vi "Oxford-1820-Main.vi"() -> ()   [LabVIEW 2016]
uses:
  <instrlib>/Mercury iXX/Mercury iXX.lvlib
  <instrlib>/Mercury iXX/Public/Controls/Comms Transport Layer.ctl
  <instrlib>/Mercury iXX/Public/Libraries/Pressure/Open/Open Pressure Device.vi
  <instrlib>/Mercury iXX/Public/Libraries/Pressure.lvlib
  <instrlib>/Mercury iXX/Public/Libraries/Pressure/Configuration/Read/Pressure Device (Read).vi
  <instrlib>/Mercury iXX/Public/Libraries/System/Read/Display Automatic Dimming (Read).vi
  <instrlib>/Mercury iXX/Public/Libraries/System.lvlib
  <instrlib>/Mercury iXX/Public/Libraries/System/Read/Display Automatic Dimming Time (Read).vi
  <instrlib>/Mercury iXX/Public/Libraries/System/Read/Display Brightness (Read).vi
  <instrlib>/Mercury iXX/Public/Libraries/System/Read/Mode (Read).vi
  <instrlib>/Mercury iXX/Public/Libraries/System/Read/Serial Number (Read).vi
  <instrlib>/Mercury iXX/Public/Libraries/System/Read/FVer (Read).vi
  <instrlib>/Mercury iXX/Public/Libraries/System/Read/HVer (Read).vi
  <instrlib>/Mercury iXX/Public/Libraries/System/Set/DateTime (Set).vi
  <instrlib>/Mercury iXX/Public/Libraries/Temperature/Signals/Read/Temperature (Read).vi
  <instrlib>/Mercury iXX/Public/Libraries/Temperature.lvlib
  <instrlib>/Mercury iXX/Public/Libraries/Temperature/Configuration/Read/Calibration Cold Limit (Read).vi
  <instrlib>/Mercury iXX/Public/Libraries/Temperature/Configuration/Read/Calibration Hot Limit (Read).vi
  <instrlib>/Mercury iXX/Public/Libraries/Temperature/Configuration/Read/Excitation Type (Read).vi
  <instrlib>/Mercury iXX/Public/Libraries/Temperature/Configuration/Read/Temperature Sensor (Read).vi
  <instrlib>/Mercury iXX/Public/Libraries/Temperature/Configuration/Read/Temperature Device (Read).vi
  <instrlib>/Mercury iXX/Public/Libraries/Temperature/Configuration/Read/Nickname (Read).vi
  <instrlib>/Mercury iXX/Public/Libraries/Temperature/Configuration/Read/Excitation Magnitude (Read).vi
  <instrlib>/Mercury iXX/Public/Libraries/Temperature/Configuration/Read/Serial Number (Read).vi
  <instrlib>/Mercury iXX/Public/Libraries/System/Read/Catalogue (Read).vi
  <instrlib>/Mercury iXX/Public/Libraries/System/Read/Flash Space (Read).vi
  <instrlib>/Mercury iXX/Public/Libraries/System/Read/DateTime (Read).vi
  <instrlib>/Mercury iXX/Public/Libraries/System/Read/Time (Read).vi
  <instrlib>/Mercury iXX/Public/Libraries/System/Read/Date (Read).vi
  <instrlib>/Mercury iXX/Public/Libraries/System/Open/Open System.vi
  <instrlib>/Mercury iXX/Public/Libraries/Temperature/Open/Open Temperature Device.vi
  <instrlib>/Mercury iXX/Public/Libraries/Auxiliary/Open/Open Auxiliary Device.vi
  <instrlib>/Mercury iXX/Public/Libraries/Auxiliary.lvlib
  <instrlib>/Mercury iXX/Public/Libraries/Auxiliary/Signals/Read/Percent Open (Read).vi
  <instrlib>/Mercury iXX/Public/Libraries/Magnet/Open/Open Magnet Device.vi
  <instrlib>/Mercury iXX/Public/Libraries/Magnet.lvlib
  <instrlib>/Mercury iXX/Public/Libraries/Magnet/Configuration/Read/PSU Action Status (Read).vi
  <instrlib>/Mercury iXX/Public/Libraries/Magnet/Configuration/Read/Magnet Device (Read).vi
  <instrlib>/Mercury iXX/Public/Libraries/Temperature/Signals/Read/Voltage (Read).vi
  <instrlib>/Mercury iXX/Private/Controls/Query Dynamic Reference.ctl
  <instrlib>/Mercury iXX/Public/Controls/Mercury Reference.ctl
  <instrlib>/Mercury iXX/Public/Libraries/Level Meter/Open/Open Level Meter Device.vi
  <instrlib>/Mercury iXX/Public/Libraries/Level Meter.lvlib
  <instrlib>/Mercury iXX/Public/Libraries/Level Meter/Signals/Read/Probe Level Nitrogen (Read).vi
  <instrlib>/Mercury iXX/Public/Libraries/Level Meter/Signals/Read/Probe Level Helium (Read).vi
  <instrlib>/Mercury iXX/Public/Libraries/Magnet/Signals/Read/Switch Heater Status (Read).vi
  <instrlib>/Mercury iXX/Public/Libraries/Magnet/Signals/Read/Current (Read).vi
  <instrlib>/Mercury iXX/Public/Libraries/Magnet/Configuration/Set/PSU Action Status (Set).vi
  <instrlib>/Mercury iXX/Public/Libraries/Magnet/Controls/PSU Actions.ctl
  <instrlib>/Mercury iXX/Public/Libraries/Magnet/Controls/Switch Heater.ctl
  SMOs/Instrument.Oxford1820/Instrument.Oxford1820.lvclass
  <instrlib>/Mercury iXX/Public/Libraries/Lambda/Configuration/Set/Lambda Percentage Flow (Set).vi
  <instrlib>/Mercury iXX/Public/Libraries/Lambda.lvlib
  <instrlib>/Mercury iXX/Public/Libraries/Lambda/Open/Open Lambda Device.vi
  <instrlib>/Mercury iXX/Public/Controls/Response String.ctl
  <instrlib>/Mercury iXX/Public/Libraries/Temperature/Signals/Read/Resistance (Read).vi
  <instrlib>/Mercury iXX/Public/Libraries/Temperature/Configuration/Set/Excitation Magnitude (Set).vi
  <instrlib>/Mercury iXX/Public/Libraries/Magnet/Signals/Read/Voltage (Read).vi
  SMOs/Instrument.Oxford1820/Typedefs/Status.ctl
  SMOs/Instrument.Oxford1820/Typedefs/Actions.ctl
  <instrlib>/Mercury iXX/Public/Libraries/System/Controls/User Mode.ctl
  <instrlib>/Mercury iXX/Public/Libraries/System/Set/Mode (Set).vi
  <instrlib>/Mercury iXX/Public/Libraries/Heater/Signals/Read/Power (Read).vi
  <instrlib>/Mercury iXX/Public/Libraries/Heater.lvlib
  <instrlib>/Mercury iXX/Public/Libraries/Heater/Signals/Read/Current (Read).vi
  <instrlib>/Mercury iXX/Public/Libraries/Auxiliary/Signals/Read/Position (Read).vi
  <instrlib>/Mercury iXX/Public/Libraries/Level Meter/Signals/Read/Probe Count Nitrogen (Read).vi
  <instrlib>/Mercury iXX/Public/Libraries/Magnet/Signals/Read/Current Rate (Read).vi
  <userlib>/_OpenG.lib/error/error.llb/Filter Error Codes (Array)__ogtk.vi
  <instrlib>/Mercury iXX/Public/Libraries/Heater/Configuration/Read/Nickname (Read).vi
  <instrlib>/Mercury iXX/Public/Libraries/Heater/Configuration/Read/Voltage Limit (Read).vi
  <instrlib>/Mercury iXX/Public/Libraries/Heater/Configuration/Read/Serial Number (Read).vi
  <instrlib>/Mercury iXX/Public/Libraries/Heater/Configuration/Read/Heater Device (Read).vi
  <instrlib>/Mercury iXX/Public/Libraries/Heater/Open/Open Heater Device.vi
  <instrlib>/Mercury iXX/Public/Libraries/Heater/Signals/Read/Voltage (Read).vi
  <instrlib>/Mercury iXX/Public/Libraries/Heater/Configuration/Read/Maximum Power (Read).vi
  <instrlib>/Mercury iXX/Public/Libraries/Heater/Configuration/Read/Nominal Resistance (Read).vi
  <instrlib>/Mercury iXX/Public/Libraries/Auxiliary/Configuration/Read/Stepper Speed (Read).vi
  <instrlib>/Mercury iXX/Public/Libraries/Auxiliary/Configuration/Read/Valve Gearing (Read).vi
  <instrlib>/Mercury iXX/Public/Libraries/Auxiliary/Configuration/Read/Temperature Error Voltage Sensitivity (Read).vi
  <instrlib>/Mercury iXX/Public/Libraries/Auxiliary/Configuration/Read/Temperature Error Sensitivity (Read).vi
  <instrlib>/Mercury iXX/Public/Libraries/Auxiliary/Configuration/Read/Gas Flow Scaling (Read).vi
  <instrlib>/Mercury iXX/Public/Libraries/Auxiliary/Configuration/Read/Minimum Gas Flow (Read).vi
  <instrlib>/Mercury iXX/Public/Libraries/Auxiliary/Configuration/Read/Serial Number (Read).vi
  <instrlib>/Mercury iXX/Public/Libraries/Auxiliary/Configuration/Read/Aux Device (Read).vi
  <instrlib>/Mercury iXX/Public/Libraries/Pressure/Signals/Read/Voltage (Read).vi
  <instrlib>/Mercury iXX/Public/Libraries/Pressure/Signals/Read/Current (Read).vi
  <instrlib>/Mercury iXX/Public/Libraries/Pressure/Configuration/Read/Nickname (Read).vi
  <instrlib>/Mercury iXX/Public/Libraries/Level Meter/Signals/Read/Probe Resistance Helium (Read).vi
  <instrlib>/Mercury iXX/Public/Libraries/Level Meter/Configuration/Read/Nitrogen Pulse Count Period (Read).vi
  <instrlib>/Mercury iXX/Public/Libraries/Level Meter/Configuration/Read/Nitrogen Freq at 100 (Read).vi
  <instrlib>/Mercury iXX/Public/Libraries/Level Meter/Configuration/Read/Helium Pulse Duration (Read).vi
  <instrlib>/Mercury iXX/Public/Libraries/Level Meter/Configuration/Read/Helium Pulse Mag (Read).vi
  <instrlib>/Mercury iXX/Public/Libraries/Level Meter/Configuration/Read/Helium Probe Resistance (Read).vi
  <instrlib>/Mercury iXX/Public/Libraries/Level Meter/Configuration/Read/Serial Number (Read).vi
  <instrlib>/Mercury iXX/Public/Libraries/Level Meter/Configuration/Read/Level Meter Device (Read).vi
  <instrlib>/Mercury iXX/Public/Libraries/Magnet/Configuration/Read/Software Voltage Limit (Read).vi
  <instrlib>/Mercury iXX/Public/Libraries/Magnet/Configuration/Read/Switch Present (Read).vi
  <instrlib>/Mercury iXX/Public/Libraries/Magnet/Configuration/Read/Current to Field Factor (Read).vi
  <instrlib>/Mercury iXX/Public/Libraries/Magnet/Configuration/Read/Current Limit (Read).vi
  <instrlib>/Mercury iXX/Public/Libraries/Magnet/Configuration/Read/Output Configuration (Read).vi
  <instrlib>/Mercury iXX/Public/Libraries/Magnet/Configuration/Read/Bipolar Output (Read).vi
  <instrlib>/Mercury iXX/Public/Libraries/Magnet/Configuration/Read/Serial Number (Read).vi
  <instrlib>/Mercury iXX/Public/Libraries/Magnet/Signals/Read/Target Field (Read).vi
  <instrlib>/Mercury iXX/Public/Libraries/Magnet/Signals/Read/Target Field Rate (Read).vi
  <instrlib>/Mercury iXX/Public/Libraries/Magnet/Signals/Read/Field (Read).vi
  <instrlib>/Mercury iXX/Public/Libraries/Magnet/Signals/Read/Persistant Field (Read).vi
  <instrlib>/Mercury iXX/Public/Libraries/Magnet/Configuration/Set/Switch Heater Current (Set).vi
  <instrlib>/Mercury iXX/Public/Libraries/Magnet/Signals/Read/Persistant Current (Read).vi
  <instrlib>/Mercury iXX/Public/Libraries/Magnet/Signals/Set/Switch Heater No Check (Set).vi
  <instrlib>/Mercury iXX/Public/Libraries/Magnet/Signals/Set/Target Field (Set).vi
  <instrlib>/Mercury iXX/Public/Libraries/Magnet/Signals/Set/Target Field Rate (Set).vi
  <instrlib>/Mercury iXX/Public/Libraries/Lambda/Configuration/Set/Lambda Flow Auto (Set).vi
  <instrlib>/Mercury iXX/Public/Libraries/Level Meter/Configuration/Set/Pulse Slow-Fast (Set).vi
  <instrlib>/Mercury iXX/Public/Libraries/Temperature/Controls/Excitation Type.ctl
  <instrlib>/Mercury iXX/Public/Controls/Manufacturing Data.ctl
  <instrlib>/Mercury iXX/Public/Libraries/Temperature/Controls/Excitation Cluster.ctl
  <instrlib>/Mercury iXX/Public/Libraries/Temperature/Controls/Calibration Interpolation.ctl
  <instrlib>/Mercury iXX/Public/Libraries/Temperature/Controls/Calibration Cluster.ctl
  <instrlib>/Mercury iXX/Public/Controls/Unit String.ctl
  <instrlib>/Mercury iXX/Public/Libraries/Heater/Controls/Heater Signals Cluster.ctl
  <instrlib>/Mercury iXX/Public/Libraries/Heater/Controls/Heater Device (Read).ctl
  <instrlib>/Mercury iXX/Public/Libraries/Level Meter/Controls/Resistance Configuration.ctl
  <instrlib>/Mercury iXX/Public/Libraries/Level Meter/Controls/Pre-Pulse.ctl
  <instrlib>/Mercury iXX/Public/Libraries/Level Meter/Controls/Pulse.ctl
  <instrlib>/Mercury iXX/Public/Libraries/Level Meter/Controls/Helium Configuration.ctl
  <instrlib>/Mercury iXX/Public/Libraries/Level Meter/Controls/Frequency Configuration.ctl
  <instrlib>/Mercury iXX/Public/Libraries/Level Meter/Controls/Nitrogen Configuration.ctl
  <instrlib>/Mercury iXX/Public/Libraries/Level Meter/Controls/Signals.ctl
  <instrlib>/Mercury iXX/Public/Libraries/Level Meter/Controls/Level Meter (Read).ctl
  <instrlib>/Mercury iXX/Public/Libraries/Auxiliary/Controls/AUX Signals (Read).ctl
  <instrlib>/Mercury iXX/Public/Libraries/Auxiliary/Controls/AUX Device (Read).ctl
  <instrlib>/Mercury iXX/Public/Libraries/Magnet/Controls/Signals (Read).ctl
  <instrlib>/Mercury iXX/Public/Libraries/Magnet/Controls/Device (Read).ctl
  <instrlib>/Mercury iXX/Public/Libraries/Magnet/Controls/Identifier.ctl
  <instrlib>/Mercury iXX/Public/Libraries/Pressure/Controls/Pressure Signals Cluster.ctl
panel:
  out "LPF ON":timestamp
  in  "Tab Control":T1(tab)
  in  "Enable RS232 Panel":bool
  out "LEDs":bool[](array[boolean])
  out "Iteration Time":dbl
  in  "Percentage Open":dbl=100.0 format="%#_13g"
  out "PS Heat on or off (sec)":dbl format="%<%H:%M:%S>t"
  out "LPF on (min)":dbl=5373.0 format="%<%H:%M:%S>t"
  out "Magnet Status 2":string
  in  "OK":bool
  out "LPF Resistance":dbl=4.2075 format="%_3f ohms"
  out "Magnet Resistance":dbl=3.8705 format="%_3f ohms"
  out "ETA":timestamp format="%<%I:%M:%S %p\n%m/%d/%y>T"
  in  "Open Needle Valve":bool
  in  "Close Needle Valve":bool
  in  "Lambda":bool
  out "LPF Pressure":dbl format="%_5f mB"
  out "LPF Needle Valve (%)":dbl format="%_6g"
  out "LPF Temperature":dbl=4.2075 format="%_2f K"
  out "Magnet Temperature":dbl=3.8705 format="%_2f K"
  out "He LVL Chart":dbl(slide)=52.0833 scale=0.0..100.0
  out "N2 LVL Chart":dbl(slide)=61.3025 scale=0.0..100.0
  in  "Remote Mode":bool
  out "Power Supply Field (T)":dbl=0.0001 format="%#.5f"
  out "Magnet Field (T)":dbl format="%.5f"
  out "Voltage (V)":dbl=-0.0003 format="%.5f"
  out "Current (A)":dbl=0.0006 format="%.5f"
  out "N2 LEVEL":dbl=61.3025 format="%.0f %"
  out "He LEVEL":dbl=52.0833 format="%.0f %"
  in  "Fast/Slow Fill":bool
  out "Magnet Field (T)":dbl(knob) caption="Voltage (V)" scale=-20.0..20.0
  out "SWITCH HEATER":bool
  in  "PS Heat":bool
  in  "Clamp":bool
  in  "To Set":bool
  in  "To Zero":bool
  in  "Hold":bool
  out "Magnet Status":string="Clamped"
  out "Target Field Rate (T/min)":dbl=1.0 format="%.5f"
  out "Target Field (T)":dbl format="%#.5f"
  in  "Target Rate (T/min)":dbl=0.1 format="%.5f"
  in  "Target Field (T)":dbl format="%#.5f"
  in  "Send to IPS":bool
  out "Voltage (V)":dbl(knob)=-0.0003 scale=-10.0..10.0
  out "Current (A)":dbl(knob)=0.0006 scale=-180.0..180.0
  in  "Mercury Functions":T2(tab)=enum."ITC: Temperature"
  out "time stamp":timestamp=timestamp(3543841780 s since 1904-01-01)
  out "Free Space":i32=166384 caption="Free Space (KB)"
  out "Set Date Response":string="VALID"
  out "String":string="NORM" caption="User Mode"
  out "Date":string="2016:04:18"
  out "Time":string="11:29:40"
  out "Hardware Version":string="65"
  out "Firmware Version":string="2.2.6.20"
  out "Serial Number":string="154650110"
  out "ITC Devices":string[](array[string])=["DB4.G1:AUX", "DB8.P1:PRES", "MB0.H1:HTR", "MB1.T1:TEMP"]
  out "S/W Version(s)":string[](array[string])=["2.2.6.20\n"]
  out "Serial Number(s)":string[](array[string])=["154650110"]
  out "# of Instruments":i32=1
  out "Automatic Dimming":string="OFF"
  out "Dimming Time":string="5"
  out "Display Brightness":string="100"
  in  "ITC IP Address":string="130.49.180.101"
  out "Excitation Magnitude":dbl=5.0
  out "Sensor Type":string="NTC"
  out "Excitation Type":string="UNIP"
  out "Hot Limit":dbl=1000.0
  out "H Unit":T3="K"
  out "Cold Limit":dbl=1000.0
  out "C Unit":T3="K"
  out "Unit":T3
  out "Voltage":dbl=0.005
  out "V Unit":T3="V"
  out "Temperature":dbl=4.2075
  out "T Unit":T3="K"
  out "Temp S/N":string="154650110"
  out "T Nickname":string="Mag_AB_MB1"
  out "ITC Calibration":T4
  out "ITC Excitation":T6
  out "ITC Manufacturing":T8
  out "Heater Device Settings":T9={"Manufacturing"={"Hardware Version"="65", "Firmware Version"="2.3", "Serial Number"="154650110"}, "Nickname"="MB0.H1", "Voltage Limit"="1", "Nominal Resistance"="10", "Maximum Power"="0.1000", "Heater Signals"={"Voltage"="0.0507V", "Current"="-0.0000A", "Power"="0.0000W"}, "Status"="2"}
  out "Htr C Unit":T3="A"
  out "Htr P Unit":T3="W"
  out "Htr V Unit":T3="V"
  out "Htr Current":dbl=-0.0
  out "Htr Power":dbl
  out "Htr Voltage":dbl=0.0507
  out "Power Unit":T3
  out "Volt Unit":T3
  out "Res Unit":T3
  out "Maximum Power":dbl=0.1
  out "Htr Resistance":dbl=10.0
  out "Htr Voltage Limit":dbl=1.0
  out "Htr S/N":string="154650110"
  out "Htr Nickname":string="MB0.H1"
  out "Nickname":string="Lam_P_DB8"
  out "Current":dbl=-0.0
  out "Voltage":dbl=-8.219999999999999e-05
  out "Manufacturing":T8
  out "Pressure Signals":T11
  out "Auxiliary Device Details":T12={"Manufacturing"={"Hardware Version"="65", "Firmware Version"="3.1", "Serial Number"="154650084"}, "Min Flow"=0.0, "Scaling Factor"=50.0, "Temp Err"=9.0, "Temp V Err"=11.0, "Gear"=2, "Speed"=2, "Signals"={"Position"=0.0, "% Open"=0.0, "I0"="ON", "I1"="OFF", "I2"="OFF", "I3"="OFF", "O0"="OFF", "O1"="OFF", "O2"="OFF", "O3"="OFF"}, "Nickname"="DB4.G1", "Status"="0"} {"Signals"."% Open" min=0.0 max=100.0 step=0.1 format="%.4f"; "Signals"."Position" max=20.0 step=1.0 format="%.4f"; "Speed" max=7 step=1; "Gear" max=7 step=1; "Temp V Err" min=0.0 max=20.0 step=0.1; "Temp Err" min=0.0 max=20.0 step=0.1; "Scaling Factor" min=0.0 max=99.0 step=0.1; "Min Flow" min=0.0 max=20.0 step=0.1}
  out "Aux S/N":string="154650084"
  out "Min Flow":dbl caption="Minimum Gas Flow" format="%#.1f"
  out "Scaling Factor":dbl=50.0 caption="Gas Flow Scaling Factor" format="%#.1f"
  out "Temp Err":dbl=9.0 caption="Temperature Error Sensitivity" format="%#.1f"
  out "Temp V Err":dbl=11.0 caption="Temperature Voltage Error Sensitivity" format="%#.1f"
  out "Gear":u32=2 caption="Valve Gearing"
  out "Speed":u32=2 caption="Stepper Speed"
  out "Unit 2":T3
  out "Unit 3":T3
  out "Unit 4":T3
  out "Unit 5":T3
  out "Unit 6":T3
  out "Unit 7":T3
  out "Position":u32
  out "% Open":dbl caption="Percentage Open (%)"
  out "Unit":T3
  out "Unit":T3="%"
  out "time stamp 2":timestamp=timestamp(3543841781 s since 1904-01-01)
  out "Free Space 2":i32=166316 caption="Free Space (KB)"
  out "Set Date Response 2":string="VALID"
  out "String 2":string="NORM" caption="User Mode"
  out "Date 2":string="2016:04:18"
  out "Time 2":string="11:29:45"
  out "Hardware Version 2":string="65"
  out "Firmware Version 2":string="2.2.6.20"
  out "Serial Number 2":string="153350063"
  out "IPS Devices":string[](array[string])=["DB3.L1:LVL", "GRPX:PSU", "GRPY:PSU", "GRPZ:PSU", "MB1.T1:TEMP", "PSU.M1:PSU", "PSU.M2:PSU", "PSU.M3:PSU"]
  out "S/W Version(s) 2":string[](array[string])=["2.2.6.20\n"]
  out "Serial Number(s) 2":string[](array[string])=["153350063"]
  out "# of Instruments 2":i32=1
  out "Automatic Dimming 2":string="OFF"
  out "Dimming Time 2":string="5"
  out "Display Brightness 2":string="100"
  in  "IPS IP Address":string="130.49.180.102"
  out "LVL Device DetailSettings":T14={"Manufacturing"={"Hardware Version"="65", "Firmware Version"="2.2", "Serial Number"="152450013"}, "Nitrogen Configuration"={"Frequency Configuration"={"Freq 0%"=0.0, "Freq 100%"=0.0}, "Pulse Period"=0.0}, "Signals"={"Helium Signals"={"Resistance"=75.5626, "Level"=52.0833}, "Nitrogen Signals"={"Count"=8800.0, "Freq"=487361.0, "Level"=61.3445}}, "Nickname"="DB3.L1", "Status"="0", "Helium Configuration"={"Resistance Configuration"={"Res 0%"=0.0, "Res 100%"=0.0}, "Pre-Pulse"={"Magnitude"=0.0, "Duration"=0.0}, "Pulse"={"Magnitude"=0.0, "Duration"=0.0, "Delay"=0.0}}}
  out "LVL S/N":string="152450013"
  out "LVL P Magnitude":dbl=125.0 caption="Pulse Magnitude (mA)"
  out "LVL P Duration":dbl=5.0 caption="Pulse Duration (s)"
  out "N Freq 100%":dbl=7880.0 caption="Frequency at 100% (Hz)"
  out "N Pulse Period":dbl=1000.0 caption="Pulse Period (ms)"
  out "He Res Config":T19={"Res 0%"=149.0, "Res 100%"=8.0}
  out "He Resistance":dbl=75.5626 caption="Resistance (Ohms)"
  out "He Level":dbl=52.0833 caption="Helium Level (%)"
  out "N Counter":u32 caption="Counter"
  out "N Level":dbl=61.3445 caption="Nitrogen Level (%)"
  out "Excitation Magnitude 2":dbl=5.0
  out "Sensor Type 2":string="NTC"
  out "Excitation Type 2":string="UNIP"
  out "Hot Limit 2":dbl=1000.0
  out "H Unit 2":T3="K"
  out "Cold Limit 2":dbl=1000.0
  out "C Unit 2":T3="K"
  out "Unit 12":T3
  out "Voltage 2":dbl=0.005
  out "V Unit 2":T3="V"
  out "Temperature 2":dbl=3.8706
  out "T Unit 2":T3="K"
  out "Temp S/N 2":string="153350063"
  out "T Nickname 2":string="MB1.T1"
  out "IPS Calibration":T4
  out "IPS Excitation":T6
  out "IPS Manufacturing":T8
  out "Magnet Device Details":T22={"Manufacturing"={"Hardware Version"="NOT_FOUND", "Firmware Version"="NOT_FOUND", "Serial Number"="NOT_FOUND"}, "Nickname"="GRPZ", "Bipolar Output"="ON", "String"="PARA", "Current Limit"=174.0, "AtoB"=8.688, "Inductance"=39.406, "Switch Present"="PSU.M1", "Swh Htr Current"=86.0, "SW VLIM"=9.0, "V Trans Time"=1000.0, "Magnet PSU Signals"={"Voltage"=-0.0002, "Current"=0.0002, "Current Rate"=100.0, "Field"=0.0001, "Field Rate"=11.5101, "Persistant Current"=0.0003, "Persistant Field"=0.0, "Target Current"=0.0, "Target Field"=0.0, "Target Current Rate"=8.688, "Target Field Rate"=1.0, "Switch Heater Status (SWHT)"="OFF", "Switch Heater Status (SWHN)"="OFF"}, "PSU Action"="CLMP", "Status"="40000000", "Level Limit"=0.0, "Temperature Limit"=999.0} {"Temperature Limit" format="%#.1f"; "Level Limit" format="%#.1f"; "V Trans Time" format="%#.1f"; "SW VLIM" format="%#.1f"; "Swh Htr Current" format="%#.1f"; "Inductance" format="%#.1f"; "AtoB" format="%#.1f"; "Current Limit" format="%#.1f"}
  out "Mag S/N":string="NOT_FOUND"
  out "Bipolar Output":string="ON"
  out "Out Config":string="PARA" caption="Output Configuration"
  out "Current Limit":dbl=174.0 caption="Current Limit (A)" format="%#.1f"
  out "AtoB":dbl=8.688 caption="Current Field Factor (A/T)" format="%#.1f"
  out "Switch Present":string="PSU.M1"
  out "SW VLIM":dbl=9.0 caption="Software Voltage Limit (V)" format="%#.1f"
  out "Unit 8":T3
  out "Unit 9":T3
  out "Unit 10":T3
  out "Current Rate":dbl=100.0
  out "PSU Act Stat":string="CLMP" caption="PSU Action Status"
  out "Unit 11":T3="A/min"
  in  "Device Identifier":T24="GRPZ"
  out "M3 Voltage":dbl
  out "M3 Current":dbl
  out "M2 Voltage":dbl
  out "M2 Current":dbl
  out "M1 Voltage":dbl
  out "M1 Current":dbl
  out "Error List":T25(array[cluster])
  out "PS ON/OFF":timestamp format="%<%I:%M:%S %p>T"
  in  "Heater Current":bool
  in  "Swh Htr Current (mA)":dbl=90.0 format="%#_13g"
  # "v2017/10/10"
  # "Voltage (V)"
  # "Magnet (T)"
  # "Current (A)"
  # "Slow Rates\nCurrent Range (A)     Field Range (T)    Rate (T/min)\n0       -- 100        0    -- 11.5       0.91\n100     -- 150        11.5 -- 17.2       0.23\n150     -- 155.467    17.2 -- 18         0.11\n155.567 -- 172.471    18   -- 20         0.11"
  # "Fast Rates\nCurrent Range (A)     Field Range (T)    Rate (T/min)\n0       -- 155.467    0    -- 18         1.0\n155.567 -- 172.471    18   -- 20         0.25"
  # "ITC: 101\nIPS: 102\nIPS VR: 67"
  # "ITC: 101\nIPS: 102\nIPS VR: 67"
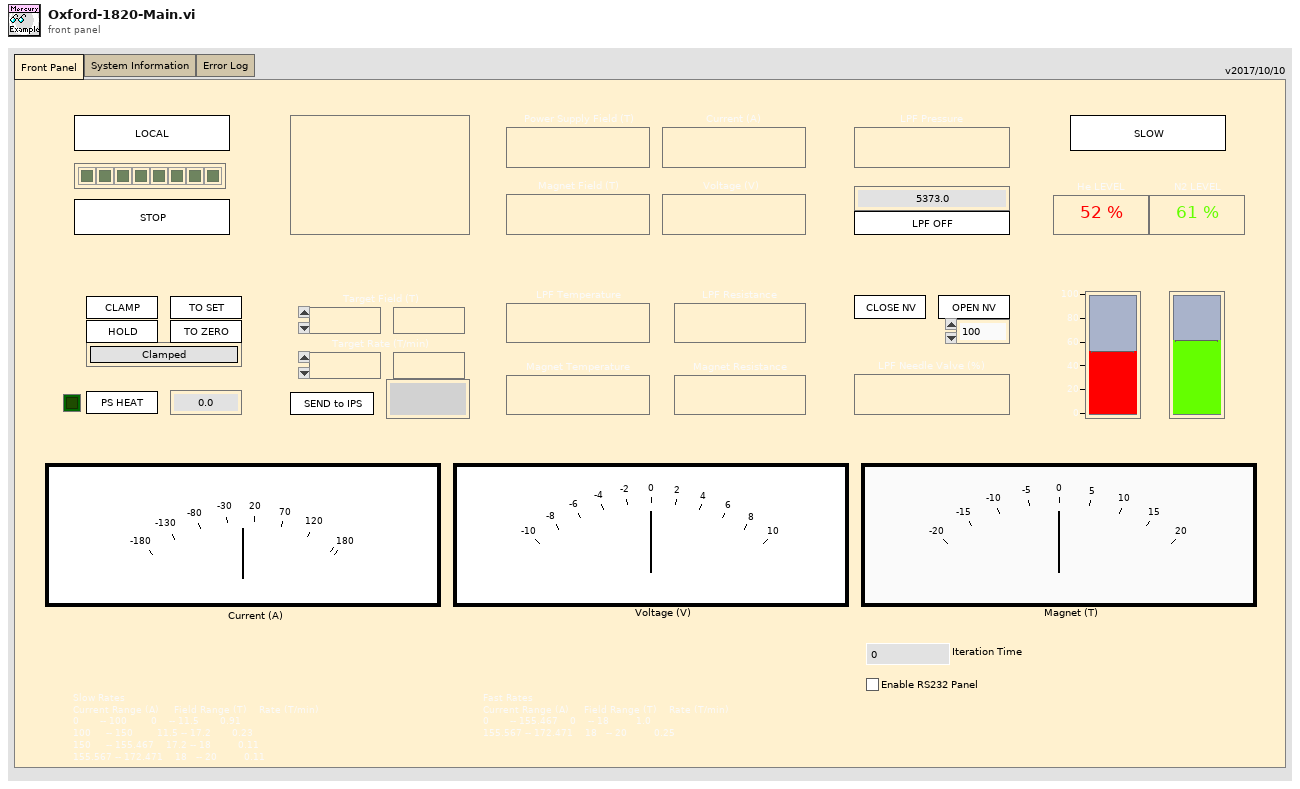
[diagram p1: front panel]
types:
  T1 = enum32{"Front Panel", "System Information", "Error Log"}
  T2 = enum32{"ITC: System", "ITC: Temperature", "ITC: Heater", "ITC: Pressure", "ITC: Auxiliary", "IPS: System", "IPS: Level Meter", "IPS: Temperature", "IPS: Magnet"}
  T3 = typedef "Mercury iXX.lvlib/Unit String.ctl" = string
  T4 = typedef "Mercury iXX.lvlib/Temperature.lvlib/Calibration Cluster.ctl" = cluster{"Filename":string, "Interpolation":T5, "Scaling Factor":string, "Offset Factor":string, "Hot Limit":string, "Cold Limit":string, "Last Calibration":string, "Reference":string}
  T5 = typedef "Mercury iXX.lvlib/Temperature.lvlib/Calibration Interpolation.ctl" = string
  T6 = typedef "Mercury iXX.lvlib/Temperature.lvlib/Excitation Cluster.ctl" = cluster{"Excitation Type":T7, "Magnitude":string}
  T7 = typedef "Mercury iXX.lvlib/Temperature.lvlib/Excitation Type.ctl" = string
  T8 = typedef "Mercury iXX.lvlib/Manufacturing Data.ctl" = cluster{"Hardware Version":string, "Firmware Version":string, "Serial Number":string}
  T9 = typedef "Mercury iXX.lvlib/Heater.lvlib/Heater Device (Read).ctl" = cluster{"Manufacturing":T8, "Nickname":string, "Voltage Limit":string, "Nominal Resistance":string, "Maximum Power":string, "Heater Signals":T10, "Status":string}
  T10 = typedef "Mercury iXX.lvlib/Heater.lvlib/Heater Signals Cluster.ctl" = cluster{"Voltage":string, "Current":string, "Power":string}
  T11 = typedef "Mercury iXX.lvlib/Pressure.lvlib/Pressure Signals Cluster.ctl" = cluster{"Voltage":string, "Current":string, "Power":string, "Pressure":string}
  T12 = typedef "Mercury iXX.lvlib/Auxiliary.lvlib/AUX Device (Read).ctl" = cluster{"Manufacturing":T8, "Min Flow":dbl, "Scaling Factor":dbl, "Temp Err":dbl, "Temp V Err":dbl, "Gear":u32, "Speed":u32, "Signals":T13, "Nickname":string, "Status":string}
  T13 = typedef "Mercury iXX.lvlib/Auxiliary.lvlib/AUX Signals (Read).ctl" = cluster{"Position":dbl, "% Open":dbl, "I0":string, "I1":string, "I2":string, "I3":string, "O0":string, "O1":string, "O2":string, "O3":string}
  T14 = typedef "Mercury iXX.lvlib/Level Meter.lvlib/Level Meter (Read).ctl" = cluster{"Manufacturing":T8, "Nitrogen Configuration":T15, "Signals":T17, "Nickname":string, "Status":string, "Helium Configuration":T18}
  T15 = typedef "Mercury iXX.lvlib/Level Meter.lvlib/Nitrogen Configuration.ctl" = cluster{"Frequency Configuration":T16, "Pulse Period":dbl}
  T16 = typedef "Mercury iXX.lvlib/Level Meter.lvlib/Frequency Configuration.ctl" = cluster{"Freq 0%":dbl, "Freq 100%":dbl}
  T17 = typedef "Mercury iXX.lvlib/Level Meter.lvlib/Signals.ctl" = cluster{"Helium Signals":cluster{"Resistance":dbl, "Level":dbl}, "Nitrogen Signals":cluster{"Count":dbl, "Freq":dbl, "Level":dbl}}
  T18 = typedef "Mercury iXX.lvlib/Level Meter.lvlib/Helium Configuration.ctl" = cluster{"Resistance Configuration":T19, "Pre-Pulse":T20, "Pulse":T21}
  T19 = typedef "Mercury iXX.lvlib/Level Meter.lvlib/Resistance Configuration.ctl" = cluster{"Res 0%":dbl, "Res 100%":dbl}
  T20 = typedef "Mercury iXX.lvlib/Level Meter.lvlib/Pre-Pulse.ctl" = cluster{"Magnitude":dbl, "Duration":dbl}
  T21 = typedef "Mercury iXX.lvlib/Level Meter.lvlib/Pulse.ctl" = cluster{"Magnitude":dbl, "Duration":dbl, "Delay":dbl}
  T22 = typedef "Mercury iXX.lvlib/Magnet.lvlib/Device (Read).ctl" = cluster{"Manufacturing":T8, "Nickname":string, "Bipolar Output":string, "String":string, "Current Limit":dbl, "AtoB":dbl, "Inductance":dbl, "Switch Present":string, "Swh Htr Current":dbl, "SW VLIM":dbl, "V Trans Time":dbl, "Magnet PSU Signals":T23, "PSU Action":string, "Status":string, "Level Limit":dbl, "Temperature Limit":dbl}
  T23 = typedef "Mercury iXX.lvlib/Magnet.lvlib/Signals (Read).ctl" = cluster{"Voltage":dbl, "Current":dbl, "Current Rate":dbl, "Field":dbl, "Field Rate":dbl, "Persistant Current":dbl, "Persistant Field":dbl, "Target Current":dbl, "Target Field":dbl, "Target Current Rate":dbl, "Target Field Rate":dbl, "Switch Heater Status (SWHT)":string, "Switch Heater Status (SWHN)":string}
  T24 = typedef "Mercury iXX.lvlib/Magnet.lvlib/Identifier.ctl" = string
  T25 = cluster{"time":timestamp, "code":i32, "source":string}[]
  T26 = enum32{"invalid app kind", "Development System", "Run Time System", "Student Edition", "Embedded LabVIEW", "Evaluation", "Custom"}
  T27 = cluster{"time":timestamp, "code":i32, "source":string}
  T28 = enum32{"Invalid", "Standard", "Closed", "Hidden", "Minimized", "Maximized"}
  T29 = typedef "Instrument.Oxford1820.lvclass/Status.ctl" = cluster{"Magnet Field":dbl, "PS Field":dbl, "Target Field":dbl, "Target Field Rate":dbl, "Voltage":dbl, "Current":dbl, "Switch":bool, "Mercury State":string}
  T30 = cluster{"Magnet Field":dbl, "PS Field":dbl, "Target Field":dbl, "Target Field Rate":dbl, "Voltage":dbl, "Current":dbl}
  T31 = typedef "Instrument.Oxford1820.lvclass/Actions.ctl" = cluster{"Hold":bool, "Clamp":bool, "To Set":bool, "To Zero":bool, "Send to IPS":bool, "PS Heat":bool, "Lambda":bool}
  T32 = typedef "Mercury iXX.lvlib/System.lvlib/User Mode.ctl" = string
  T33 = typedef "Mercury iXX.lvlib/Magnet.lvlib/Switch Heater.ctl" = string
  T34 = typedef "Mercury iXX.lvlib/Response String.ctl" = string
  T35 = typedef "Mercury iXX.lvlib/Mercury Reference.ctl" = cluster{"Comms":refnum<visa-resource-name>, "Device ID":string[], "Comms Layer":T36, "Command":string, "Query reference":T37}
  T36 = typedef "Mercury iXX.lvlib/Comms Transport Layer.ctl" = enum16{"Ethernet TCP/IP", "USB", "ISOBus - RS-232", "GPIB"}
  T37 = typedef "Mercury iXX.lvlib/Query Dynamic Reference.ctl" = refnum<vi>
  T38 = cluster{"Core":cluster{"Current VI Reference":refnum<vi>, "Close Panel on Exit?":bool}, "Mercury ITC Ref":T35, "Mercury IPS Ref":T35, "sentinel":bool, "Error Log":cluster{"time":timestamp, "code":i32, "source":string}[], "read ITC T?":bool, "counter":i32, "LEDs":bool[]}
  T39 = typedef "Filtered Error Details - Cluster__ogtk.ctl" = cluster{"code":i32, "source":string}
  T40 = cluster{"Current VI Reference":refnum<vi>, "Close Panel on Exit?":bool}
  T41 = typedef "Mercury iXX.lvlib/Temperature.lvlib/Temperature Sensor Type.ctl" = string
  T42 = typedef "Mercury iXX.lvlib/Temperature.lvlib/Temperature Device (Read).ctl" = cluster{"Manufacturing":T8, "Temperature Sensor Type":T41, "Excitation":T6, "Calibration":T4, "Control Loop":T43, "Temperature Signals":T44, "Nickname":string, "Status":string}
  T43 = typedef "Mercury iXX.lvlib/Temperature.lvlib/Loop Cluster.ctl" = cluster{"Heater":string, "Auxiliary":string, "Heater Auto":string, "Percentage Heat":string, "Temperature Set Point":string, "PID Auto (from file)":string, "P Value":string, "I Value":string, "D Value":string, "Auto PID Table Filename":string, "Flow Auto":string, "Target Heater Table":string, "Sweep mode":string, "Sweep Table Filename":string, "Percentage Flow":string}
  T44 = typedef "Mercury iXX.lvlib/Temperature.lvlib/Temperature Signals Cluster.ctl" = cluster{"Voltage":string, "Current":string, "Power":string, "Resistance":string, "Temperature":string, "Sensitivity":string, "Reference":string}
  T45 = typedef "Mercury iXX.lvlib/Pressure.lvlib/Pressure Device (Read).ctl" = cluster{"Manufacturing":T8, "Temperature Sensor Type":T46, "Calibration":T47, "Control Loop":T49, "Pressure Signals":T11, "Nickname":string, "Status":string}
  T46 = typedef "Mercury iXX.lvlib/Pressure.lvlib/Pressure Sensor Type.ctl" = string
  T47 = typedef "Mercury iXX.lvlib/Pressure.lvlib/Calibration Cluster.ctl" = cluster{"Filename":string, "Interpolation":T48, "Scaling Factor":string, "Offset Factor":string, "High Limit":string, "Low Limit":string, "Last Calibration":string}
  T48 = typedef "Mercury iXX.lvlib/Pressure.lvlib/Calibration Interpolation.ctl" = string
  T49 = typedef "Mercury iXX.lvlib/Pressure.lvlib/Loop Cluster.ctl" = cluster{"Heater":string, "Auxiliary":string, "Heater Auto":string, "Percentage Heat":string, "Pressure Set Point":string, "PID Auto (from file)":string, "P Value":string, "I Value":string, "D Value":string, "Auto PID Table Filename":string, "Flow Auto":string, "Target Heater Table":string, "Sweep mode":string, "Sweep Table Filename":string, "Percentage Flow":string}
  T50 = typedef "Mercury iXX.lvlib/Magnet.lvlib/Output Configuration.ctl" = string
  T51 = typedef "Mercury iXX.lvlib/Magnet.lvlib/PSU Actions.ctl" = string
  T52 = typedef "Instrument.Oxford1820.lvclass/Targets.ctl" = cluster{"Field (T)":dbl, "Field Rate (T/min)":dbl}
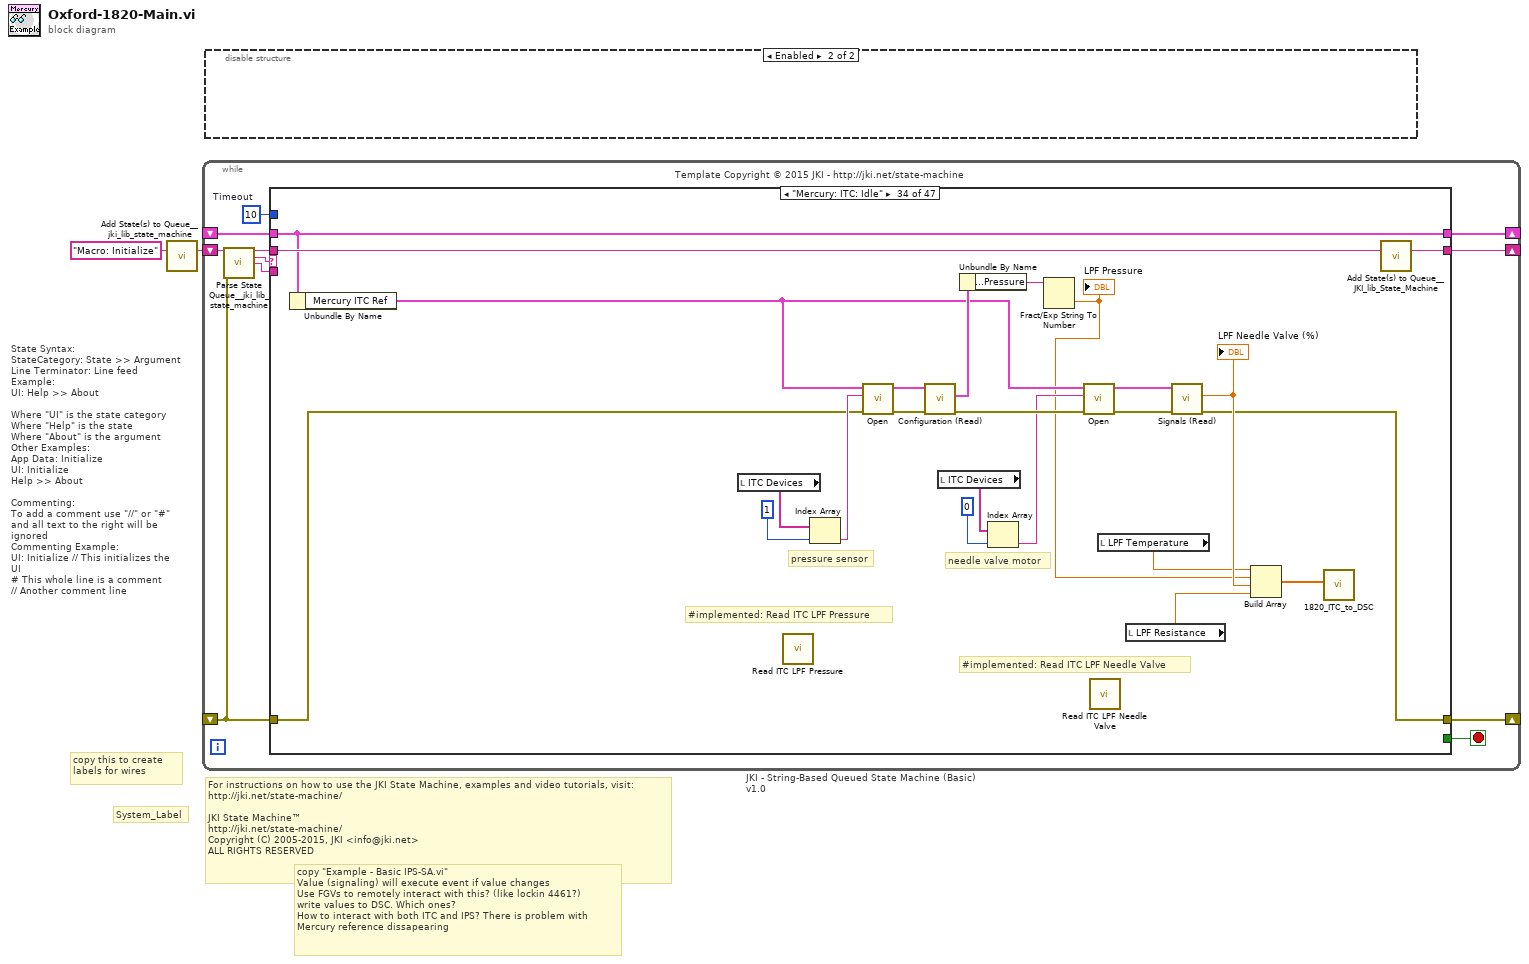
[diagram p0: block diagram]
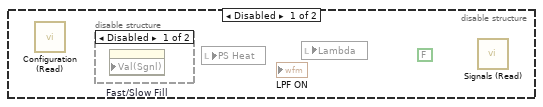
[diagram p2: hidden frame]
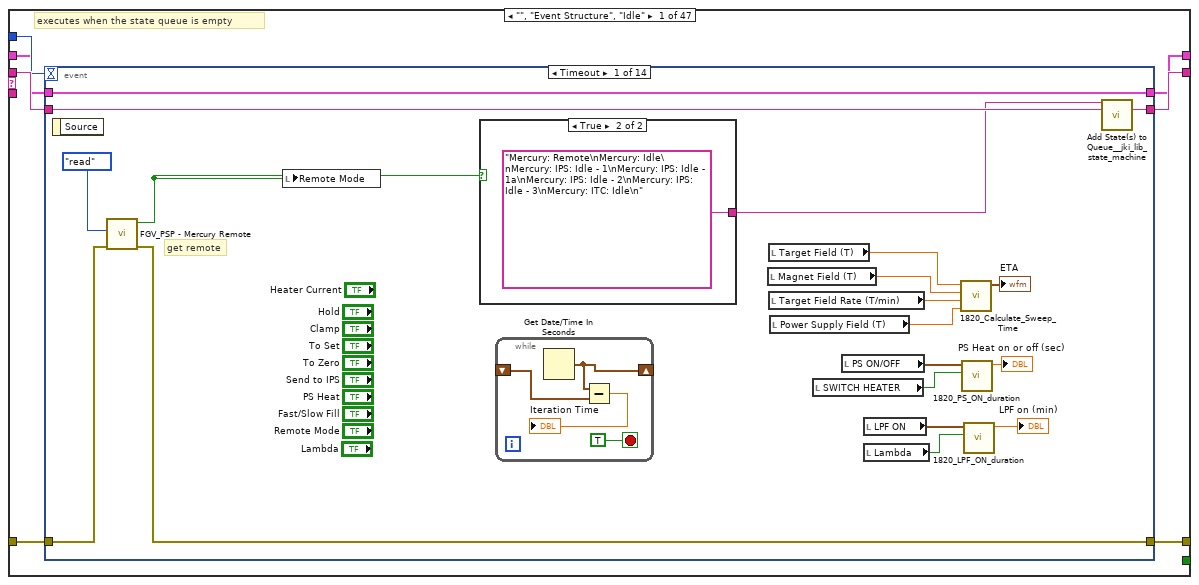
[diagram p4: hidden frame]
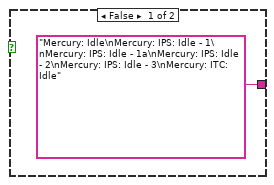
[diagram p5: hidden frame]
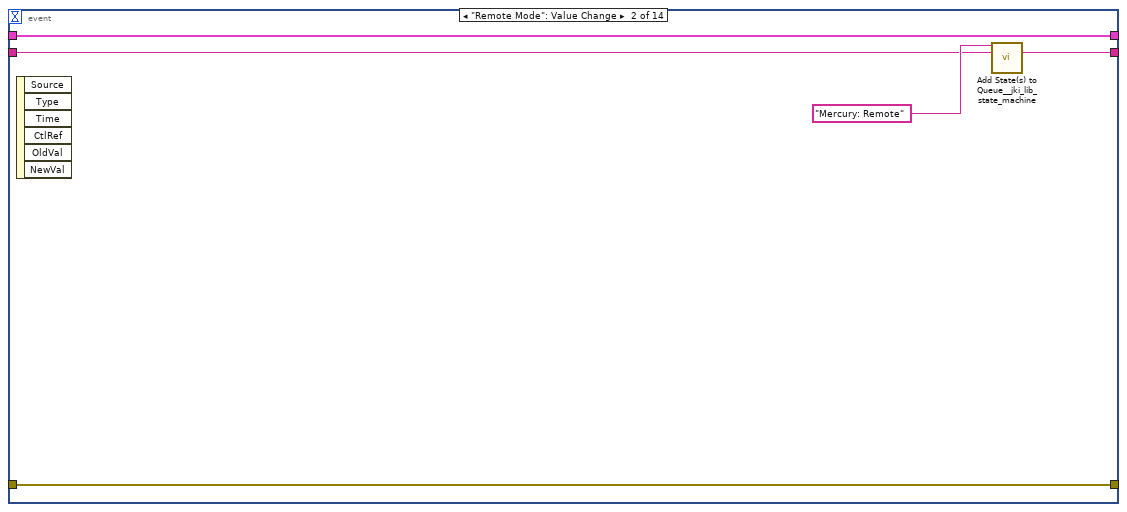
[diagram p6: hidden frame]
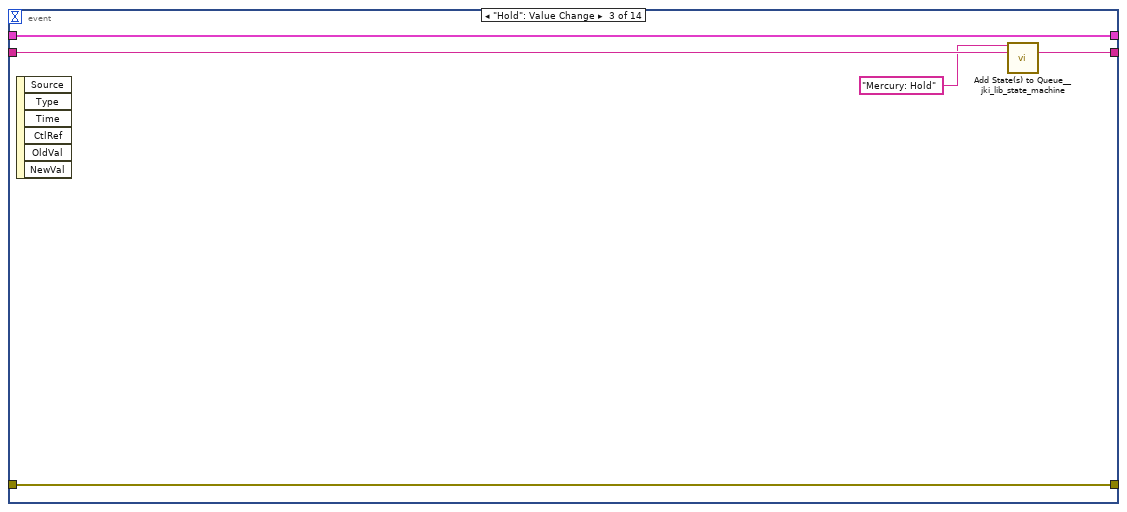
[diagram p7: hidden frame]
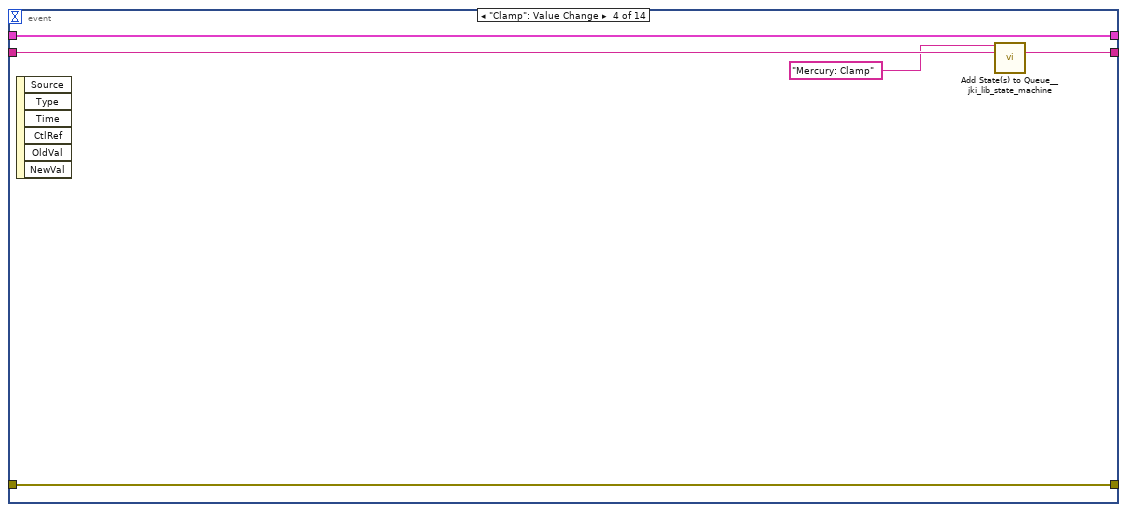
[diagram p8: hidden frame]
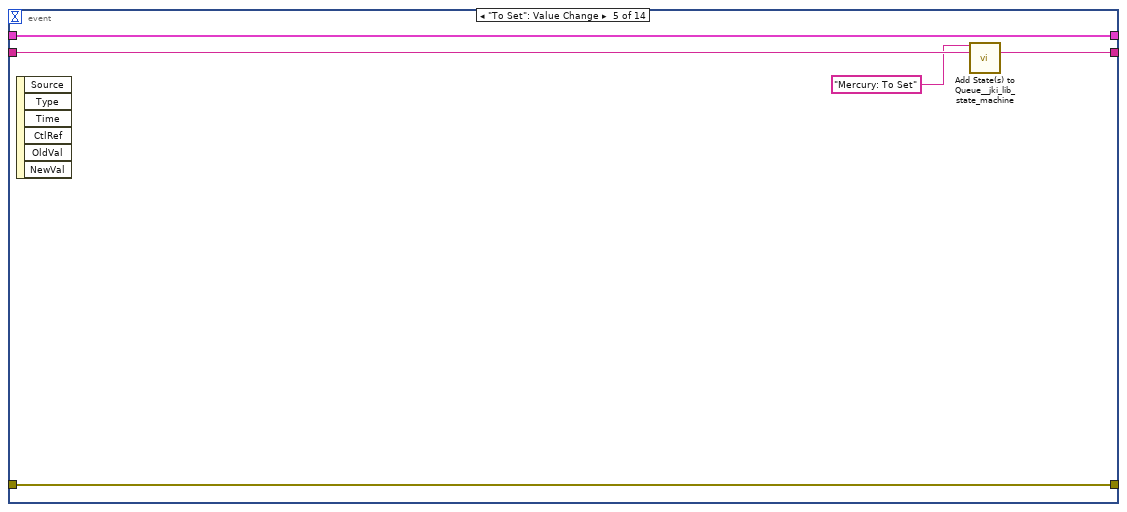
[diagram p9: hidden frame]
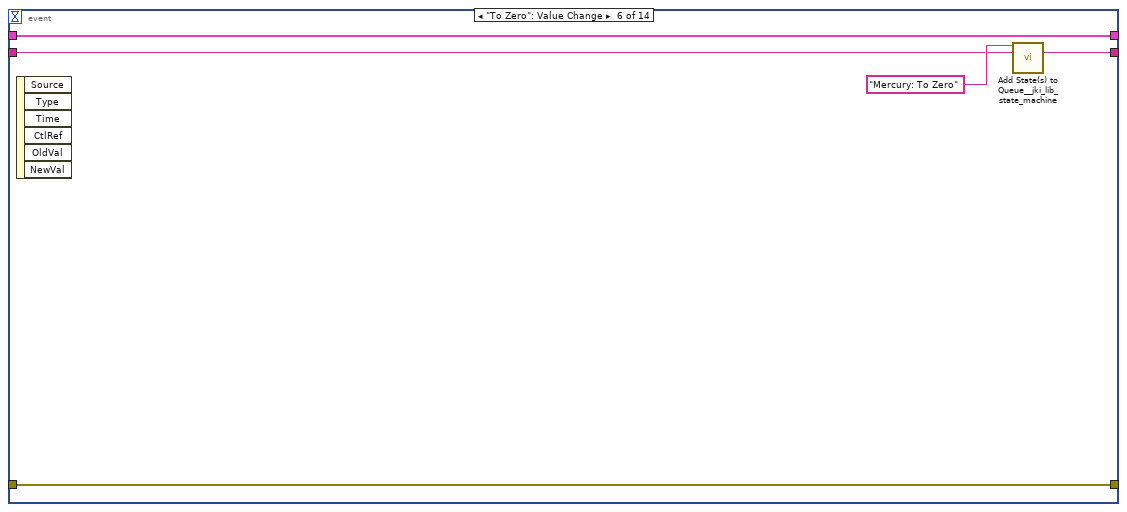
[diagram p10: hidden frame]
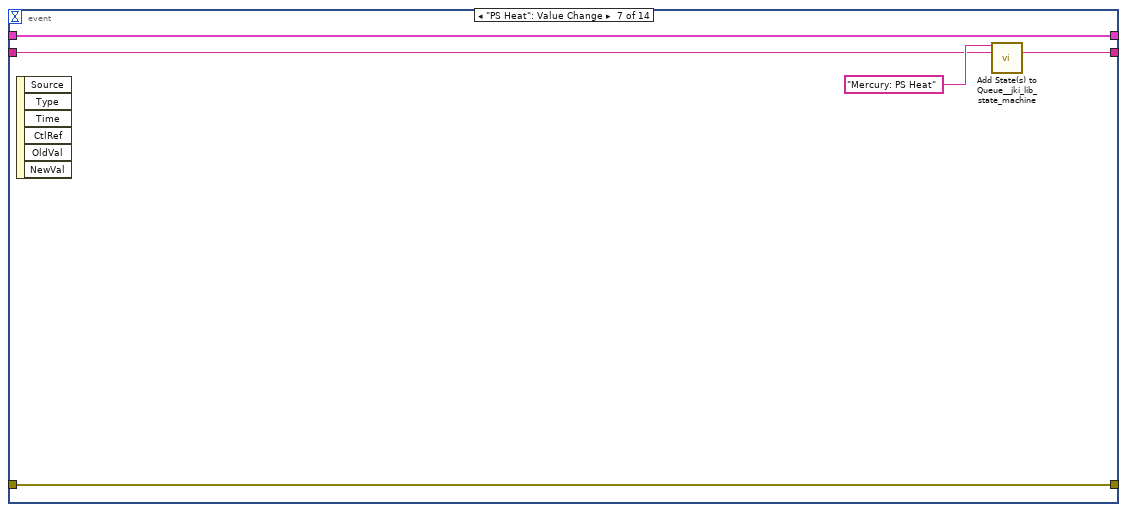
[diagram p11: hidden frame]
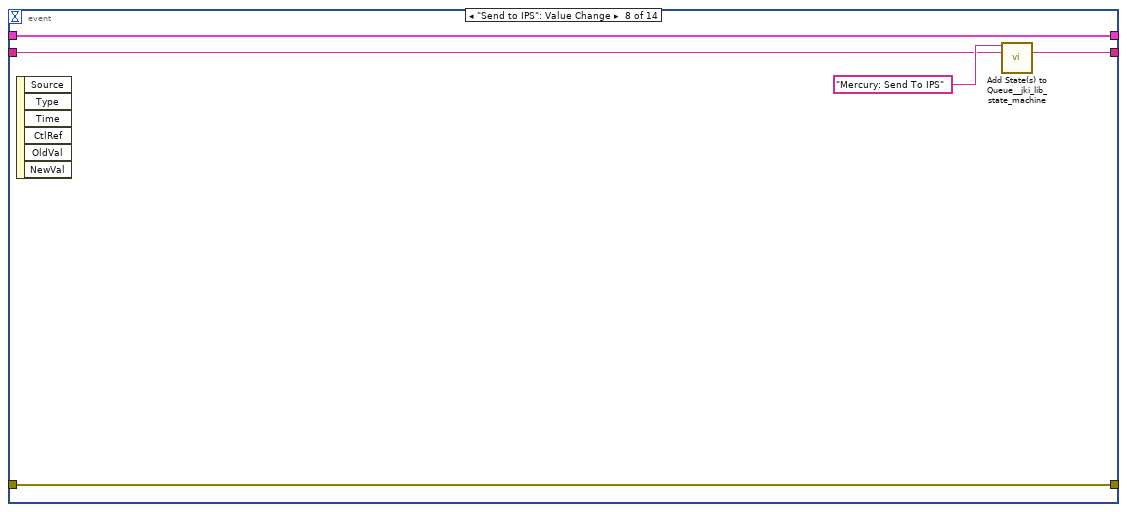
[diagram p12: hidden frame]
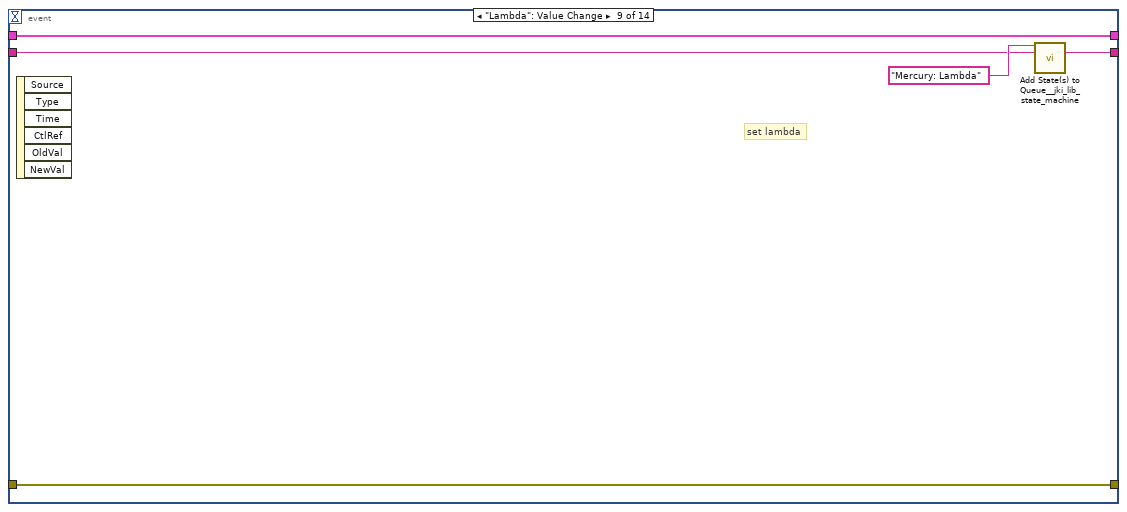
[diagram p13: hidden frame]
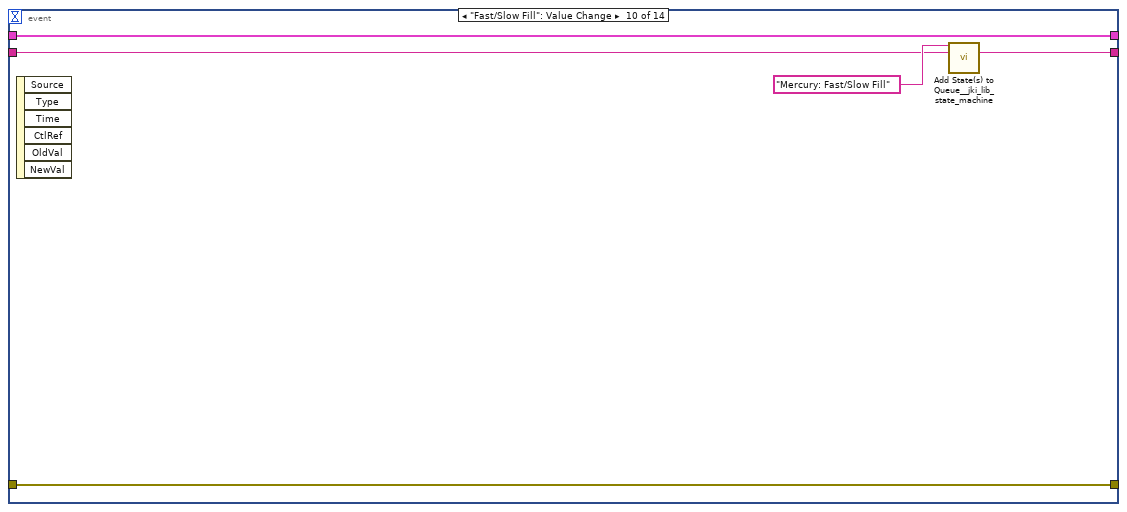
[diagram p14: hidden frame]
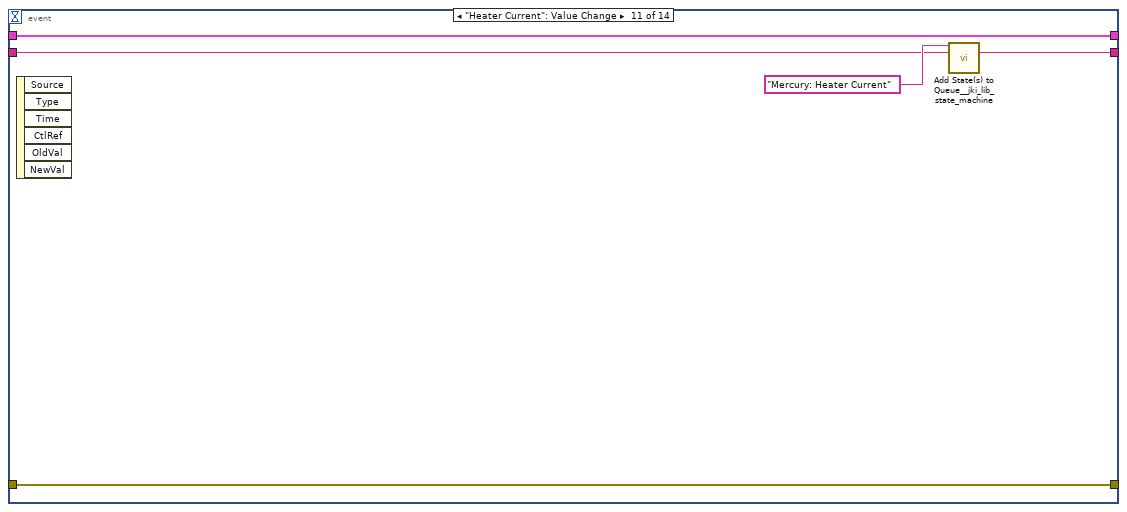
[diagram p15: hidden frame]
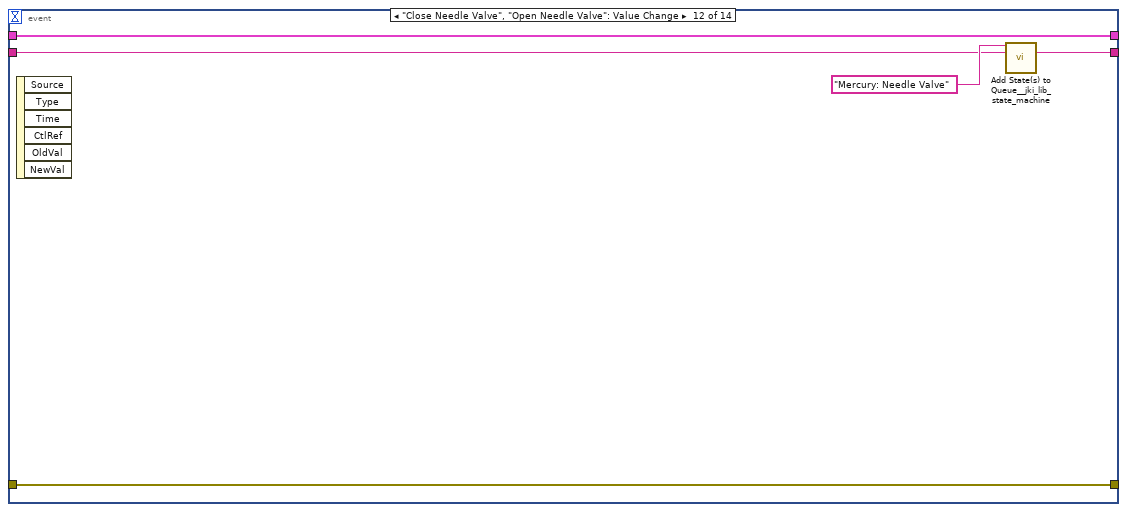
[diagram p16: hidden frame]
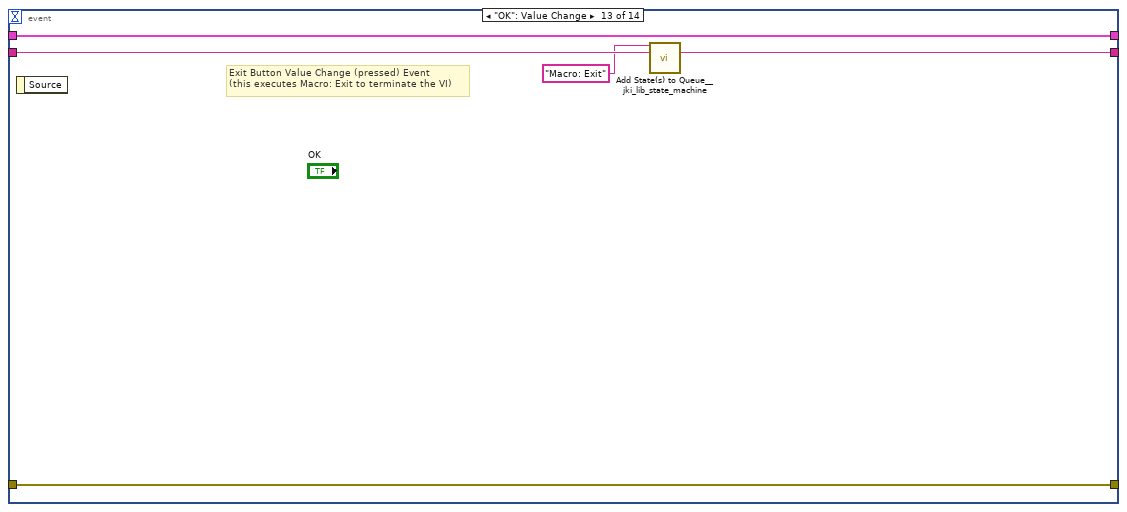
[diagram p17: hidden frame]
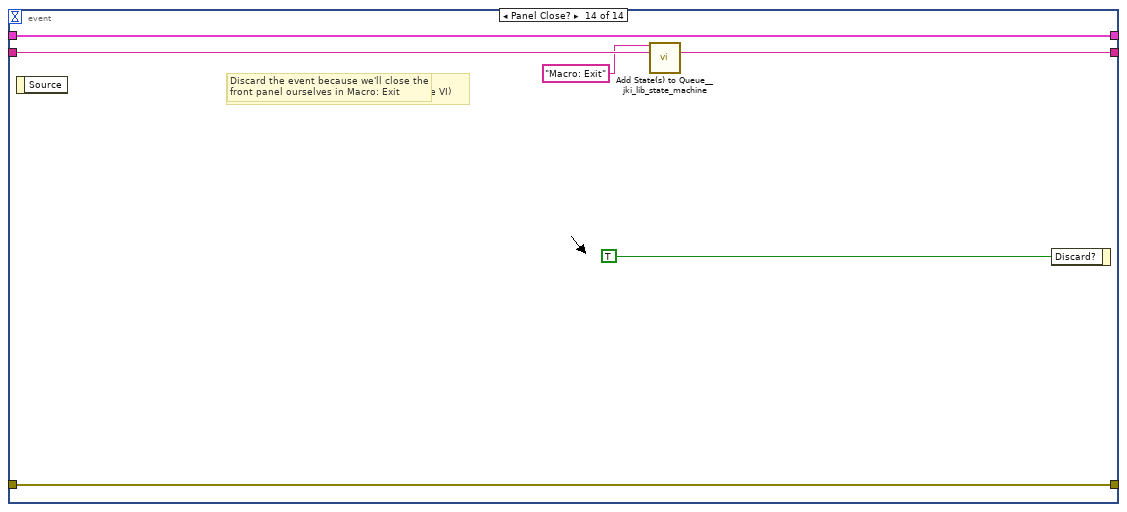
[diagram p18: hidden frame]
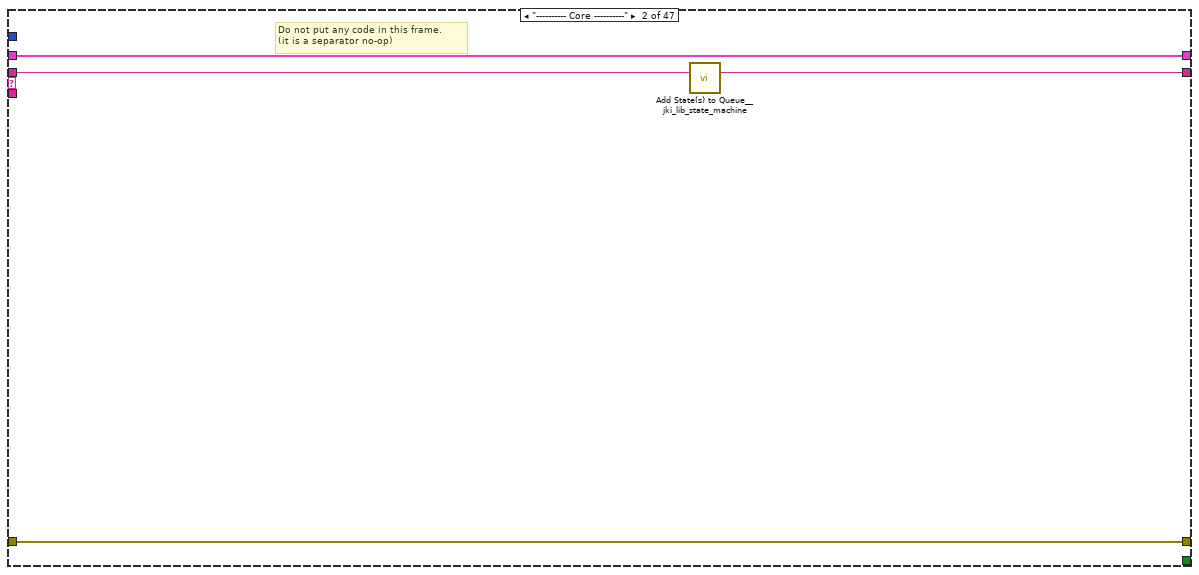
[diagram p19: hidden frame]
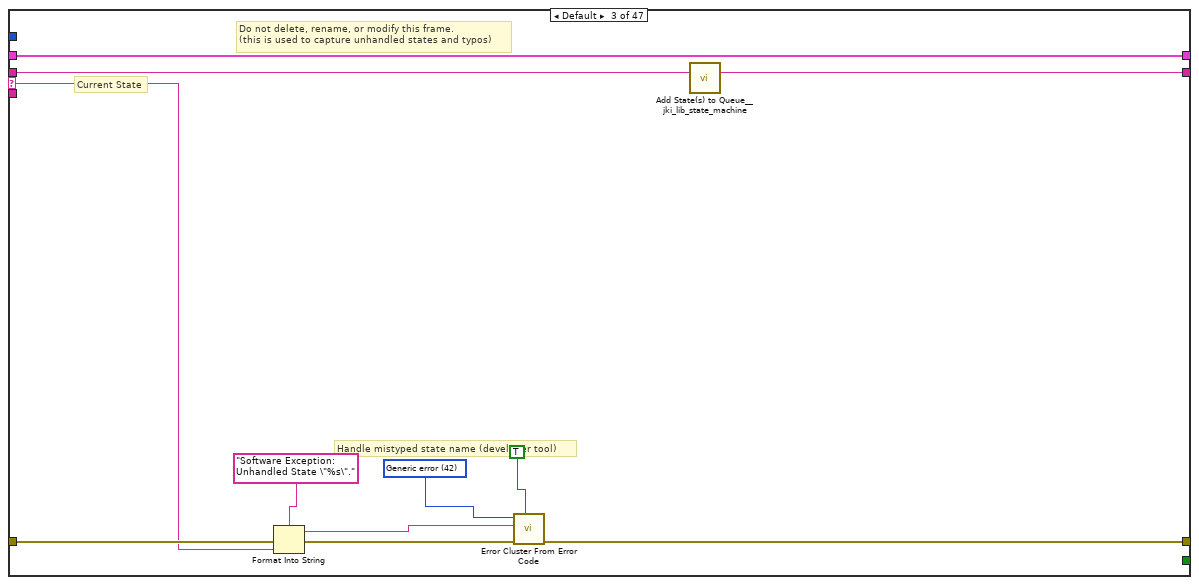
[diagram p20: hidden frame]
diagram:
  # "copy \"Example - Basic IPS-SA.vi\"\nValue (signaling) will execute event if value changes\nUse FGVs to remotely interact with this? (like lockin 4461?)\nwrite values to DSC. Which ones?\nHow to interact with both ITC and IPS? There is problem with \nMercury reference dissapearing"
  # "For instructions on how to use the JKI State Machine, examples and video tutorials, visit:\nhttp://jki.net/state-machine/\n\nJKI State Machine™\nhttp://jki.net/state-machine/\nCopyright (C) 2005-2015, JKI <info@jki.net>\nALL RIGHTS RESERVED"
  # "State Syntax:\nStateCategory: State >> Argument\nLine Terminator: Line feed\nExample:\nUI: Help >> About\n\nWhere \"UI\" is the state category\nWhere \"Help\" is the state\nWhere \"About\" is the argument\nOther Examples:\nApp Data: Initialize\nUI: Initialize\nHelp >> About\n\nCommenting:\nTo add a comment use \"//\" or \"#\" and all text to the right will be ignored\nCommenting Example:\nUI: Initialize // This initializes the UI\n# This whole line is a comment\n// Another comment line"
  # "copy this to create labels for wires"
  # "System_Label"
  n1 = call <vilib>:"Add State(s) to Queue__jki_lib_state_machine.vi"("State(s) in (\"\")"="Macro: Initialize") -> ("States Out"=w2:string)  [unwired: 14 in]
  n2 = while "JKI - String-Based Queued State Machine (Basic) v1.0" {
    shift-right: [w6] -> _
    shift-left: _ -> [w5]
    shift-right: [w9] -> _
    shift-left: _ -> [w3]
    shift-right: [w8] -> _
    shift-left: w2 -> [w10]
    stop <- w7 stop-if-true
    w4 = 10  # Timeout
    # "Template Copyright © 2015 JKI - http://jki.net/state-machine"
    n3 = call <vilib>:"Parse State Queue__jki_lib_state_machine.vi"("State Queue"=w10, "Error In (no error)"=w3) -> ("Remaining States"=w12:string, "Current State"=w13:string, "Arguments"=w11:string)  [unwired: 11 in]
    n4 = case shown="\"Mercury: ITC: Idle\"" w13 {
      selector: w13 -> [_ _ w116 _ _ _ _ _ _ _ _ _ _ _ _ _ _ _ _ _ _ _ _ _ _ _ _ _ _ _ _ _ _ _ _ _ _ _ _ _ _ _ _ _ _ _ _]
      tunnel: w12 -> [w20 w115 w120 w138 w155 w160 w164 w177 w183 w187 w197 w207 w218 w244 w251 w266 w270 w294 w343 w389 w431 w478 w501 w546 w587 w634 w675 w680 w702 w768 w805 w863 w879 w906 w910 w915 w958 w991 w1023 w1042 w1061 w1080 w1102 w1170 w1191 w1212 w1230]
      tunnel: w11 -> [_ _ _ _ _ _ _ _ _ _ _ w202 w212 _ _ _ _ _ _ _ _ _ _ _ _ _ _ _ _ _ _ _ _ _ _ _ _ _ _ _ _ _ _ _ _ _ _]
      tunnel: w5 -> [w16 w112 w118 w129 w141 w158 w161 _ w178 w184 w188 w205 w214 w241 w249 w264 w267 w289 w341 w388 w395 w438 w487 w544 w586 w633 w674 w677 w684 w736 w804 w820 w878 w905 w909 w912 w956 w981 w1018 w1032 w1051 w1070 w1088 w1155 w1181 w1197 w1218]
      tunnel: [w14 w113 w122 w135 errorcluster {"status"=FALSE, "code"=0, "source"=""} ("error out") w157 w162 w171 w179 w185 w192 w203 w215 w242 w248 w254 w268 w272 w303 w344 w392 w441 w488 w508 w553 w606 w641 w678 w687 w737 w776 w816 w876 w890 w908 w913 w924 w975 w1000 w1027 w1045 w1064 w1089 w1148 w1175 w1199 w1217] -> w9
      tunnel: [w19 w114 w119 w137 w154 w159 w163 w176 w182 w186 w196 w206 w217 w243 w250 w265 w269 w293 w342 w390 w432 w479 w502 w545 w588 w635 w676 w679 w703 w769 w806 w864 w880 w907 w911 w914 w959 w992 w1024 w1043 w1062 w1081 w1103 w1171 w1192 w1213 w1231] -> w8
      tunnel: [_ _ _ _ _ TRUE _ _ _ _ _ _ _ _ _ _ _ _ _ _ _ _ _ _ _ _ _ _ _ _ _ _ _ _ _ _ _ _ _ _ _ _ _ _ _ _ _] -> w7
      tunnel: [w18 w112 w118 w136 w140 w158 w161 w175 w178 w184 w189 w205 w214 w241 w249 w264 w267 w288 w341 w388 w395 w438 w487 w544 w586 w633 w674 w677 w683 w736 w804 w820 w878 w905 w909 w912 w956 w981 w1018 w1032 w1051 w1070 w1088 w1155 w1181 w1197 w1218] -> w6
      tunnel: w4 -> [w17 _ _ _ _ _ _ _ _ _ _ _ _ _ _ _ _ _ _ _ _ _ _ _ _ _ _ _ _ _ _ _ _ _ _ _ _ _ _ _ _ _ _ _ _ _ _]
      tunnel: w3 -> [w15 w113 w121 w135 w150 w157 w162 w171 w180 w185 w194 w204 w216 w242 w248 w256 w268 w281 w305 w355 w398 w440 w482 w510 w555 w593 w636 w678 w699 w767 w802 w853 w877 w884 w908 w913 w953 w986 w1015 w1037 w1056 w1075 w1090 w1165 w1182 w1200 w1216]
      frame "", "Event Structure", "Idle" {
        # "executes when the state queue is empty"
        n5 = event shown="[0] Timeout" {
          selector: _ -> [_ _ _ _ _ _ _ _ _ _ _ _ _ _]
          dyn-events: _ -> [_ _ _ _ _ _ _ _ _ _ _ _ _ _]
          timeout: w17 -> [_ _ _ _ _ _ _ _ _ _ _ _ _ _]
          tunnel: w20 -> [w39 w49 w55 w60 w64 w69 w74 w78 w84 w88 w93 w97 w105 w111]
          tunnel: [w38 w48 w54 w59 w63 w68 w73 w77 w83 w87 w92 w96 w104 w110] -> w19
          tunnel: [w21 w47 w51 w56 w61 w66 w71 w76 w81 w90 w95 w100 w102 w108] -> w18
          tunnel: w16 -> [w21 w47 w51 w56 w61 w66 w71 w76 w81 w90 w95 w100 w102 w108]
          tunnel: w15 -> [w24 w46 w52 w58 w65 w67 w72 w80 w82 w86 w91 w99 w103 w109]
          tunnel: [w23 w46 w52 w58 w65 w67 w72 w80 w82 w86 w91 w99 w103 w109] -> w14
          event Timeout {
            # "get remote"
            n6 = event-data() -> ()  [unwired: 1 in, 1 out]
            n7 = call "FGV_PSP - Mercury Remote.vi"("error in"=w24, "Function"=enum16{"write", "read"}."read") -> ("error out"=w23:errorcluster, "Remote"=w22:bool)  [unwired: 4 in]
            n8 = local write "Remote Mode"(w22) -> ()
            n9 = case shown="True" w22 {
              tunnel: ["Mercury: Idle\nMercury: IPS: Idle - 1\nMercury: IPS: Idle - 1a\nMercury: IPS: Idle - 2\nMercury: IPS: Idle - 3\nMercury: ITC: Idle" ("State(s) at Back (\"\")") "Mercury: Remote\nMercury: Idle\nMercury: IPS: Idle - 1\nMercury: IPS: Idle - 1a\nMercury: IPS: Idle - 2\nMercury: IPS: Idle - 3\nMercury: ITC: Idle\n" ("State(s) at Back (\"\")")] -> w27
              frame False {
              }
              frame True {
              }
            }
            n10 = while {
              shift-right: [w42] -> _
              shift-left: _ -> [w43]
              stop <- TRUE stop-if-true
              n11 = Get Date/Time In Seconds() -> (seconds since 1Jan1904=w42:timestamp)
              n12 = Subtract(x=w42, y=w43) -> (x-y=→"Iteration Time":dbl)
            }
            n13 = local read "Magnet Field (T)"() -> (w35:dbl)
            n14 = local read "Target Field (T)"() -> (w34:dbl)
            n15 = local read "Target Field Rate (T/min)"() -> (w37:dbl)
            n16 = local read "Power Supply Field (T)"() -> (w33:dbl)
            n17 = local read "SWITCH HEATER"() -> (w29:bool)
            n18 = local read "PS ON/OFF"() -> (w30:timestamp)
            n19 = local read "LPF ON"() -> (w32:timestamp)
            n20 = local read "Lambda"() -> (w26:bool)
            n21 = call "1820_Calculate_Sweep_Time.vi"("Power Supply Field (T)"=w33, "Target Field Rate (T/min)"=w37, "Magnet Field (T)"=w35, "Target Field (T)"=w34) -> ("ETA"=→"ETA":timestamp)  [unwired: 6 in, 1 out]
            n22 = call "1820_PS_ON_duration.vi"("SWITCH HEATER"=w29, "time stamp"=w30) -> ("PS Heat on (sec)"=→"PS Heat on or off (sec)":dbl)  [unwired: 9 in]
            n23 = call "1820_LPF_ON_duration.vi"("Lambda"=w26, "LPF ON"=w32) -> ("LPF on (min)"=→"LPF on (min)":dbl)  [unwired: 9 in]
            n24 = call <vilib>:"Add State(s) to Queue__jki_lib_state_machine.vi"("State(s) in Front (\"\")"=w27, "State(s) in (\"\")"=w39) -> ("States Out"=w38:string)  [unwired: 13 in]
          }
          event "Remote Mode": Value Change {
            n25 = event-data() -> ()  [unwired: 1 in, 6 out]
            n26 = call <vilib>:"Add State(s) to Queue__jki_lib_state_machine.vi"("State(s) in Front (\"\")"="Mercury: Remote", "State(s) in (\"\")"=w49) -> ("States Out"=w48:string)  [unwired: 13 in]
          }
          event "Hold": Value Change {
            n27 = event-data() -> ()  [unwired: 1 in, 6 out]
            n28 = call <vilib>:"Add State(s) to Queue__jki_lib_state_machine.vi"("State(s) in Front (\"\")"="Mercury: Hold" ("State(s) in Front (\"\")"), "State(s) in (\"\")"=w55) -> ("States Out"=w54:string)  [unwired: 13 in]
          }
          event "Clamp": Value Change {
            n29 = event-data() -> ()  [unwired: 1 in, 6 out]
            n30 = call <vilib>:"Add State(s) to Queue__jki_lib_state_machine.vi"("State(s) in Front (\"\")"="Mercury: Clamp" ("State(s) in Front (\"\")"), "State(s) in (\"\")"=w60) -> ("States Out"=w59:string)  [unwired: 13 in]
          }
          event "To Set": Value Change {
            n31 = event-data() -> ()  [unwired: 1 in, 6 out]
            n32 = call <vilib>:"Add State(s) to Queue__jki_lib_state_machine.vi"("State(s) in Front (\"\")"="Mercury: To Set" ("State(s) in Front (\"\")"), "State(s) in (\"\")"=w64) -> ("States Out"=w63:string)  [unwired: 13 in]
          }
          event "To Zero": Value Change {
            n33 = event-data() -> ()  [unwired: 1 in, 6 out]
            n34 = call <vilib>:"Add State(s) to Queue__jki_lib_state_machine.vi"("State(s) in Front (\"\")"="Mercury: To Zero" ("State(s) in Front (\"\")"), "State(s) in (\"\")"=w69) -> ("States Out"=w68:string)  [unwired: 13 in]
          }
          event "PS Heat": Value Change {
            n35 = event-data() -> ()  [unwired: 1 in, 6 out]
            n36 = call <vilib>:"Add State(s) to Queue__jki_lib_state_machine.vi"("State(s) in Front (\"\")"="Mercury: PS Heat" ("State(s) in Front (\"\")"), "State(s) in (\"\")"=w74) -> ("States Out"=w73:string)  [unwired: 13 in]
          }
          event "Send to IPS": Value Change {
            n37 = event-data() -> ()  [unwired: 1 in, 6 out]
            n38 = call <vilib>:"Add State(s) to Queue__jki_lib_state_machine.vi"("State(s) in Front (\"\")"="Mercury: Send To IPS" ("State(s) in Front (\"\")"), "State(s) in (\"\")"=w78) -> ("States Out"=w77:string)  [unwired: 13 in]
          }
          event "Lambda": Value Change {
            # "set lambda"
            n39 = event-data() -> ()  [unwired: 1 in, 6 out]
            n40 = call <vilib>:"Add State(s) to Queue__jki_lib_state_machine.vi"("State(s) in Front (\"\")"="Mercury: Lambda" ("State(s) in Front (\"\")"), "State(s) in (\"\")"=w84) -> ("States Out"=w83:string)  [unwired: 13 in]
          }
          event "Fast/Slow Fill": Value Change {
            n41 = event-data() -> ()  [unwired: 1 in, 6 out]
            n42 = call <vilib>:"Add State(s) to Queue__jki_lib_state_machine.vi"("State(s) in Front (\"\")"="Mercury: Fast/Slow Fill" ("State(s) in Front (\"\")"), "State(s) in (\"\")"=w88) -> ("States Out"=w87:string)  [unwired: 13 in]
          }
          event "Heater Current": Value Change {
            n43 = event-data() -> ()  [unwired: 1 in, 6 out]
            n44 = call <vilib>:"Add State(s) to Queue__jki_lib_state_machine.vi"("State(s) in Front (\"\")"="Mercury: Heater Current" ("State(s) in Front (\"\")"), "State(s) in (\"\")"=w93) -> ("States Out"=w92:string)  [unwired: 13 in]
          }
          event "Close Needle Valve", "Open Needle Valve": Value Change {
            n45 = event-data() -> ()  [unwired: 1 in, 6 out]
            n46 = call <vilib>:"Add State(s) to Queue__jki_lib_state_machine.vi"("State(s) in Front (\"\")"="Mercury: Needle Valve" ("State(s) in Front (\"\")"), "State(s) in (\"\")"=w97) -> ("States Out"=w96:string)  [unwired: 13 in]
          }
          event "OK": Value Change {
            # "Exit Button Value Change (pressed) Event\n(this executes Macro: Exit to terminate the VI)"
            n47 = event-data() -> ()  [unwired: 1 in, 1 out]
            n48 = call <vilib>:"Add State(s) to Queue__jki_lib_state_machine.vi"("State(s) in Front (\"\")"="Macro: Exit", "State(s) in (\"\")"=w105) -> ("States Out"=w104:string)  [unwired: 13 in]
          }
          event Panel Close? {
            # "Discard the event because we'll close the front panel ourselves in Macro: Exit"
            # "Close Panel button (pressed) Event\n(this executes Macro: Exit to terminate the VI)"
            n49 = event-data() -> ()  [unwired: 1 in, 1 out]
            n50 = call <vilib>:"Add State(s) to Queue__jki_lib_state_machine.vi"("State(s) in Front (\"\")"="Macro: Exit", "State(s) in (\"\")"=w111) -> ("States Out"=w110:string)  [unwired: 13 in]
            n51 = event-data("Discard?"=TRUE) -> ()  [unwired: 1 in, 1 out]
          }
        }
      }
      frame "---------- Core ----------" {
        # "Do not put any code in this frame.\n(it is a separator no-op)"
        n52 = call <vilib>:"Add State(s) to Queue__jki_lib_state_machine.vi"("State(s) in (\"\")"=w115) -> ("States Out"=w114:string)  [unwired: 14 in]
      }
      frame Default {
        w125 = 42 items=["No error", "Argument error", "Memory is full", "Out of zone", "End of file", "File already open", "Generic file I/O error", "File not found", "File permission error", "Disk is full", "Duplicate path", "Too many files open", "System feature not enabled", "Resource file not found", "Cannot add resource", "Resource not found", "Image not found", "Image memory error", "Pen does not exist", "Config type invalid", "Config token not found", "Config parse error", "Config memory error", "Bad external code format", "Bad external code offset", "External code not present", "Null window", "Destroy window error", "Null menu", "Print aborted", "Bad print record", "Print driver error", "Windows error during printing", "Memory error during printing", "Print dialog error", "Generic print error", "Invalid device refnum", "Device not found", "Device parameter error", "Device unit error", "Cannot open device", "Device call aborted", "Generic error", "Cancelled by user", "Object ID too low", "Object ID too high", "Object not in heap", "Unknown heap", "Unknown object (invalid DefProc)", "Unknown object (DefProc not in table)", "Message out of range", "Invalid (null) method", "Unknown message", "Manager call not supported", "Bad address", "Network operation in progress", "Network operation timed out", "Connection is busy", "Network attribute not supported", "Network error", "Address in use", "System out of memory", "Connection aborted", "Connection refused", "Not connected", "Already connected", "Connection closed", "Initialization error (interapplication manager)", "Bad occurrence", "Wait on unbound occurrence handler", "Occurrence queue overflow", "Datalog type conflict", "Unused", "Unrecognized type (interapplication manager)", "Memory corrupt", "Failed to make temporary DLL", "Old CIN version", "Drag socket not found", "Failed to load drop-object", "Failed to register OLE object", "Failed to release OLE object", "Format specifier type mismatch", "Unknown format specifier", "Too few format specifiers", "Too many format specifiers", "Scan failed", "Newer CIN version", "Error converting to variant", "Runtime menu error", "Password tampered", "Variant attribute not found", "Incompatible variant data type", "Event data is not available", "Event Store is not present", "Occurrence is not found", "Event Queue is not created", "Event info is not available", "Refnum passed is NULL", "Error retrieving Class GUID", "Error retrieving CoClass GUID", "Error retrieving TypeLib GUID.", "Bad built application magic bytes.", "Specific driver is different from the specific driver associated with the Logical Name.", "There is no session opened to the class driver.", "Max Error", "MAX - Error with config objects", "MAX - Error loading configuration", "MAX - Group not supported"]
        # "Current State"
        # "Do not delete, rename, or modify this frame.\n(this is used to capture unhandled states and typos)"
        # "Handle mistyped state name (developer tool)"
        n53 = Format Into String(format string="Software Exception: Unhandled State \"%s\"." ("message"), error in=w121, w116) -> (resulting string=w124:string, error out=w123:errorcluster)  [unwired: 1 in]
        n54 = call <vilib>:"Error Cluster From Error Code.vi"("show call chain? (False)"=TRUE, "error in (no error)"=w123, "error message (\"\")"=w124, "error code (0)"=w125) -> ("error out"=w122:errorcluster)  [unwired: 5 in]
        n55 = call <vilib>:"Add State(s) to Queue__jki_lib_state_machine.vi"("State(s) in (\"\")"=w120) -> ("States Out"=w119:string)  [unwired: 14 in]
      }
      frame "Initialize Core Data" {
        # "Do not delete, rename, or modify this frame.\n(this is used to determine panel behavior on exit)"
        # "originally closed?"
        # "exe?"
        # "If panel starts closed or is an EXE, then close it when we exit"
        n56 = property class="VI"() -> ("Front Panel.Open"=w134:bool)  [unwired: 2 in, 2 out]
        n57 = property class="App"() -> ("App.Kind"=w133:T26)  [unwired: 2 in, 2 out]
        n58 = control-ref of="Current VI Reference"() -> (w127:refnum<vi>)
        n59 = Not(x=w134) -> (.not. x?=w131:bool)
        n60 = Equal?(x=w133, y=T26."Run Time System" ("Application:Kind")) -> (x = y?=w130:bool)
        n61 = Or(x=w131, y=w130) -> (x .or. y?=w128:bool)
        n62 = Bundle By Name(cluster=w129, "Core.Current VI Reference"=w127, "Core.Close Panel on Exit?"=w128) -> (w136:T38)
        n63 = call <vilib>:"Add State(s) to Queue__jki_lib_state_machine.vi"("State(s) in (\"\")"=w138) -> ("States Out"=w137:string)  [unwired: 14 in]
      }
      frame "Error Handler" {
        w149 = i32[] [-1950679035, -1950678943]  # Error Codes to Filter
        # "Unhandled Error -- Display it"
        # "Handle any errors here.\nYou can also output any states to clean-up after errors occur"
        # "Clear error"
        n64 = call-poly <userlib>:"Filter Error Codes__ogtk.vi"("Error In"=w150, "Error Codes to Filter"=w149) -> ("Error Out"=w151:errorcluster, "Filtered Error Details"=w148:T39)  [unwired: 7 in, 1 out]
        n65 = Unbundle(w148) -> ("code"=w146:i32, "source"=w147:string)
        n66 = Get Date/Time In Seconds() -> (seconds since 1Jan1904=w145:timestamp)
        n67 = Unbundle By Name(w141) -> ("Error Log"=w143:T25)
        n68 = Bundle By Name(cluster=T27 {"time"=timestamp(0 s since 1904-01-01), "code"=0, "source"=""} ("output cluster"), "time"=w145, "code"=w146, "source"=w147) -> (w142:T27)
        n69 = Build Array (concatenate)(w143, w142) -> (w139:T25)
        "Error List" <- w139
        n70 = Bundle By Name(cluster=w141, "Error Log"=w139) -> (w140:T38)
        n71 = call <vilib>:"General Error Handler.vi"("error in (no error)"=w151) -> ()  [unwired: 10 in, 5 out]
        n72 = call <vilib>:"Add State(s) to Queue__JKI_lib_State_Machine.vi"("State(s) in Front (\"\")"="/* Post Error States", "State(s) in (\"\")"=w155) -> ("States Out"=w154:string)  [unwired: 13 in]
      }
      frame "Exit" {
        # "Do not put any code in this frame.\n(No errors that occur here will be handled.)"
        n73 = call <vilib>:"Add State(s) to Queue__jki_lib_state_machine.vi"("State(s) in (\"\")"=w160) -> ("States Out"=w159:string)  [unwired: 14 in]
      }
      frame "---------- Data ----------" {
        # "Do not put any code in this frame.\n(It is a separator no-op. You can make a copy of this frame to create a new Data frame)"
        n74 = call <vilib>:"Add State(s) to Queue__jki_lib_state_machine.vi"("State(s) in (\"\")"=w164) -> ("States Out"=w163:string)  [unwired: 14 in]
      }
      frame "Data: Initialize" {
        w165 = bool[] [FALSE, FALSE, FALSE, FALSE, FALSE, FALSE, FALSE, FALSE]  # LEDs
        w166 = 0  # counter
        w168 = TRUE  # read ITC T?
        w169 = T35 {"Comms"="", "Device ID"=[], "Comms Layer"=enum."Ethernet TCP/IP", "Command"="", "Query reference"=refnum}  # Mercury ITC Ref
        w170 = T25 []  # Error Log
        w172 = TRUE  # sentinel
        w173 = T35 {"Comms"="", "Device ID"=[], "Comms Layer"=enum."Ethernet TCP/IP", "Command"="", "Query reference"=refnum}  # Mercury IPS Ref
        w174 = T40 {"Current VI Reference"=refnum, "Close Panel on Exit?"=FALSE}  # Core
        # "read FGV in timeout"
        # "do not delete - used by framework"
        # "Data names and types of shift register data are defined by this bundle."
        # "Initialize the shift-register data, here.\n(data names are defined by what you wire into the bundle function)"
        n75 = call <vilib>:"Add State(s) to Queue__jki_lib_state_machine.vi"("State(s) in (\"\")"=w177) -> ("States Out"=w176:string)  [unwired: 14 in]
        n76 = call "MercuryStateHistory.vi"("initialize?"=TRUE) -> ()  [unwired: 9 in, 2 out]
        n77 = Bundle("Core"=w174, "Mercury ITC Ref"=w169, "Mercury IPS Ref"=w173, "sentinel"=w172, "Error Log"=w170, "read ITC T?"=w168, "counter"=w166, "LEDs"=w165) -> (w175:T38)  [unwired: 1 in]
      }
      frame "Data: Cleanup" {
        # "Cleanup any data and references, here.\n(this is called automatically, by the Macro: Exit)"
        n78 = Unbundle By Name(w178) -> ("Core.Current VI Reference"=w181:refnum<vi>)
        n79 = Close Reference(reference=w181, error in (no error)=w180) -> (error out=w179:errorcluster)
        n80 = call <vilib>:"Add State(s) to Queue__jki_lib_state_machine.vi"("State(s) in (\"\")"=w183) -> ("States Out"=w182:string)  [unwired: 14 in]
      }
      frame "---------- UI ----------" {
        # "Do not put any code in this frame.\n(It is a separator no-op. You can make a copy of this frame to create a new UI frame)"
        n81 = call <vilib>:"Add State(s) to Queue__jki_lib_state_machine.vi"("State(s) in (\"\")"=w187) -> ("States Out"=w186:string)  [unwired: 14 in]
      }
      frame "UI: Initialize" {
        w190 = bool[] [TRUE, FALSE, TRUE, FALSE, TRUE, FALSE, TRUE, FALSE] ("LEDs")
        w193 = FALSE
        # "start in local mode"
        # "Initialize the User Interface, here.\n(this is called automatically, by the Macro: Init)"
        n82 = disable-structure shown="Enabled" {
          frame Disabled {
            n83 = Open Application Reference() -> (0:w199:errorcluster, 3:w198:refnum<vi>)  [unwired: 4 in]
            n84 = Open VI Reference(vi path=path "") -> ()  [unwired: 5 in, 2 out]
            n85 = property class="App"(reference=w198, error in=w199, "WebSrvr.Active"=TRUE ("Web Server:Server Active")) -> ()  [unwired: 2 out]
            n86 = call "MNK_Dashboard_v2.vi"() -> ()  [unwired: 12 in]
          }
          frame Enabled {
          }
        }
        n87 = call <userlib>:"Fit VI window to Largest Dec__ogtk.vi"("error in (no error)"=w194) -> ("error out"=w191:errorcluster)  [unwired: 5 in, 1 out]
        n88 = local write "Remote Mode"(w193) -> ()
        n89 = call <vilib>:"Add State(s) to Queue__jki_lib_state_machine.vi"("State(s) in (\"\")"=w197) -> ("States Out"=w196:string)  [unwired: 14 in]
        n90 = call "FGV_PSP - Mercury Remote.vi"("error in"=w191, "Remote"=w193) -> ("error out"=w192:errorcluster)  [unwired: 4 in, 1 out]
        n91 = local write "LEDs"(w190) -> ()
        n92 = Bundle By Name(cluster=w188, "LEDs"=w190) -> (w189:T38)
        "Magnet Status 2" <- "" ("Magnet Status 2")
      }
      frame "UI: Cursor Set" {
        # "Argument"
        # "Set and Unset Cursor Busy.\n(Usage: \"UI: Cursor Set >> Busy|Idle\")"
        n93 = case shown="\"Idle\", Default" w202 {
          tunnel: w204 -> [w209 w211]
          tunnel: [w208 w210] -> w203
          frame "Idle", Default {
            n94 = call <vilib>:"Unset Busy.vi"("error in (no error)"=w209) -> ("error out"=w208:errorcluster)  [unwired: 10 in]
          }
          frame "Busy" {
            n95 = call <vilib>:"Set Busy.vi"("error in (no error)"=w211) -> ("error out"=w210:errorcluster)  [unwired: 9 in, 1 out]
          }
        }
        n96 = call <vilib>:"Add State(s) to Queue__JKI_lib_State_Machine.vi"("State(s) in (\"\")"=w207) -> ("States Out"=w206:string)  [unwired: 14 in]
      }
      frame "UI: Front Panel State" {
        # "Argument"
        # "Set Front Panel Open or Closed\n(Usage: \"UI: Front Panel State >> Open|Close\")"
        n97 = Unbundle By Name(w214) -> ("Core.Current VI Reference"=w213:refnum<vi>)
        n98 = case shown="\"Open\", Default" w212 {
          tunnel: w216 -> [w222 w235]
          tunnel: [w224 w236] -> w215
          tunnel: w213 -> [w223 w233]
          frame "Open", Default {
            n99 = property class="VI"(reference=w223, error in=w222) -> (reference out=w220:refnum<vi>, error out=w221:errorcluster, "Front Panel.Open"=w219:bool)
            n100 = case shown="True" w219 {
              tunnel: [w227 w230] -> w224
              tunnel: w221 -> [w226 w230]
              tunnel: w220 -> [w225 _]
              frame False {
                n101 = invoke class="VI" method="FP.Open"(reference=w225, error in=w226, "Activate"=TRUE, "State"=T28."Standard") -> (error out=w227:errorcluster)  [unwired: 1 in, 4 out]
              }
              frame True {
              }
            }
          }
          frame "Close" {
            n102 = property class="VI"(reference=w233, error in=w235) -> (reference out=w232:refnum<vi>, error out=w234:errorcluster, "Front Panel.Open"=w231:bool)
            n103 = case shown="True" w231 {
              tunnel: [w237 w240] -> w236
              tunnel: w234 -> [w237 w239]
              tunnel: w232 -> [_ w238]
              frame False {
              }
              frame True {
                n104 = invoke class="VI" method="FP.Close"(reference=w238, error in=w239) -> (error out=w240:errorcluster)  [unwired: 1 in, 2 out]
              }
            }
          }
        }
        n105 = call <vilib>:"Add State(s) to Queue__JKI_lib_State_Machine.vi"("State(s) in (\"\")"=w218) -> ("States Out"=w217:string)  [unwired: 14 in]
      }
      frame "---------- Macro ----------" {
        # "Do not put any code in this frame.\n(It is a separator no-op. You can make a copy of this frame to create a new Macro frame)"
        n106 = call <vilib>:"Add State(s) to Queue__JKI_lib_State_Machine.vi"("State(s) in (\"\")"=w244) -> ("States Out"=w243:string)  [unwired: 14 in]
      }
      frame "Macro: Initialize" {
        w247 = "Data: Initialize\nInitialize Core Data\nUI: Initialize\nUI: Front Panel State >> Open"  # Data: Initialize Initialize Core Data UI: Initialize UI: Front Panel State >> Open
        # "Initialization Macro\n(This is called once, when the VI starts)"
        n107 = call <vilib>:"Add State(s) to Queue__JKI_lib_State_Machine.vi"("State(s) in Front (\"\")"=w247, "State(s) at Back (\"\")"="Mercury: Initialize") -> ("States Out"=w246:string)  [unwired: 13 in]
        n108 = call <vilib>:"Add State(s) to Queue__JKI_lib_State_Machine.vi"("State(s) in Front (\"\")"=w246, "State(s) in (\"\")"=w251) -> ("States Out"=w250:string)  [unwired: 13 in]
      }
      frame "Macro: Exit" {
        # "#Implemented in Close Instrument.vi"
        # "Exit Macro\n(This is called once, when the VI exits)"
        n109 = Unbundle By Name(w264) -> ("Core.Close Panel on Exit?"=w263:bool, "Mercury ITC Ref"=w252:T35, "Mercury IPS Ref"=w253:T35)
        n110 = call <instrlib>:"Close.vi"("error in (no error)"=w256, "Mercury Reference"=w253) -> ("error out"=w255:errorcluster)  [unwired: 9 out]
        n111 = call <instrlib>:"Close.vi"("error in (no error)"=w255, "Mercury Reference"=w252) -> ("error out"=w257:errorcluster)  [unwired: 9 out]
        n112 = call <vilib>:"Simple Error Handler.vi"("error in (no error)"=w257) -> ("error out"=w254:errorcluster)  [unwired: 1 in, 7 out]
        n113 = Select(t="UI: Front Panel State >> Close", s=w263, f="") -> (s? t:f=w260:string)
        n114 = call <vilib>:"Add State(s) to Queue__JKI_lib_State_Machine.vi"("State(s) in (\"\")"=w260, "State(s) at Back (\"\")"="Data: Cleanup\nExit") -> ("States Out"=w258:string)  [unwired: 13 in]
        n115 = call <vilib>:"Add State(s) to Queue__JKI_lib_State_Machine.vi"("State(s) in Front (\"\")"=w258, "State(s) in (\"\")"=w266) -> ("States Out"=w265:string)  [unwired: 13 in]
      }
      frame "---------- Mercury: Query ----------" {
        n116 = call <vilib>:"Add State(s) to Queue__JKI_lib_State_Machine.vi"("State(s) in (\"\")"=w270) -> ("States Out"=w269:string)  [unwired: 14 in]
      }
      frame "Mercury: Initialize" {
        w280 = Comms_Transport_Layer."Ethernet TCP/IP" ("Comms Layer")
        # "#Implemented in Open Instrument.vi"
        n117 = call-poly <instrlib>:"Open.vi"("Clear Previous Connections (False)"=TRUE ("Clear Previous Connections (True)"), "ID Query (True)"=TRUE, "IP Address"="ITC IP Address", "error in (no error)"=w281, "Comms Layer"=w280) -> ("error out"=w275:errorcluster, "# of Instruments"=→"# of Instruments":i32, "Serial Number(s)"=→"Serial Number(s)":string[], "Mercury Reference Out"=w276:T35, "S/W Version(s)"=→"S/W Version(s)":string[])  [unwired: 2 in]
        n118 = call-poly <instrlib>:"Open.vi"("Clear Previous Connections (False)"=FALSE ("Clear Previous Connections (True)"), "ID Query (True)"=TRUE, "IP Address"="IPS IP Address", "error in (no error)"=w275, "Comms Layer"=w280) -> ("error out"=w272:errorcluster, "# of Instruments"=→"# of Instruments 2":i32, "Serial Number(s)"=→"Serial Number(s) 2":string[], "Mercury Reference Out"=w274:T35, "S/W Version(s)"=→"S/W Version(s) 2":string[])  [unwired: 2 in]
        n119 = case shown="No Error" w272 {
          tunnel: ["Mercury: Query ITC: System\nMercury: Query IPS: System\nMercury: Query ITC: Temperature\nMercury: Query ITC: Heater\nMercury: Query ITC: Aux\nMercury: Query ITC: Pressure\nMercury: Query IPS: LVL\nMercury: Query IPS: Temperature\nMercury: Query IPS: Magnet" ("State(s) at Back (\"\")") "Error Handler\nMacro: Exit" ("State(s) at Back (\"\")")] -> w273
          tunnel: [bool[] [TRUE, FALSE, TRUE, FALSE, TRUE, FALSE, TRUE, FALSE] ("LEDs") w298] -> w271
          frame No Error {
            n120 = local write "LEDs"(bool[] [TRUE, TRUE, TRUE, TRUE, TRUE, TRUE, TRUE, TRUE] ("LEDs")) -> ()
          }
          frame Error {
            w298 = bool[] [FALSE, FALSE, FALSE, FALSE, FALSE, FALSE, FALSE, FALSE] ("LEDs")
            n121 = local write "LEDs"(w298) -> ()
          }
        }
        n122 = Bundle By Name(cluster=w289, "Mercury ITC Ref"=w276, "Mercury IPS Ref"=w274, "LEDs"=w271) -> (w288:T38)
        n123 = call <vilib>:"Add State(s) to Queue__JKI_lib_State_Machine.vi"("State(s) in Front (\"\")"=w273, "State(s) in (\"\")"=w294) -> ("States Out"=w293:string)  [unwired: 13 in]
      }
      frame "Mercury: Query ITC: System" {
        n124 = Unbundle By Name(w341) -> ("Mercury ITC Ref"=w301:T35)
        n125 = call-poly <instrlib>:"Configuration (Read).vi"("error in"=w305, "Mercury Reference In"=w301) -> ("error out"=w337:errorcluster, "Devices"=→"ITC Devices":string[], "Mercury Reference Out"=w338:T35)  [unwired: 1 in, 6 out]
        n126 = call-poly <instrlib>:"Configuration (Read).vi"("error in"=w337, "Mercury Reference In"=w338) -> ("error out"=w330:errorcluster, "Automatic Dimming"=→"Automatic Dimming":string, "Mercury Reference Out"=w331:T35)  [unwired: 1 in, 6 out]
        n127 = call-poly <instrlib>:"Configuration (Read).vi"("error in"=w330, "Mercury Reference In"=w331) -> ("error out"=w333:errorcluster, "Dimming Time"=→"Dimming Time":string, "Mercury Reference Out"=w332:T35)  [unwired: 1 in, 6 out]
        n128 = call-poly <instrlib>:"Configuration (Read).vi"("error in"=w333, "Mercury Reference In"=w332) -> ("error out"=w339:errorcluster, "Display Brightness"=→"Display Brightness":string, "Mercury Reference Out"=w340:T35)  [unwired: 1 in, 6 out]
        n129 = call-poly <instrlib>:"Configuration (Read).vi"("error in"=w339, "Mercury Reference In"=w340) -> ("error out"=w324:errorcluster, "Date"=→"Date":string, "Mercury Reference Out"=w323:T35)  [unwired: 1 in, 6 out]
        n130 = call-poly <instrlib>:"Configuration (Read).vi"("error in"=w324, "Mercury Reference In"=w323) -> ("error out"=w326:errorcluster, "Time"=→"Time":string, "Mercury Reference Out"=w325:T35)  [unwired: 1 in, 6 out]
        n131 = call-poly <instrlib>:"Configuration (Read).vi"("error in"=w326, "Mercury Reference In"=w325) -> ("error out"=w304:errorcluster, "time stamp"=→"time stamp":timestamp, "Mercury Reference Out"=w302:T35)  [unwired: 1 in, 6 out]
        n132 = call-poly <instrlib>:"Configuration (Read).vi"("error in"=w304, "Mercury Reference In"=w302) -> ("error out"=w322:errorcluster, "Hardware Version"=→"Hardware Version":string, "Mercury Reference Out"=w321:T35)  [unwired: 1 in, 6 out]
        n133 = call-poly <instrlib>:"Configuration (Read).vi"("error in"=w322, "Mercury Reference In"=w321) -> ("error out"=w320:errorcluster, "Firmware Version"=→"Firmware Version":string, "Mercury Reference Out"=w319:T35)  [unwired: 1 in, 6 out]
        n134 = call-poly <instrlib>:"Configuration (Read).vi"("error in"=w320, "Mercury Reference In"=w319) -> ("error out"=w307:errorcluster, "Serial Number"=→"Serial Number":string, "Mercury Reference Out"=w306:T35)  [unwired: 1 in, 6 out]
        n135 = call-poly <instrlib>:"Configuration (Read).vi"("error in"=w307, "Mercury Reference In"=w306) -> ("error out"=w313:errorcluster, "Free Space"=→"Free Space":i32, "Mercury Reference Out"=w312:T35)  [unwired: 1 in, 6 out]
        n136 = call-poly <instrlib>:"Configuration (Read).vi"("error in"=w313, "Mercury Reference In"=w312) -> ("error out"=w309:errorcluster, "Mode"=→"String":T32, "Mercury Reference Out"=w310:T35)  [unwired: 1 in, 6 out]
        n137 = Get Date/Time In Seconds() -> (seconds since 1Jan1904=w318:timestamp)
        n138 = call-poly <instrlib>:"Configuration (Set).vi"("error in"=w309, "time stamp"=w318, "Mercury Reference In"=w310) -> ("error out"=w303:errorcluster, "Response"=→"Set Date Response":T34)  [unwired: 1 in, 6 out]
        n139 = call <vilib>:"Add State(s) to Queue__JKI_lib_State_Machine.vi"("State(s) in (\"\")"=w343) -> ("States Out"=w342:string)  [unwired: 14 in]
      }
      frame "Mercury: Query ITC: Temperature" {
        # "Temperature"
        n140 = Unbundle By Name(w388) -> ("Mercury ITC Ref"=w350:T35)
        n141 = local read "ITC Devices"() -> (w349:string[])
        n142 = Index Array(array=w349, index=3) -> (element=w351:string)
        n143 = call-poly <instrlib>:"Open.vi"("error in (no error)"=w355, "Device Identifier"=w351, "Mercury Reference In"=w350) -> ("error out"=w367:errorcluster, "Mercury Reference Out"=w368:T35)  [unwired: 7 out]
        n144 = call-poly <instrlib>:"Configuration (Read).vi"("error in"=w367, "Mercury Reference In"=w368) -> ("error out"=w359:errorcluster, "Serial Number"=→"Temp S/N":string, "Mercury Reference Out"=w358:T35)  [unwired: 1 in, 6 out]
        n145 = call-poly <instrlib>:"Configuration (Read).vi"("error in"=w359, "Mercury Reference In"=w358) -> ("error out"=w361:errorcluster, "Nickname"=→"T Nickname":string, "Mercury Reference Out"=w360:T35)  [unwired: 1 in, 6 out]
        n146 = call-poly <instrlib>:"Configuration (Read).vi"("error in"=w361, "Mercury Reference In"=w360) -> ("error out"=w364:errorcluster, "Unit"=→"Unit":T3, "Excitation Magnitude"=→"Excitation Magnitude":dbl, "Mercury Reference Out"=w363:T35)  [unwired: 1 in, 5 out]
        n147 = call-poly <instrlib>:"Configuration (Read).vi"("error in"=w364, "Mercury Reference In"=w363) -> ("error out"=w354:errorcluster, "Sensor Type"=→"Sensor Type":T41, "Mercury Reference Out"=w352:T35)  [unwired: 1 in, 6 out]
        n148 = call-poly <instrlib>:"Configuration (Read).vi"("error in"=w354, "Mercury Reference In"=w352) -> ("error out"=w370:errorcluster, "Excitation Type"=→"Excitation Type":T7, "Mercury Reference Out"=w371:T35)  [unwired: 1 in, 6 out]
        n149 = call-poly <instrlib>:"Configuration (Read).vi"("error in"=w370, "Mercury Reference In"=w371) -> ("error out"=w372:errorcluster, "Unit"=→"H Unit":T3, "Hot Limit"=→"Hot Limit":dbl, "Mercury Reference Out"=w373:T35)  [unwired: 1 in, 5 out]
        n150 = call-poly <instrlib>:"Configuration (Read).vi"("error in"=w372, "Mercury Reference In"=w373) -> ("error out"=w379:errorcluster, "Unit"=→"C Unit":T3, "Cold Limit"=→"Cold Limit":dbl, "Mercury Reference Out"=w378:T35)  [unwired: 1 in, 5 out]
        n151 = call-poly <instrlib>:"Signals (Read).vi"("error in"=w379, "Mercury Reference In"=w378) -> ("error out"=w383:errorcluster, "Unit"=→"V Unit":T3, "Voltage"=→"Voltage":dbl, "Mercury Reference Out"=w382:T35)  [unwired: 1 in, 5 out]
        n152 = call-poly <instrlib>:"Signals (Read).vi"("error in"=w383, "Mercury Reference In"=w382) -> ("error out"=w384:errorcluster, "Unit"=→"T Unit":T3, "Temperature"=→"Temperature":dbl, "Mercury Reference Out"=w387:T35)  [unwired: 1 in, 5 out]
        n153 = call-poly <instrlib>:"Configuration (Read).vi"("error in"=w384, "Mercury Reference In"=w387) -> ("error out"=w344:errorcluster, "Device Details"=w345:T42)  [unwired: 1 in, 7 out]
        n154 = Unbundle By Name(w345) -> ("Manufacturing"=→"ITC Manufacturing":T8, "Excitation"=→"ITC Excitation":T6, "Calibration"=→"ITC Calibration":T4)
        n155 = call <vilib>:"Add State(s) to Queue__JKI_lib_State_Machine.vi"("State(s) in (\"\")"=w389) -> ("States Out"=w390:string)  [unwired: 14 in]
      }
      frame "Mercury: Query ITC: Heater" {
        # "Heater"
        n156 = Unbundle By Name(w395) -> ("Mercury ITC Ref"=w394:T35)
        n157 = local read "ITC Devices"() -> (w396:string[])
        n158 = Index Array(array=w396, index=2) -> (element=w391:string)
        n159 = call-poly <instrlib>:"Open.vi"("error in (no error)"=w398, "Device Identifier"=w391, "Mercury Reference In"=w394) -> ("error out"=w401:errorcluster, "Mercury Reference Out"=w400:T35)  [unwired: 7 out]
        n160 = call-poly <instrlib>:"Configuration (Read).vi"("error in"=w401, "Mercury Reference In"=w400) -> ("error out"=w408:errorcluster, "Device Details"=→"Heater Device Settings":T9, "Mercury Reference Out"=w407:T35)  [unwired: 1 in, 6 out]
        n161 = call-poly <instrlib>:"Configuration (Read).vi"("error in"=w408, "Mercury Reference In"=w407) -> ("error out"=w410:errorcluster, "Nickname"=→"Htr Nickname":string, "Mercury Reference Out"=w409:T35)  [unwired: 1 in, 6 out]
        n162 = call-poly <instrlib>:"Configuration (Read).vi"("error in"=w410, "Mercury Reference In"=w409) -> ("error out"=w403:errorcluster, "Serial Number"=→"Htr S/N":string, "Mercury Reference Out"=w402:T35)  [unwired: 1 in, 6 out]
        n163 = call-poly <instrlib>:"Configuration (Read).vi"("error in"=w403, "Mercury Reference In"=w402) -> ("error out"=w399:errorcluster, "Unit"=→"Volt Unit":T3, "Voltage Limit"=→"Htr Voltage Limit":dbl, "Mercury Reference Out"=w393:T35)  [unwired: 1 in, 5 out]
        n164 = call-poly <instrlib>:"Configuration (Read).vi"("error in"=w399, "Mercury Reference In"=w393) -> ("error out"=w413:errorcluster, "Unit"=→"Res Unit":T3, "Nominal Resistance"=→"Htr Resistance":dbl, "Mercury Reference Out"=w414:T35)  [unwired: 1 in, 5 out]
        n165 = call-poly <instrlib>:"Configuration (Read).vi"("error in"=w413, "Mercury Reference In"=w414) -> ("error out"=w420:errorcluster, "Unit"=→"Power Unit":T3, "Maximum Power"=→"Maximum Power":dbl, "Mercury Reference Out"=w419:T35)  [unwired: 1 in, 5 out]
        n166 = call-poly <instrlib>:"Signals (Read).vi"("error in"=w420, "Mercury Reference In"=w419) -> ("error out"=w422:errorcluster, "Unit"=→"Htr V Unit":T3, "Voltage"=→"Htr Voltage":dbl, "Mercury Reference Out"=w421:T35)  [unwired: 1 in, 5 out]
        n167 = call-poly <instrlib>:"Signals (Read).vi"("error in"=w422, "Mercury Reference In"=w421) -> ("error out"=w424:errorcluster, "Unit"=→"Htr P Unit":T3, "Power"=→"Htr Power":dbl, "Mercury Reference Out"=w423:T35)  [unwired: 1 in, 5 out]
        n168 = call-poly <instrlib>:"Signals (Read).vi"("error in"=w424, "Mercury Reference In"=w423) -> ("error out"=w392:errorcluster, "Unit"=→"Htr C Unit":T3, "Current"=→"Htr Current":dbl)  [unwired: 1 in, 6 out]
        n169 = call <vilib>:"Add State(s) to Queue__JKI_lib_State_Machine.vi"("State(s) in (\"\")"=w431) -> ("States Out"=w432:string)  [unwired: 14 in]
      }
      frame "Mercury: Query ITC: Aux" {
        # "Auxiliary"
        n170 = Unbundle By Name(w438) -> ("Mercury ITC Ref"=w433:T35)
        n171 = local read "ITC Devices"() -> (w436:string[])
        n172 = Index Array(array=w436, index=0) -> (element=w434:string)
        n173 = call-poly <instrlib>:"Open.vi"("error in (no error)"=w440, "Device Identifier"=w434, "Mercury Reference In"=w433) -> ("error out"=w460:errorcluster, "Mercury Reference Out"=w461:T35)  [unwired: 7 out]
        n174 = call-poly <instrlib>:"Configuration (Read).vi"("error in"=w460, "Mercury Reference In"=w461) -> ("error out"=w464:errorcluster, "Auxiliary Device Details"=→"Auxiliary Device Details":T12, "Mercury Reference Out"=w463:T35)  [unwired: 1 in, 6 out]
        n175 = call-poly <instrlib>:"Configuration (Read).vi"("error in"=w464, "Mercury Reference In"=w463) -> ("error out"=w467:errorcluster, "Serial Number"=→"Aux S/N":string, "Mercury Reference Out"=w466:T35)  [unwired: 1 in, 6 out]
        n176 = call-poly <instrlib>:"Configuration (Read).vi"("error in"=w467, "Mercury Reference In"=w466) -> ("error out"=w469:errorcluster, "Unit"=→"Unit 2":T3, "Min Flow"=→"Min Flow":dbl, "Mercury Reference Out"=w468:T35)  [unwired: 1 in, 5 out]
        n177 = call-poly <instrlib>:"Configuration (Read).vi"("error in"=w469, "Mercury Reference In"=w468) -> ("error out"=w471:errorcluster, "Unit"=→"Unit 3":T3, "Scaling Factor"=→"Scaling Factor":dbl, "Mercury Reference Out"=w470:T35)  [unwired: 1 in, 5 out]
        n178 = call-poly <instrlib>:"Configuration (Read).vi"("error in"=w471, "Mercury Reference In"=w470) -> ("error out"=w439:errorcluster, "Unit"=→"Unit 4":T3, "Temp Err"=→"Temp Err":dbl, "Mercury Reference Out"=w435:T35)  [unwired: 1 in, 5 out]
        n179 = call-poly <instrlib>:"Configuration (Read).vi"("error in"=w439, "Mercury Reference In"=w435) -> ("error out"=w443:errorcluster, "Unit"=→"Unit 5":T3, "Temp V Err"=→"Temp V Err":dbl, "Mercury Reference Out"=w442:T35)  [unwired: 1 in, 5 out]
        n180 = call-poly <instrlib>:"Configuration (Read).vi"("error in"=w443, "Mercury Reference In"=w442) -> ("error out"=w445:errorcluster, "Unit"=→"Unit 6":T3, "Gear"=→"Gear":u32, "Mercury Reference Out"=w444:T35)  [unwired: 1 in, 5 out]
        n181 = call-poly <instrlib>:"Configuration (Read).vi"("error in"=w445, "Mercury Reference In"=w444) -> ("error out"=w453:errorcluster, "Unit"=→"Unit 7":T3, "Speed"=→"Speed":u32, "Mercury Reference Out"=w452:T35)  [unwired: 1 in, 5 out]
        n182 = call-poly <instrlib>:"Signals (Read).vi"("error in"=w453, "Mercury Reference In"=w452) -> ("error out"=w455:errorcluster, "Unit"=→"Unit":T3, "Position"=→"Position":u32, "Mercury Reference Out"=w454:T35)  [unwired: 1 in, 5 out]
        n183 = call-poly <instrlib>:"Signals (Read).vi"("error in"=w455, "Mercury Reference In"=w454) -> ("error out"=w441:errorcluster, "Unit"=→"Unit":T3, "% Open"=→"% Open":dbl)  [unwired: 1 in, 6 out]
        n184 = call <vilib>:"Add State(s) to Queue__JKI_lib_State_Machine.vi"("State(s) in (\"\")"=w478) -> ("States Out"=w479:string)  [unwired: 14 in]
      }
      frame "Mercury: Query ITC: Pressure" {
        # "Pressure"
        n185 = Unbundle By Name(w487) -> ("Mercury ITC Ref"=w484:T35)
        n186 = local read "ITC Devices"() -> (w486:string[])
        n187 = Index Array(array=w486, index=1) -> (element=w483:string)
        n188 = call-poly <instrlib>:"Open.vi"("error in (no error)"=w482, "Device Identifier"=w483, "Mercury Reference In"=w484) -> ("error out"=w490:errorcluster, "Mercury Reference Out"=w491:T35)  [unwired: 7 out]
        n189 = call-poly <instrlib>:"Configuration (Read).vi"("error in"=w490, "Mercury Reference In"=w491) -> ("error out"=w492:errorcluster, "Device Details"=w489:T45, "Mercury Reference Out"=w493:T35)  [unwired: 1 in, 6 out]
        n190 = Unbundle By Name(w489) -> ("Manufacturing"=→"Manufacturing":T8, "Pressure Signals"=→"Pressure Signals":T11)
        n191 = call-poly <instrlib>:"Configuration (Read).vi"("error in"=w492, "Mercury Reference In"=w493) -> ("error out"=w497:errorcluster, "Nickname"=→"Nickname":string, "Mercury Reference Out"=w498:T35)  [unwired: 1 in, 6 out]
        n192 = call-poly <instrlib>:"Signals (Read).vi"("error in"=w497, "Mercury Reference In"=w498) -> ("error out"=w495:errorcluster, "Current"=→"Current":dbl, "Mercury Reference Out"=w496:T35)  [unwired: 1 in, 6 out]
        n193 = call-poly <instrlib>:"Signals (Read).vi"("error in"=w495, "Mercury Reference In"=w496) -> ("error out"=w488:errorcluster, "Voltage"=→"Voltage":dbl)  [unwired: 1 in, 7 out]
        n194 = call <vilib>:"Add State(s) to Queue__JKI_lib_State_Machine.vi"("State(s) in (\"\")"=w501) -> ("States Out"=w502:string)  [unwired: 14 in]
      }
      frame "Mercury: Query IPS: System" {
        # "Your code here.\n(You can make a copy of, or modify, this frame)"
        n195 = Unbundle By Name(w544) -> ("Mercury IPS Ref"=w505:T35)
        n196 = call-poly <instrlib>:"Configuration (Read).vi"("error in"=w510, "Mercury Reference In"=w505) -> ("error out"=w530:errorcluster, "Devices"=→"IPS Devices":string[], "Mercury Reference Out"=w529:T35)  [unwired: 1 in, 6 out]
        n197 = call-poly <instrlib>:"Configuration (Read).vi"("error in"=w530, "Mercury Reference In"=w529) -> ("error out"=w534:errorcluster, "Automatic Dimming"=→"Automatic Dimming 2":string, "Mercury Reference Out"=w533:T35)  [unwired: 1 in, 6 out]
        n198 = call-poly <instrlib>:"Configuration (Read).vi"("error in"=w534, "Mercury Reference In"=w533) -> ("error out"=w531:errorcluster, "Dimming Time"=→"Dimming Time 2":string, "Mercury Reference Out"=w532:T35)  [unwired: 1 in, 6 out]
        n199 = call-poly <instrlib>:"Configuration (Read).vi"("error in"=w531, "Mercury Reference In"=w532) -> ("error out"=w528:errorcluster, "Display Brightness"=→"Display Brightness 2":string, "Mercury Reference Out"=w527:T35)  [unwired: 1 in, 6 out]
        n200 = call-poly <instrlib>:"Configuration (Read).vi"("error in"=w528, "Mercury Reference In"=w527) -> ("error out"=w537:errorcluster, "Date"=→"Date 2":string, "Mercury Reference Out"=w538:T35)  [unwired: 1 in, 6 out]
        n201 = call-poly <instrlib>:"Configuration (Read).vi"("error in"=w537, "Mercury Reference In"=w538) -> ("error out"=w535:errorcluster, "Time"=→"Time 2":string, "Mercury Reference Out"=w536:T35)  [unwired: 1 in, 6 out]
        n202 = call-poly <instrlib>:"Configuration (Read).vi"("error in"=w535, "Mercury Reference In"=w536) -> ("error out"=w509:errorcluster, "time stamp"=→"time stamp 2":timestamp, "Mercury Reference Out"=w506:T35)  [unwired: 1 in, 6 out]
        n203 = call-poly <instrlib>:"Configuration (Read).vi"("error in"=w509, "Mercury Reference In"=w506) -> ("error out"=w511:errorcluster, "Hardware Version"=→"Hardware Version 2":string, "Mercury Reference Out"=w512:T35)  [unwired: 1 in, 6 out]
        n204 = call-poly <instrlib>:"Configuration (Read).vi"("error in"=w511, "Mercury Reference In"=w512) -> ("error out"=w513:errorcluster, "Firmware Version"=→"Firmware Version 2":string, "Mercury Reference Out"=w514:T35)  [unwired: 1 in, 6 out]
        n205 = call-poly <instrlib>:"Configuration (Read).vi"("error in"=w513, "Mercury Reference In"=w514) -> ("error out"=w519:errorcluster, "Serial Number"=→"Serial Number 2":string, "Mercury Reference Out"=w520:T35)  [unwired: 1 in, 6 out]
        n206 = call-poly <instrlib>:"Configuration (Read).vi"("error in"=w519, "Mercury Reference In"=w520) -> ("error out"=w515:errorcluster, "Free Space"=→"Free Space 2":i32, "Mercury Reference Out"=w516:T35)  [unwired: 1 in, 6 out]
        n207 = call-poly <instrlib>:"Configuration (Read).vi"("error in"=w515, "Mercury Reference In"=w516) -> ("error out"=w518:errorcluster, "Mode"=→"String 2":T32, "Mercury Reference Out"=w517:T35)  [unwired: 1 in, 6 out]
        n208 = Get Date/Time In Seconds() -> (seconds since 1Jan1904=w526:timestamp)
        n209 = call-poly <instrlib>:"Configuration (Set).vi"("error in"=w518, "time stamp"=w526, "Mercury Reference In"=w517) -> ("error out"=w508:errorcluster, "Response"=→"Set Date Response 2":T34)  [unwired: 1 in, 6 out]
        n210 = call <vilib>:"Add State(s) to Queue__JKI_lib_State_Machine.vi"("State(s) in (\"\")"=w546) -> ("States Out"=w545:string)  [unwired: 14 in]
      }
      frame "Mercury: Query IPS: LVL" {
        # "level"
        # "Level"
        n211 = Unbundle By Name(w586) -> ("Mercury IPS Ref"=w549:T35)
        n212 = local read "IPS Devices"() -> (w585:string[])
        n213 = Index Array(array=w585, index=0) -> (element=w548:string)
        n214 = call-poly <instrlib>:"Open.vi"("error in (no error)"=w555, "Device Identifier"=w548, "Mercury Reference In"=w549) -> ("error out"=w571:errorcluster, "Mercury Reference Out"=w570:T35)  [unwired: 7 out]
        n215 = call-poly <instrlib>:"Configuration (Read).vi"("error in"=w571, "Mercury Reference In"=w570) -> ("error out"=w576:errorcluster, "LVL Device Settings"=→"LVL Device DetailSettings":T14, "Mercury Reference Out"=w573:T35)  [unwired: 1 in, 6 out]
        n216 = call-poly <instrlib>:"Configuration (Read).vi"("error in"=w576, "Mercury Reference In"=w573) -> ("error out"=w577:errorcluster, "Serial Number"=→"LVL S/N":string, "Mercury Reference Out"=w575:T35)  [unwired: 1 in, 6 out]
        n217 = call-poly <instrlib>:"Configuration (Read).vi"("error in"=w577, "Mercury Reference In"=w575) -> ("error out"=w580:errorcluster, "Resistance Configuration"=→"He Res Config":T19, "Mercury Reference Out"=w579:T35)  [unwired: 1 in, 6 out]
        n218 = call-poly <instrlib>:"Configuration (Read).vi"("error in"=w580, "Mercury Reference In"=w579) -> ("error out"=w582:errorcluster, "Magnitude"=→"LVL P Magnitude":dbl, "Mercury Reference Out"=w581:T35)  [unwired: 1 in, 6 out]
        n219 = call-poly <instrlib>:"Configuration (Read).vi"("error in"=w582, "Mercury Reference In"=w581) -> ("error out"=w554:errorcluster, "Duration"=→"LVL P Duration":dbl, "Mercury Reference Out"=w552:T35)  [unwired: 1 in, 6 out]
        n220 = call-poly <instrlib>:"Configuration (Read).vi"("error in"=w554, "Mercury Reference In"=w552) -> ("error out"=w558:errorcluster, "Freq 100%"=→"N Freq 100%":dbl, "Mercury Reference Out"=w557:T35)  [unwired: 1 in, 6 out]
        n221 = call-poly <instrlib>:"Configuration (Read).vi"("error in"=w558, "Mercury Reference In"=w557) -> ("error out"=w561:errorcluster, "Pulse Period"=→"N Pulse Period":dbl, "Mercury Reference Out"=w560:T35)  [unwired: 1 in, 6 out]
        n222 = call-poly <instrlib>:"Signals (Read).vi"("error in"=w561, "Mercury Reference In"=w560) -> ("error out"=w563:errorcluster, "Resistance"=→"He Resistance":dbl, "Mercury Reference Out"=w562:T35)  [unwired: 1 in, 6 out]
        n223 = call-poly <instrlib>:"Signals (Read).vi"("error in"=w563, "Mercury Reference In"=w562) -> ("error out"=w565:errorcluster, "Level"=→"He Level" →"He LEVEL":dbl, "Mercury Reference Out"=w564:T35)  [unwired: 1 in, 6 out]
        n224 = call-poly <instrlib>:"Signals (Read).vi"("error in"=w565, "Mercury Reference In"=w564) -> ("error out"=w567:errorcluster, "Counter"=→"N Counter":u32, "Mercury Reference Out"=w566:T35)  [unwired: 1 in, 6 out]
        n225 = call-poly <instrlib>:"Signals (Read).vi"("error in"=w567, "Mercury Reference In"=w566) -> ("error out"=w553:errorcluster, "Level"=→"N Level" →"N2 LEVEL":dbl)  [unwired: 1 in, 7 out]
        n226 = call <vilib>:"Add State(s) to Queue__JKI_lib_State_Machine.vi"("State(s) in (\"\")"=w587) -> ("States Out"=w588:string)  [unwired: 14 in]
      }
      frame "Mercury: Query IPS: Temperature" {
        # "temperature"
        n227 = Unbundle By Name(w633) -> ("Mercury IPS Ref"=w594:T35)
        n228 = local read "IPS Devices"() -> (w632:string[])
        n229 = Index Array(array=w632, index=4) -> (element=w595:string)
        n230 = call-poly <instrlib>:"Open.vi"("error in (no error)"=w593, "Device Identifier"=w595, "Mercury Reference In"=w594) -> ("error out"=w620:errorcluster, "Mercury Reference Out"=w615:T35)  [unwired: 7 out]
        n231 = call-poly <instrlib>:"Configuration (Read).vi"("error in"=w620, "Mercury Reference In"=w615) -> ("error out"=w621:errorcluster, "Serial Number"=→"Temp S/N 2":string, "Mercury Reference Out"=w616:T35)  [unwired: 1 in, 6 out]
        n232 = call-poly <instrlib>:"Configuration (Read).vi"("error in"=w621, "Mercury Reference In"=w616) -> ("error out"=w622:errorcluster, "Nickname"=→"T Nickname 2":string, "Mercury Reference Out"=w617:T35)  [unwired: 1 in, 6 out]
        n233 = call-poly <instrlib>:"Configuration (Read).vi"("error in"=w622, "Mercury Reference In"=w617) -> ("error out"=w623:errorcluster, "Unit"=→"Unit 12":T3, "Excitation Magnitude"=→"Excitation Magnitude 2":dbl, "Mercury Reference Out"=w618:T35)  [unwired: 1 in, 5 out]
        n234 = call-poly <instrlib>:"Configuration (Read).vi"("error in"=w623, "Mercury Reference In"=w618) -> ("error out"=w624:errorcluster, "Sensor Type"=→"Sensor Type 2":T41, "Mercury Reference Out"=w619:T35)  [unwired: 1 in, 6 out]
        n235 = call-poly <instrlib>:"Configuration (Read).vi"("error in"=w624, "Mercury Reference In"=w619) -> ("error out"=w597:errorcluster, "Excitation Type"=→"Excitation Type 2":T7, "Mercury Reference Out"=w596:T35)  [unwired: 1 in, 6 out]
        n236 = call-poly <instrlib>:"Configuration (Read).vi"("error in"=w597, "Mercury Reference In"=w596) -> ("error out"=w602:errorcluster, "Unit"=→"H Unit 2":T3, "Hot Limit"=→"Hot Limit 2":dbl, "Mercury Reference Out"=w598:T35)  [unwired: 1 in, 5 out]
        n237 = call-poly <instrlib>:"Configuration (Read).vi"("error in"=w602, "Mercury Reference In"=w598) -> ("error out"=w603:errorcluster, "Unit"=→"C Unit 2":T3, "Cold Limit"=→"Cold Limit 2":dbl, "Mercury Reference Out"=w599:T35)  [unwired: 1 in, 5 out]
        n238 = call-poly <instrlib>:"Signals (Read).vi"("error in"=w603, "Mercury Reference In"=w599) -> ("error out"=w604:errorcluster, "Unit"=→"V Unit 2":T3, "Voltage"=→"Voltage 2":dbl, "Mercury Reference Out"=w600:T35)  [unwired: 1 in, 5 out]
        n239 = call-poly <instrlib>:"Signals (Read).vi"("error in"=w604, "Mercury Reference In"=w600) -> ("error out"=w605:errorcluster, "Unit"=→"T Unit 2":T3, "Temperature"=→"Temperature 2":dbl, "Mercury Reference Out"=w601:T35)  [unwired: 1 in, 5 out]
        n240 = call-poly <instrlib>:"Configuration (Read).vi"("error in"=w605, "Mercury Reference In"=w601) -> ("error out"=w606:errorcluster, "Device Details"=w589:T42)  [unwired: 1 in, 7 out]
        n241 = Unbundle By Name(w589) -> ("Manufacturing"=→"IPS Manufacturing":T8, "Excitation"=→"IPS Excitation":T6, "Calibration"=→"IPS Calibration":T4)
        n242 = call <vilib>:"Add State(s) to Queue__JKI_lib_State_Machine.vi"("State(s) in (\"\")"=w634) -> ("States Out"=w635:string)  [unwired: 14 in]
      }
      frame "Mercury: Query IPS: Magnet" {
        n243 = Unbundle By Name(w674) -> ("Mercury IPS Ref"=w640:T35)
        n244 = call-poly <instrlib>:"Open.vi"("error in (no error)"=w636, "Device Identifier"="Device Identifier", "Mercury Reference In"=w640) -> ("error out"=w659:errorcluster, "Mercury Reference Out"=w658:T35)  [unwired: 7 out]
        n245 = call-poly <instrlib>:"Configuration (Read).vi"("error in"=w659, "Mercury Reference In"=w658) -> ("error out"=w662:errorcluster, "Magnet Device Details"=→"Magnet Device Details":T22, "Mercury Reference Out"=w661:T35)  [unwired: 1 in, 6 out]
        n246 = call-poly <instrlib>:"Configuration (Read).vi"("error in"=w662, "Mercury Reference In"=w661) -> ("error out"=w665:errorcluster, "Serial Number"=→"Mag S/N":string, "Mercury Reference Out"=w664:T35)  [unwired: 1 in, 6 out]
        n247 = call-poly <instrlib>:"Configuration (Read).vi"("error in"=w665, "Mercury Reference In"=w664) -> ("error out"=w668:errorcluster, "Bipolar Output"=→"Bipolar Output":string, "Mercury Reference Out"=w667:T35)  [unwired: 1 in, 6 out]
        n248 = call-poly <instrlib>:"Configuration (Read).vi"("error in"=w668, "Mercury Reference In"=w667) -> ("error out"=w671:errorcluster, "Out Config"=→"Out Config":T50, "Mercury Reference Out"=w670:T35)  [unwired: 1 in, 6 out]
        n249 = call-poly <instrlib>:"Configuration (Read).vi"("error in"=w671, "Mercury Reference In"=w670) -> ("error out"=w642:errorcluster, "Unit"=→"Unit 8":T3, "Current Limit"=→"Current Limit":dbl, "Mercury Reference Out"=w639:T35)  [unwired: 1 in, 5 out]
        n250 = call-poly <instrlib>:"Configuration (Read).vi"("error in"=w642, "Mercury Reference In"=w639) -> ("error out"=w645:errorcluster, "Unit"=→"Unit 9":T3, "AtoB"=→"AtoB":dbl, "Mercury Reference Out"=w644:T35)  [unwired: 1 in, 5 out]
        n251 = call-poly <instrlib>:"Configuration (Read).vi"("error in"=w645, "Mercury Reference In"=w644) -> ("error out"=w648:errorcluster, "Switch Present"=→"Switch Present":string, "Mercury Reference Out"=w647:T35)  [unwired: 1 in, 6 out]
        n252 = call-poly <instrlib>:"Configuration (Read).vi"("error in"=w648, "Mercury Reference In"=w647) -> ("error out"=w653:errorcluster, "Unit"=→"Unit 10":T3, "SW VLIM"=→"SW VLIM":dbl, "Mercury Reference Out"=w652:T35)  [unwired: 1 in, 5 out]
        n253 = call-poly <instrlib>:"Signals (Read).vi"("error in"=w653, "Mercury Reference In"=w652) -> ("error out"=w655:errorcluster, "Unit"=→"Unit 11":T3, "Current Rate"=→"Current Rate":dbl, "Mercury Reference Out"=w654:T35)  [unwired: 1 in, 5 out]
        n254 = call-poly <instrlib>:"Signals (Read).vi"("error in"=w655, "Mercury Reference In"=w654) -> ("error out"=w641:errorcluster, "PSU Act Stat"=→"PSU Act Stat":T51)  [unwired: 1 in, 7 out]
        n255 = call <vilib>:"Add State(s) to Queue__JKI_lib_State_Machine.vi"("State(s) in (\"\")"=w675) -> ("States Out"=w676:string)  [unwired: 14 in]
      }
      frame "---------- Mercury: Idle ----------" {
        n256 = call <vilib>:"Add State(s) to Queue__JKI_lib_State_Machine.vi"("State(s) in (\"\")"=w680) -> ("States Out"=w679:string)  [unwired: 14 in]
      }
      frame "Mercury: Idle" {
        # "#Implemented: Get IPS Magnet Temperature.vi"
        n257 = Unbundle By Name(w684) -> ("LEDs"=w682:bool[], "Mercury IPS Ref"=w701:T35, "Mercury ITC Ref"=w700:T35)
        n258 = Not(x=w682) -> (.not. x?=w681:bool[])
        "LEDs" <- w681
        n259 = disable-structure shown="Enabled" {
          disable-tunnel: w700 -> [w720 _]
          disable-tunnel: w699 -> [w719 w722]
          disable-tunnel: [w706 w722] -> w695
          frame Disabled {
            n260 = local read "ITC Devices"() -> (w717:string[])
            n261 = Index Array(array=w717, index=3) -> (element=w710:string)
            n262 = call-poly <instrlib>:"Open.vi"("error in (no error)"=w719, "Device Identifier"=w710, "Mercury Reference In"=w720) -> ("error out"=w716:errorcluster, "Mercury Reference Out"=w714:T35)  [unwired: 7 out]
            n263 = call-poly <instrlib>:"Signals (Read).vi"("error in"=w716, "Mercury Reference In"=w714) -> ("error out"=w713:errorcluster, "Temperature"=→"LPF Temperature":dbl, "Mercury Reference Out"=w712:T35)  [unwired: 1 in, 6 out]
            n264 = call-poly <instrlib>:"Signals (Read).vi"("error in"=w713, "Mercury Reference In"=w712) -> ("error out"=w709:errorcluster, "Resistance"=→"LPF Resistance":dbl, "Mercury Reference Out"=w708:T35)  [unwired: 1 in, 6 out]
            n265 = call-poly <instrlib>:"Configuration (Set).vi"("error in"=w709, "Excitation Magnitude"=0.0, "Mercury Reference In"=w708) -> ("error out"=w706:errorcluster, "Response"=w705:T34)  [unwired: 5 in, 2 out]
            n266 = call "MercuryStateHistory.vi"("Current State in"=w705) -> ("delimited string"=w704:string)  [unwired: 9 in, 1 out]
            n267 = local write "Magnet Status 2"(w704) -> ()
          }
          frame Enabled {
            w721 = -1.0 ("LPF Temperature")
            n268 = local write "LPF Temperature"(w721) -> ()
            n269 = local write "LPF Resistance"(w721) -> ()
          }
        }
        n270 = local read "IPS Devices"() -> (w698:string[])
        n271 = Index Array(array=w698, index=5) -> (element=w696:string)
        n272 = Bundle By Name(cluster=w684, "LEDs"=w681) -> (w683:T38)
        n273 = call-poly <instrlib>:"Open.vi"("error in (no error)"=w695, "Device Identifier"=w696, "Mercury Reference In"=w701) -> ("error out"=w692:errorcluster, "Mercury Reference Out"=w693:T35)  [unwired: 7 out]
        n274 = call-poly <instrlib>:"Signals (Read).vi"("error in"=w692, "Mercury Reference In"=w693) -> ("error out"=w685:errorcluster, "Temperature"=→"Magnet Temperature":dbl, "Mercury Reference Out"=w694:T35)  [unwired: 1 in, 6 out]
        n275 = call "Read IPS Magnet Temperature.vi"() -> ()  [unwired: 8 in, 4 out]
        n276 = call-poly <instrlib>:"Signals (Read).vi"("error in"=w685, "Mercury Reference In"=w694) -> ("error out"=w688:errorcluster, "Resistance"=→"Magnet Resistance":dbl, "Mercury Reference Out"=w689:T35)  [unwired: 1 in, 6 out]
        n277 = First Call?() -> (First Call?: T/F=w686:bool)
        n278 = case shown="True" w686 {
          tunnel: [w723 w726] -> w687
          tunnel: w689 -> [_ w725]
          tunnel: w688 -> [w723 w724]
          frame False {
          }
          frame True {
            n279 = disable-structure shown="Disabled" {
              disable-tunnel: [w732 _] -> w726
              disable-tunnel: w725 -> [w728 _]
              disable-tunnel: w724 -> [w727 _]
              frame Disabled {
                n280 = call-poly <instrlib>:"Configuration (Set).vi"("error in"=w727, "Excitation Magnitude"=20.0, "Mercury Reference In"=w728) -> ("error out"=w732:errorcluster, "Response"=w730:T34)  [unwired: 5 in, 2 out]
                n281 = call "MercuryStateHistory.vi"("Current State in"=w730) -> ("delimited string"=w729:string)  [unwired: 9 in, 1 out]
                n282 = local write "Magnet Status 2"(w729) -> ()
              }
              frame Enabled {
              }
            }
          }
        }
        n283 = call <vilib>:"Add State(s) to Queue__JKI_lib_State_Machine.vi"("State(s) in (\"\")"=w702) -> ("States Out"=w703:string)  [unwired: 14 in]
      }
      frame "Mercury: IPS: Idle - 1" {
        # "#Implemented: Read IPS Status"
        # "#Implemented: Read IPS Magnet Field"
        # "#Implemented: Read IPS Targets"
        # "#Implemented: Read IPS PSU Field"
        # "#Implemented: Read IPS PSU Current Voltage"
        # "#Implemented: Read IPS Switch Heater"
        # "Magnet"
        # "set switch status"
        n284 = Unbundle By Name(w736) -> ("Mercury IPS Ref"=w739:T35)
        n285 = local read "Device Identifier"() -> (w752:T24)
        n286 = call-poly <instrlib>:"Configuration (Read).vi"("error in"=w767, "Mercury Reference In"=w739) -> ("error out"=w759:errorcluster, "Time"=w762:string, "Mercury Reference Out"=w760:T35)  [unwired: 1 in, 6 out]
        n287 = local write "Time 2"(w762) -> ()
        n288 = call-poly <instrlib>:"Open.vi"("error in (no error)"=w759, "Device Identifier"=w752, "Mercury Reference In"=w760) -> ("error out"=w758:errorcluster, "Mercury Reference Out"=w757:T35)  [unwired: 7 out]
        n289 = call-poly <instrlib>:"Signals (Read).vi"("error in"=w758, "Mercury Reference In"=w757) -> ("error out"=w734:errorcluster, "Switch Heater Status"=w738:string, "Mercury Reference Out"=w733:T35)  [unwired: 1 in, 6 out]
        n290 = call "Read IPS Switch Heater.vi"() -> ()  [unwired: 8 in, 4 out]
        n291 = Equal?(x=w738, y="ON") -> (x = y?=→"SWITCH HEATER":bool)
        n292 = call-poly <instrlib>:"Signals (Read).vi"("error in"=w734, "Mercury Reference In"=w733) -> ("error out"=w766:errorcluster, "Current"=→"Current (A)" →"Current (A)":dbl, "Mercury Reference Out"=w764:T35)  [unwired: 1 in, 6 out]
        n293 = call "Read IPS PSU Current Voltage.vi"() -> ()  [unwired: 8 in, 4 out]
        n294 = call-poly <instrlib>:"Signals (Read).vi"("error in"=w766, "Mercury Reference In"=w764) -> ("error out"=w751:errorcluster, "Voltage"=→"Voltage (V)" →"Voltage (V)":dbl, "Mercury Reference Out"=w750:T35)  [unwired: 1 in, 6 out]
        n295 = call-poly <instrlib>:"Signals (Read).vi"("error in"=w751, "Mercury Reference In"=w750) -> ("error out"=w753:errorcluster, "Field"=→"Power Supply Field (T)":dbl, "Mercury Reference Out"=w756:T35)  [unwired: 1 in, 6 out]
        n296 = call-poly <instrlib>:"Signals (Read).vi"("error in"=w753, "Mercury Reference In"=w756) -> ("error out"=w754:errorcluster, "Target Field Rate"=→"Target Field Rate (T/min)":dbl, "Mercury Reference Out"=w755:T35)  [unwired: 1 in, 6 out]
        n297 = call "Read IPS PSU Targets.vi"() -> ()  [unwired: 8 in, 4 out]
        n298 = call-poly <instrlib>:"Signals (Read).vi"("error in"=w754, "Mercury Reference In"=w755) -> ("error out"=w749:errorcluster, "Target Field"=→"Target Field (T)":dbl, "Mercury Reference Out"=w748:T35)  [unwired: 1 in, 6 out]
        n299 = call-poly <instrlib>:"Signals (Read).vi"("error in"=w749, "Mercury Reference In"=w748) -> ("error out"=w765:errorcluster, "Persistant Field"=→"Magnet Field (T)" →"Magnet Field (T)":dbl, "Mercury Reference Out"=w763:T35)  [unwired: 1 in, 6 out]
        n300 = call "Read IPS PSU Field.vi"() -> ()  [unwired: 9 in, 3 out]
        n301 = call "Read IPS Magnet Field.vi"() -> ()  [unwired: 9 in, 3 out]
        n302 = call-poly <instrlib>:"Signals (Read).vi"("error in"=w765, "Mercury Reference In"=w763) -> ("error out"=w737:errorcluster, "PSU Act Stat"=w740:T51)  [unwired: 1 in, 7 out]
        n303 = local write "PSU Act Stat"(w740) -> ()
        n304 = call "Read IPS Status.vi"() -> ()  [unwired: 9 in, 3 out]
        n305 = case shown="\"RTOZ\"" w740 {
          selector: w740 -> [w770 _ _ _ _]
          tunnel: [w770 "Holding" "Ramping to Setpoint" "Ramping to Zero" "Clamped"] -> w747
          frame Default {
          }
          frame "HOLD" {
          }
          frame "RTOS" {
          }
          frame "RTOZ" {
          }
          frame "CLMP" {
          }
        }
        "Magnet Status" <- w747
        n306 = call <vilib>:"Add State(s) to Queue__JKI_lib_State_Machine.vi"("State(s) in (\"\")"=w768) -> ("States Out"=w769:string)  [unwired: 14 in]
      }
      frame "Mercury: IPS: Idle - 1a" {
        # "#implemented: Read IPS PSU1/2/3 Current Voltage"
        n307 = local read "IPS Devices"() -> (w800:string[])
        n308 = Unbundle By Name(w804) -> ("Mercury IPS Ref"=w803:T35)
        n309 = for {
          tunnel: w800 -> [w808] mode=indexing
          tunnel: [w807] -> w799 mode=indexing
          n310 = Match Pattern(string=w808, regular expression=":PSU") -> (before substring=w807:string)  [unwired: 1 in, 3 out]
        }
        n311 = Index Array(array=w799, index #1=6 ("index")) -> (element #1=w801:string, element #2=w797:string, element #3=w798:string)  [unwired: 2 in]
        n312 = call-poly <instrlib>:"Open.vi"("error in (no error)"=w802, "Device Identifier"=w801, "Mercury Reference In"=w803) -> ("error out"=w779:errorcluster, "Mercury Reference Out"=w783:T35)  [unwired: 7 out]
        n313 = call-poly <instrlib>:"Signals (Read).vi"("error in"=w779, "Mercury Reference In"=w783) -> ("error out"=w785:errorcluster, "Current"=→"M1 Current":dbl, "Mercury Reference Out"=w784:T35)  [unwired: 1 in, 6 out]
        n314 = call-poly <instrlib>:"Signals (Read).vi"("error in"=w785, "Mercury Reference In"=w784) -> ("error out"=w777:errorcluster, "Voltage"=→"M1 Voltage":dbl)  [unwired: 1 in, 7 out]
        n315 = call-poly <instrlib>:"Open.vi"("error in (no error)"=w777, "Device Identifier"=w797, "Mercury Reference In"=w803) -> ("error out"=w780:errorcluster, "Mercury Reference Out"=w782:T35)  [unwired: 7 out]
        n316 = call "Read IPS PSU1 Current Voltage.vi"() -> ()  [unwired: 8 in, 4 out]
        n317 = call-poly <instrlib>:"Signals (Read).vi"("error in"=w780, "Mercury Reference In"=w782) -> ("error out"=w788:errorcluster, "Current"=→"M2 Current":dbl, "Mercury Reference Out"=w786:T35)  [unwired: 1 in, 6 out]
        n318 = call "Read IPS PSU2 Current Voltage.vi"() -> ()  [unwired: 8 in, 4 out]
        n319 = call-poly <instrlib>:"Signals (Read).vi"("error in"=w788, "Mercury Reference In"=w786) -> ("error out"=w775:errorcluster, "Voltage"=→"M2 Voltage":dbl)  [unwired: 1 in, 7 out]
        n320 = call "Read IPS PSU3 Current Voltage.vi"() -> ()  [unwired: 8 in, 4 out]
        n321 = call-poly <instrlib>:"Open.vi"("error in (no error)"=w775, "Device Identifier"=w798, "Mercury Reference In"=w803) -> ("error out"=w778:errorcluster, "Mercury Reference Out"=w781:T35)  [unwired: 7 out]
        n322 = call-poly <instrlib>:"Signals (Read).vi"("error in"=w778, "Mercury Reference In"=w781) -> ("error out"=w789:errorcluster, "Current"=→"M3 Current":dbl, "Mercury Reference Out"=w787:T35)  [unwired: 1 in, 6 out]
        n323 = call-poly <instrlib>:"Signals (Read).vi"("error in"=w789, "Mercury Reference In"=w787) -> ("error out"=w776:errorcluster, "Voltage"=→"M3 Voltage":dbl)  [unwired: 1 in, 7 out]
        n324 = call <vilib>:"Add State(s) to Queue__JKI_lib_State_Machine.vi"("State(s) in (\"\")"=w805) -> ("States Out"=w806:string)  [unwired: 14 in]
      }
      frame "Mercury: IPS: Idle - 2" {
        w812 = enum16{"write", "read"}."write" ("Function")
        # "#implemented: Read IPS Level"
        # "set all of these things"
        n325 = Unbundle By Name(w820) -> ("Mercury IPS Ref"=w832:T35)
        n326 = local read "IPS Devices"() -> (w857:string[])
        n327 = Index Array(array=w857, index=0) -> (element=w856:string)
        n328 = call-poly <instrlib>:"Open.vi"("error in (no error)"=w853, "Device Identifier"=w856, "Mercury Reference In"=w832) -> ("error out"=w859:errorcluster, "Mercury Reference Out"=w860:T35)  [unwired: 7 out]
        n329 = call-poly <instrlib>:"Signals (Read).vi"("error in"=w859, "Mercury Reference In"=w860) -> ("error out"=w861:errorcluster, "Level"=w844:dbl, "Mercury Reference Out"=w862:T35)  [unwired: 1 in, 6 out]
        "He LVL Chart" <- w844
        n330 = call "Read IPS Level.vi"() -> ()  [unwired: 8 in, 4 out]
        n331 = Greater?(x=w844, y=20.0) -> (0:w851:bool)
        n332 = Greater?(x=w844, y=50.0) -> (0:w852:bool)
        n333 = call-poly <instrlib>:"Signals (Read).vi"("error in"=w861, "Mercury Reference In"=w862) -> ("error out"=w810:errorcluster, "Level"=w843:dbl)  [unwired: 1 in, 7 out]
        "N2 LVL Chart" <- w843
        n334 = case shown="False" w851 {
          tunnel: [w870 u32 6618880] -> w841
          tunnel: w852 -> [w871 _]
          frame False {
            n335 = case shown="False" w871 {
              tunnel: [u32 16711680 u32 16776704] -> w870
              frame False {
              }
              frame True {
              }
            }
          }
          frame True {
          }
        }
        n336 = local write "He LEVEL"(w844) -> ()
        n337 = property on="He LVL Chart" class="Slide (strict)"("Fill Color"=w841) -> ()  [unwired: 2 in, 2 out]
        n338 = property on="He LEVEL" class="DigNum (strict)"("NumText.TextColor"=w841) -> ()  [unwired: 2 in, 2 out]
        n339 = local write "N2 LEVEL"(w843) -> ()
        n340 = local read "Target Field Rate (T/min)"() -> (w837:dbl)
        n341 = local read "Power Supply Field (T)"() -> (w835:dbl)
        n342 = Greater?(x=w843, y=20.0) -> (0:w846:bool)
        n343 = Greater?(x=w843, y=50.0) -> (0:w845:bool)
        n344 = local read "Magnet Field (T)"() -> (w834:dbl)
        n345 = local read "Target Field (T)"() -> (w836:dbl)
        n346 = local read "Current (A)"() -> (w839:dbl)
        n347 = local read "Voltage (V)"() -> (w838:dbl)
        n348 = local read "SWITCH HEATER"() -> (w821:bool)
        n349 = local read "PSU Act Stat"() -> (w813:string)
        n350 = case shown="True" w846 {
          tunnel: [w865 u32 6618880] -> w842
          tunnel: w845 -> [w866 _]
          frame False {
            n351 = case shown="False" w866 {
              tunnel: [u32 16711680 u32 16776704] -> w865
              frame False {
              }
              frame True {
              }
            }
          }
          frame True {
          }
        }
        n352 = local read "Magnet Temperature"() -> (w830:dbl)
        n353 = property on="N2 LVL Chart" class="Slide (strict)"("Fill Color"=w842) -> ()  [unwired: 2 in, 2 out]
        n354 = property on="N2 LEVEL" class="DigNum (strict)"("NumText.TextColor"=w842) -> ()  [unwired: 2 in, 2 out]
        n355 = Bundle By Name(cluster=T29 {"Magnet Field"=0.0, "PS Field"=0.0, "Target Field"=0.0, "Target Field Rate"=0.0, "Voltage"=0.0, "Current"=0.0, "Switch"=FALSE, "Mercury State"=""} ("Status"), "Magnet Field"=w834, "PS Field"=w835, "Target Field"=w836, "Target Field Rate"=w837, "Voltage"=w838, "Current"=w839, "Switch"=w821, "Mercury State"=w813) -> (w818:T29)
        n356 = local read "Magnet Resistance"() -> (w831:dbl)
        n357 = Select(t="ON", s=w821, f="OFF") -> (s? t:f=w811:string)
        n358 = local read "M1 Current"() -> (w829:dbl)
        n359 = local read "M1 Voltage"() -> (w828:dbl)
        n360 = local read "M2 Current"() -> (w827:dbl)
        n361 = local read "M2 Voltage"() -> (w826:dbl)
        n362 = local read "M3 Current"() -> (w825:dbl)
        n363 = local read "M3 Voltage"() -> (w824:dbl)
        n364 = call "FGV_PSP - Mercury Status.vi"("error in"=w810, "Function"=w812, "Status"=w818) -> ("error out"=w817:errorcluster)  [unwired: 3 in, 1 out]
        n365 = Bundle(cluster=T30 {"Magnet Field"=0.0, "PS Field"=0.0, "Target Field"=0.0, "Target Field Rate"=0.0, "Voltage"=0.0, "Current"=0.0}, "Magnet Field"=w834, "PS Field"=w835, "Target Field"=w836, "Target Field Rate"=w837, "Voltage"=w838, "Current"=w839) -> (w840:T30)
        n366 = call "FGV_PSP - Mercury Action Status.vi"("error in"=w817, "Function"=w812, "Mercury Status"=w813) -> ("error out"=w816:errorcluster)  [unwired: 3 in, 1 out]
        n367 = Cluster To Array(cluster=w840) -> (array=w815:dbl[])
        n368 = Build Array(w829, w828, w827, w826, w825, w824) -> (w814:dbl[])
        n369 = Build Array (concatenate)(w815, w843, w844, w830, w831, w814) -> (w855:dbl[])
        n370 = Build Array(w813, w811) -> (w854:string[])
        n371 = call "1820_IPS_to_DSC.vi"("str"=w854, "dbl"=w855) -> ()  [unwired: 2 in]
        n372 = call <vilib>:"Add State(s) to Queue__JKI_lib_State_Machine.vi"("State(s) in (\"\")"=w863) -> ("States Out"=w864:string)  [unwired: 14 in]
      }
      frame "Mercury: IPS: Idle - 3" {
        n373 = case shown="True" "Enable RS232 Panel" {
          tunnel: w877 -> [w881 w883]
          tunnel: [w881 w882] -> w876
          frame False {
          }
          frame True {
            n374 = call "Oxford_MNK_Omega_Sign.vi"("error in (no error)"=w883) -> ("error out"=w882:errorcluster)  [unwired: 10 in]
          }
        }
        n375 = call <vilib>:"Add State(s) to Queue__JKI_lib_State_Machine.vi"("State(s) in (\"\")"=w879) -> ("States Out"=w880:string)  [unwired: 14 in]
      }
      frame "Mercury: ITC: Idle" {
        # "#implemented: Read ITC LPF Needle Valve"
        # "#implemented: Read ITC LPF Pressure"
        # "needle valve motor"
        # "pressure sensor"
        n376 = Unbundle By Name(w905) -> ("Mercury ITC Ref"=w889:T35)
        n377 = local read "ITC Devices"() -> (w904:string[])
        n378 = call "Read ITC LPF Pressure.vi"() -> ()  [unwired: 9 in, 3 out]
        n379 = Index Array(array=w904, index=1) -> (element=w902:string)
        n380 = call-poly <instrlib>:"Open.vi"("error in (no error)"=w884, "Device Identifier"=w902, "Mercury Reference In"=w889) -> ("error out"=w901:errorcluster, "Mercury Reference Out"=w900:T35)  [unwired: 7 out]
        n381 = call-poly <instrlib>:"Configuration (Read).vi"("error in"=w901, "Mercury Reference In"=w900) -> ("error out"=w898:errorcluster, "Device Details"=w899:T45)  [unwired: 1 in, 7 out]
        n382 = local read "ITC Devices"() -> (w896:string[])
        n383 = Unbundle By Name(w899) -> ("Pressure Signals.Pressure"=w888:string)
        n384 = Index Array(array=w896, index=0) -> (element=w895:string)
        n385 = Fract/Exp String To Number(string=w888) -> (number=w887:dbl)  [unwired: 3 in, 1 out]
        "LPF Pressure" <- w887
        n386 = call-poly <instrlib>:"Open.vi"("error in (no error)"=w898, "Device Identifier"=w895, "Mercury Reference In"=w889) -> ("error out"=w894:errorcluster, "Mercury Reference Out"=w893:T35)  [unwired: 7 out]
        n387 = call "Read ITC LPF Needle Valve.vi"() -> ()  [unwired: 9 in, 3 out]
        n388 = local read "LPF Temperature"() -> (w886:dbl)
        n389 = local read "LPF Resistance"() -> (w885:dbl)
        n390 = call-poly <instrlib>:"Signals (Read).vi"("error in"=w894, "Mercury Reference In"=w893) -> ("error out"=w890:errorcluster, "% Open"=w891:dbl)  [unwired: 1 in, 7 out]
        "LPF Needle Valve (%)" <- w891
        n391 = Build Array(w886, w887, w891, w885) -> (w892:dbl[])
        n392 = call "1820_ITC_to_DSC.vi"("dbl"=w892) -> ()  [unwired: 3 in]
        n393 = call <vilib>:"Add State(s) to Queue__JKI_lib_State_Machine.vi"("State(s) in (\"\")"=w906) -> ("States Out"=w907:string)  [unwired: 14 in]
      }
      frame "Mercury: Empty" {
        n394 = call <vilib>:"Add State(s) to Queue__JKI_lib_State_Machine.vi"("State(s) in (\"\")"=w910) -> ("States Out"=w911:string)  [unwired: 14 in]
      }
      frame "---------- Mercury: Action ----------" {
        n395 = call <vilib>:"Add State(s) to Queue__JKI_lib_State_Machine.vi"("State(s) in (\"\")"=w915) -> ("States Out"=w914:string)  [unwired: 14 in]
      }
      frame "Mercury: Remote" {
        w930 = "\n"
        w923 = enum16{"write", "read"}."read" ("Function")
        n396 = call "FGV_PSP - Mercury Remote.vi"("error in"=w953, "Function"=enum16{"write", "read"}."write", "Remote"=TRUE ("Mercury FGV.Remote")) -> ("error out"=w952:errorcluster)  [unwired: 3 in, 1 out]
        n397 = call "FGV_PSP - Mercury Actions.vi"("error in"=w952, "Function"=w923) -> ("error out"=w928:errorcluster, "Actions"=w929:T31)  [unwired: 4 in]
        n398 = call "FGV_PSP - Mercury Targets.vi"("error in"=w928, "Function"=w923) -> ("error out"=w924:errorcluster, "Targets"=w927:T52)  [unwired: 4 in]
        n399 = Unbundle By Name(w927) -> ("Field (T)"=w926:dbl, "Field Rate (T/min)"=w925:dbl)
        n400 = Unbundle By Name(w929) -> ("Hold"=w922:bool, "Clamp"=w917:bool, "To Set"=w918:bool, "To Zero"=w919:bool, "PS Heat"=w920:bool, "Lambda"=w916:bool, "Send to IPS"=w921:bool)
        n401 = local read "Send to IPS"() -> (w944:bool)
        n402 = local read "Lambda"() -> (w943:bool)
        n403 = local read "To Zero"() -> (w941:bool)
        n404 = local read "PS Heat"() -> (w942:bool)
        n405 = local read "Clamp"() -> (w939:bool)
        n406 = local read "To Set"() -> (w940:bool)
        n407 = local read "Hold"() -> (w938:bool)
        n408 = local write "Send to IPS"(w921) -> ()
        n409 = local write "Lambda"(w916) -> ()
        n410 = local write "To Zero"(w919) -> ()
        n411 = local write "PS Heat"(w920) -> ()
        n412 = local write "Clamp"(w917) -> ()
        n413 = Not Equal?(x=w938, y=w922) -> (x != y?=w951:bool)
        n414 = Not Equal?(x=w939, y=w917) -> (x != y?=w950:bool)
        n415 = Not Equal?(x=w940, y=w918) -> (x != y?=w949:bool)
        n416 = local write "To Set"(w918) -> ()
        n417 = Not Equal?(x=w941, y=w919) -> (x != y?=w948:bool)
        n418 = Not Equal?(x=w942, y=w920) -> (x != y?=w947:bool)
        n419 = Not Equal?(x=w943, y=w916) -> (x != y?=w946:bool)
        n420 = Not Equal?(x=w944, y=w921) -> (x != y?=w945:bool)
        n421 = local write "Hold"(w922) -> ()
        n422 = local write "Target Field (T)"(w926) -> ()
        n423 = local write "Target Rate (T/min)"(w925) -> ()
        n424 = case shown="True" w951 {
          tunnel: ["" ("State(s) in Front (\"\")") "Mercury: Hold" ("State(s) in Front (\"\")")] -> w937
          frame False {
          }
          frame True {
          }
        }
        n425 = case shown="True" w949 {
          tunnel: ["" ("State(s) in Front (\"\")") "Mercury: To Set" ("State(s) in Front (\"\")")] -> w935
          frame False {
          }
          frame True {
          }
        }
        n426 = case shown="True" w947 {
          tunnel: ["" ("State(s) in Front (\"\")") "Mercury: PS Heat" ("State(s) in Front (\"\")")] -> w933
          frame False {
          }
          frame True {
          }
        }
        n427 = case shown="True" w946 {
          tunnel: ["" ("State(s) in Front (\"\")") "Mercury: Lambda" ("State(s) in Front (\"\")")] -> w932
          frame False {
          }
          frame True {
          }
        }
        n428 = case shown="True" w945 {
          tunnel: ["" ("State(s) in Front (\"\")") "Mercury: Send To IPS" ("State(s) in Front (\"\")")] -> w931
          frame False {
          }
          frame True {
          }
        }
        n429 = case shown="True" w950 {
          tunnel: ["" ("State(s) in Front (\"\")") "Mercury: Clamp" ("State(s) in Front (\"\")")] -> w936
          frame False {
          }
          frame True {
          }
        }
        n430 = case shown="True" w948 {
          tunnel: ["" ("State(s) in Front (\"\")") "Mercury: To Zero" ("State(s) in Front (\"\")")] -> w934
          frame False {
          }
          frame True {
          }
        }
        n431 = Concatenate Strings(w937, w930, w936, w930, w935, w930, w934, w930, w933, w930, w932, w930, w931, w930) -> (w957:string)
        n432 = call <vilib>:"Add State(s) to Queue__JKI_lib_State_Machine.vi"("State(s) in Front (\"\")"=w957, "State(s) in (\"\")"=w958) -> ("States Out"=w959:string)  [unwired: 13 in]
      }
      frame "Mercury: Hold" {
        w976 = FALSE ("Hold")
        w974 = T51 "HOLD" ("PSU Act Stat")
        # "#implemented: Set IPS Action"
        # "log action to remote variable server"
        # "keep history of commands"
        # "log reply to DSC"
        # "action set"
        # "open connection"
        n433 = Unbundle By Name(w981) -> ("Mercury IPS Ref"=w988:T35)
        n434 = local read "Device Identifier"() -> (w989:T24)
        n435 = call-poly <instrlib>:"Open.vi"("error in (no error)"=w986, "Device Identifier"=w989, "Mercury Reference In"=w988) -> ("error out"=w990:errorcluster, "Mercury Reference Out"=w987:T35)  [unwired: 7 out]
        n436 = call-poly <instrlib>:"Signals (Set).vi"("error in"=w990, "PSU Act Stat"=w974, "Mercury Reference In"=w987) -> ("error out"=w984:errorcluster, "Response"=w982:T34)  [unwired: 1 in, 6 out]
        n437 = call "IPSReplytoDSC.vi"("error in (no error)"=w984, "Response"=w982) -> ("error out"=w977:errorcluster)  [unwired: 9 in]
        n438 = call "Set IPS Action.vi"("PSU Act Stat"=w974) -> ()  [unwired: 8 in, 3 out]
        n439 = call "MercuryStateHistory.vi"("initialize?"=FALSE, "Current State in"=w982) -> ("delimited string"=w985:string)  [unwired: 8 in, 1 out]
        n440 = local write "Magnet Status 2"(w985) -> ()
        n441 = local write "Hold"(w976) -> ()
        n442 = Bundle By Name(cluster=T31 {"Hold"=FALSE, "Clamp"=FALSE, "To Set"=FALSE, "To Zero"=FALSE, "Send to IPS"=FALSE, "PS Heat"=FALSE, "Lambda"=FALSE} ("Actions"), "Hold"=w976) -> (w979:T31)
        n443 = call "FGV_PSP - Mercury Actions.vi"("error in"=w977, "Function"=enum16{"write", "read"}."write", "Actions"=w979) -> ("error out"=w975:errorcluster)  [unwired: 3 in, 1 out]
        n444 = call <vilib>:"Add State(s) to Queue__JKI_lib_State_Machine.vi"("State(s) in (\"\")"=w991) -> ("States Out"=w992:string)  [unwired: 14 in]
      }
      frame "Mercury: Heater Current" {
        n445 = Unbundle By Name(w1018) -> ("Mercury IPS Ref"=w1021:T35)
        n446 = local read "Device Identifier"() -> (w1022:T24)
        n447 = call-poly <instrlib>:"Open.vi"("error in (no error)"=w1015, "Device Identifier"=w1022, "Mercury Reference In"=w1021) -> ("Mercury Reference Out"=w1014:T35)  [unwired: 8 out]
        n448 = call-poly <instrlib>:"Configuration (Set).vi"("error in"=w1015, "Password"="abc123", "Mode"=T32 "ENG", "Mercury Reference In"=w1014) -> ("error out"=w1012:errorcluster, "Response"=w1013:T34, "Mercury Reference Out"=w1010:T35)  [unwired: 4 in, 1 out]
        n449 = call "IPSReplytoDSC.vi"("error in (no error)"=w1012, "Response"=w1013) -> ("error out"=w1008:errorcluster)  [unwired: 9 in]
        n450 = call "MercuryStateHistory.vi"("initialize?"=FALSE, "Current State in"=w1013) -> ("delimited string"=w1020:string)  [unwired: 8 in, 1 out]
        n451 = local write "Magnet Status 2"(w1020) -> ()
        n452 = call <userlib>:"Wait (ms)__ogtk.vi"("error in (no error)"=w1008, "milliseconds to wait"=u32 1000) -> ("error out"=w1009:errorcluster)  [unwired: 8 in, 1 out]
        n453 = call-poly <instrlib>:"Configuration (Set).vi"("error in"=w1009, "Swh Htr Current"="Swh Htr Current (mA)", "Mercury Reference In"=w1010) -> ("error out"=w1004:errorcluster, "Response"=w994:T34, "Mercury Reference Out"=w999:T35)  [unwired: 5 in, 1 out]
        n454 = call "IPSReplytoDSC.vi"("error in (no error)"=w1004, "Response"=w994) -> ("error out"=w1003:errorcluster)  [unwired: 9 in]
        n455 = call "MercuryStateHistory.vi"("initialize?"=FALSE, "Current State in"=w994) -> ("delimited string"=w997:string)  [unwired: 8 in, 1 out]
        n456 = local write "Magnet Status 2"(w997) -> ()
        n457 = call <userlib>:"Wait (ms)__ogtk.vi"("error in (no error)"=w1003, "milliseconds to wait"=u32 1000) -> ("error out"=w1002:errorcluster)  [unwired: 8 in, 1 out]
        n458 = call-poly <instrlib>:"Configuration (Set).vi"("error in"=w1002, "Mode"=T32 "NORM", "Mercury Reference In"=w999) -> ("error out"=w1001:errorcluster, "Response"=w993:T34)  [unwired: 5 in, 2 out]
        n459 = call "IPSReplytoDSC.vi"("error in (no error)"=w1001, "Response"=w993) -> ("error out"=w1000:errorcluster)  [unwired: 9 in]
        n460 = call "MercuryStateHistory.vi"("initialize?"=FALSE, "Current State in"=w993) -> ("delimited string"=w996:string)  [unwired: 8 in, 1 out]
        n461 = local write "Magnet Status 2"(w996) -> ()
        n462 = call <vilib>:"Add State(s) to Queue__JKI_lib_State_Machine.vi"("State(s) in (\"\")"=w1023) -> ("States Out"=w1024:string)  [unwired: 14 in]
      }
      frame "Mercury: Clamp" {
        w1026 = FALSE
        w1025 = T51 "CLMP" ("PSU Act Stat")
        # "#implemented: Set IPS Action"
        n463 = Unbundle By Name(w1032) -> ("Mercury IPS Ref"=w1038:T35)
        n464 = local read "Device Identifier"() -> (w1041:T24)
        n465 = call-poly <instrlib>:"Open.vi"("error in (no error)"=w1037, "Device Identifier"=w1041, "Mercury Reference In"=w1038) -> ("error out"=w1040:errorcluster, "Mercury Reference Out"=w1039:T35)  [unwired: 7 out]
        n466 = call-poly <instrlib>:"Signals (Set).vi"("error in"=w1040, "PSU Act Stat"=w1025, "Mercury Reference In"=w1039) -> ("error out"=w1036:errorcluster, "Response"=w1033:T34)  [unwired: 1 in, 6 out]
        n467 = call "Set IPS Action.vi"("PSU Act Stat"=w1025) -> ()  [unwired: 8 in, 3 out]
        n468 = call "IPSReplytoDSC.vi"("error in (no error)"=w1036, "Response"=w1033) -> ("error out"=w1028:errorcluster)  [unwired: 9 in]
        n469 = call "MercuryStateHistory.vi"("initialize?"=FALSE, "Current State in"=w1033) -> ("delimited string"=w1034:string)  [unwired: 8 in, 1 out]
        n470 = local write "Magnet Status 2"(w1034) -> ()
        n471 = local write "Clamp"(w1026) -> ()
        n472 = Bundle By Name(cluster=T31 {"Hold"=FALSE, "Clamp"=FALSE, "To Set"=FALSE, "To Zero"=FALSE, "Send to IPS"=FALSE, "PS Heat"=FALSE, "Lambda"=FALSE} ("Actions"), "Clamp"=w1026) -> (w1030:T31)
        n473 = call "FGV_PSP - Mercury Actions.vi"("error in"=w1028, "Function"=enum16{"write", "read"}."write", "Actions"=w1030) -> ("error out"=w1027:errorcluster)  [unwired: 3 in, 1 out]
        n474 = call <vilib>:"Add State(s) to Queue__JKI_lib_State_Machine.vi"("State(s) in (\"\")"=w1042) -> ("States Out"=w1043:string)  [unwired: 14 in]
      }
      frame "Mercury: To Set" {
        w1047 = FALSE
        w1044 = T51 "RTOS" ("PSU Act Stat")
        # "#implemented: Set IPS Action"
        n475 = Unbundle By Name(w1051) -> ("Mercury IPS Ref"=w1058:T35)
        n476 = local read "Device Identifier"() -> (w1057:T24)
        n477 = call-poly <instrlib>:"Open.vi"("error in (no error)"=w1056, "Device Identifier"=w1057, "Mercury Reference In"=w1058) -> ("error out"=w1059:errorcluster, "Mercury Reference Out"=w1060:T35)  [unwired: 7 out]
        n478 = call-poly <instrlib>:"Signals (Set).vi"("error in"=w1059, "PSU Act Stat"=w1044, "Mercury Reference In"=w1060) -> ("error out"=w1054:errorcluster, "Response"=w1053:T34)  [unwired: 1 in, 6 out]
        n479 = call "Set IPS Action.vi"("PSU Act Stat"=w1044) -> ()  [unwired: 8 in, 3 out]
        n480 = call "IPSReplytoDSC.vi"("error in (no error)"=w1054, "Response"=w1053) -> ("error out"=w1046:errorcluster)  [unwired: 9 in]
        n481 = call "MercuryStateHistory.vi"("initialize?"=FALSE, "Current State in"=w1053) -> ("delimited string"=w1055:string)  [unwired: 8 in, 1 out]
        n482 = local write "Magnet Status 2"(w1055) -> ()
        n483 = local write "To Set"(w1047) -> ()
        n484 = Bundle By Name(cluster=T31 {"Hold"=FALSE, "Clamp"=FALSE, "To Set"=FALSE, "To Zero"=FALSE, "Send to IPS"=FALSE, "PS Heat"=FALSE, "Lambda"=FALSE} ("Actions"), "To Set"=w1047) -> (w1049:T31)
        n485 = call "FGV_PSP - Mercury Actions.vi"("error in"=w1046, "Function"=enum16{"write", "read"}."write", "Actions"=w1049) -> ("error out"=w1045:errorcluster)  [unwired: 3 in, 1 out]
        n486 = call <vilib>:"Add State(s) to Queue__JKI_lib_State_Machine.vi"("State(s) in (\"\")"=w1061) -> ("States Out"=w1062:string)  [unwired: 14 in]
      }
      frame "Mercury: To Zero" {
        w1066 = FALSE
        w1063 = T51 "RTOZ" ("PSU Act Stat")
        # "#implemented: Set IPS Action"
        n487 = Unbundle By Name(w1070) -> ("Mercury IPS Ref"=w1077:T35)
        n488 = local read "Device Identifier"() -> (w1076:T24)
        n489 = call-poly <instrlib>:"Open.vi"("error in (no error)"=w1075, "Device Identifier"=w1076, "Mercury Reference In"=w1077) -> ("error out"=w1078:errorcluster, "Mercury Reference Out"=w1079:T35)  [unwired: 7 out]
        n490 = call-poly <instrlib>:"Signals (Set).vi"("error in"=w1078, "PSU Act Stat"=w1063, "Mercury Reference In"=w1079) -> ("error out"=w1073:errorcluster, "Response"=w1071:T34)  [unwired: 1 in, 6 out]
        n491 = call "Set IPS Action.vi"("PSU Act Stat"=w1063) -> ()  [unwired: 8 in, 3 out]
        n492 = call "IPSReplytoDSC.vi"("error in (no error)"=w1073, "Response"=w1071) -> ("error out"=w1065:errorcluster)  [unwired: 9 in]
        n493 = call "MercuryStateHistory.vi"("initialize?"=FALSE, "Current State in"=w1071) -> ("delimited string"=w1074:string)  [unwired: 8 in, 1 out]
        n494 = local write "Magnet Status 2"(w1074) -> ()
        n495 = local write "To Zero"(w1066) -> ()
        n496 = Bundle By Name(cluster=T31 {"Hold"=FALSE, "Clamp"=FALSE, "To Set"=FALSE, "To Zero"=FALSE, "Send to IPS"=FALSE, "PS Heat"=FALSE, "Lambda"=FALSE} ("Actions"), "To Zero"=w1066) -> (w1068:T31)
        n497 = call "FGV_PSP - Mercury Actions.vi"("error in"=w1065, "Function"=enum16{"write", "read"}."write", "Actions"=w1068) -> ("error out"=w1064:errorcluster)  [unwired: 3 in, 1 out]
        n498 = call <vilib>:"Add State(s) to Queue__JKI_lib_State_Machine.vi"("State(s) in (\"\")"=w1080) -> ("States Out"=w1081:string)  [unwired: 14 in]
      }
      frame "Mercury: PS Heat" {
        # "#implement: Set IPS Switch Heater"
        # "set switch action to F because we\nalready changed it"
        # "set the status of the switch\nT = ON\nF = OFF"
        n499 = local read "Device Identifier"() -> (w1093:T24)
        n500 = Unbundle By Name(w1088) -> ("Mercury IPS Ref"=w1094:T35)
        n501 = call-poly <instrlib>:"Open.vi"("error in (no error)"=w1090, "Device Identifier"=w1093, "Mercury Reference In"=w1094) -> ("error out"=w1091:errorcluster, "Mercury Reference Out"=w1092:T35)  [unwired: 7 out]
        n502 = call-poly <instrlib>:"Signals (Read).vi"("error in"=w1091, "Mercury Reference In"=w1092) -> ("error out"=w1096:errorcluster, "Current"=w1085:dbl, "Mercury Reference Out"=w1095:T35)  [unwired: 1 in, 6 out]
        n503 = call-poly <instrlib>:"Signals (Read).vi"("error in"=w1096, "Mercury Reference In"=w1095) -> ("error out"=w1082:errorcluster, "Persistant Current"=w1084:dbl, "Mercury Reference Out"=w1097:T35)  [unwired: 1 in, 6 out]
        n504 = Subtract(x=w1084, y=w1085) -> (x-y=w1098:dbl)
        n505 = Absolute Value(x=w1098) -> (abs(x)=w1099:dbl)
        n506 = Less?(x=w1099, y=0.1) -> (x < y?=w1101:bool)
        n507 = case shown="False" w1101 {
          selector: w1101 -> [_ w1106]
          tunnel: [w1105 w1106] -> w1083
          frame False {
            n508 = Two Button Dialog(message="The magnet current is more\nthan 0.1A different to the\nPSU output current.  It is not\nadvisable to switch on the\nswitch heater unless these\ncurrents are equal!") -> (T button?=w1105:bool)  [unwired: 2 out]
          }
          frame True {
          }
        }
        n509 = call "Set IPS Switch Heater.vi"() -> ()  [unwired: 9 in, 3 out]
        n510 = local read "PS Heat"() -> (w1087:bool)
        n511 = Or(x=w1083, y=w1087) -> (x .or. y?=w1086:bool)
        n512 = case shown="True" w1086 {
          tunnel: w1097 -> [_ w1136]
          tunnel: w1082 -> [w1107 w1135]
          tunnel: [w1107 w1122] -> w1089
          frame False {
          }
          frame True {
            w1108 = FALSE ("PS Heat")
            n513 = Get Date/Time In Seconds() -> (seconds since 1Jan1904=→"PS ON/OFF":timestamp)
            n514 = call-poly <instrlib>:"Signals (Read).vi"("error in"=w1135, "Mercury Reference In"=w1136) -> ("error out"=w1137:errorcluster, "Switch Heater Status"=w1118:string, "Mercury Reference Out"=w1119:T35)  [unwired: 1 in, 6 out]
            n515 = Equal?(x=w1118, y="ON") -> (x = y?=w1116:bool)
            n516 = call <userlib>:"Wait (ms)__ogtk.vi"("error in (no error)"=w1137, "milliseconds to wait"=u32 100 ("millisecond multiple")) -> ("error out"=w1134:errorcluster)  [unwired: 8 in, 1 out]
            n517 = Select(t=T33 "OFF" ("Set Switch Heater"), s=w1116, f=T33 "ON" ("Set Switch Heater")) -> (s? t:f=w1111:T33)
            n518 = call-poly <instrlib>:"Signals (Set).vi"("error in"=w1134, "Set Switch Heater"=w1111, "Mercury Reference In"=w1119) -> ("error out"=w1128:errorcluster, "Response"=w1126:T34, "Mercury Reference Out"=w1115:T35)  [unwired: 1 in, 5 out]
            n519 = call "MercuryStateHistory.vi"("initialize?"=FALSE, "Current State in"=w1126) -> ("delimited string"=w1130:string)  [unwired: 8 in, 1 out]
            n520 = local write "Magnet Status 2"(w1130) -> ()
            n521 = call "IPSReplytoDSC.vi"("error in (no error)"=w1128, "Response"=w1126) -> ("error out"=w1125:errorcluster)  [unwired: 9 in]
            n522 = while {
              tunnel: [w1145] -> w1120
              tunnel: w1125 -> [w1143]
              tunnel: w1111 -> [w1141]
              tunnel: w1115 -> [w1139]
              tunnel: [w1138] -> w1110
              stop <- w1140 stop-if-true
              # "wait here while setting"
              n523 = call-poly <instrlib>:"Signals (Read).vi"("error in"=w1143, "Mercury Reference In"=w1139) -> ("error out"=w1145:errorcluster, "Switch Heater Status"=w1142:string)  [unwired: 1 in, 7 out]
              n524 = Equal?(x=w1142, y=w1141) -> (x = y?=w1140:bool)
              n525 = Equal?(x=w1142, y="ON") -> (x = y?=w1138:bool)
            }
            n526 = Bundle By Name(cluster=T29 {"Magnet Field"=0.0, "PS Field"=0.0, "Target Field"=0.0, "Target Field Rate"=0.0, "Voltage"=0.0, "Current"=0.0, "Switch"=FALSE, "Mercury State"=""} ("Status"), "Switch"=w1110) -> (w1113:T29)
            n527 = call "FGV_PSP - Mercury Status.vi"("error in"=w1120, "Function"=enum16{"write", "read"}."write", "Status"=w1113) -> ("error out"=w1121:errorcluster)  [unwired: 3 in, 1 out]
            n528 = local write "PS Heat"(w1108) -> ()
            n529 = Bundle By Name(cluster=T31 {"Hold"=FALSE, "Clamp"=FALSE, "To Set"=FALSE, "To Zero"=FALSE, "Send to IPS"=FALSE, "PS Heat"=FALSE, "Lambda"=FALSE} ("Actions"), "PS Heat"=w1108) -> (w1123:T31)
            n530 = call "FGV_PSP - Mercury Actions.vi"("error in"=w1121, "Function"=enum16{"write", "read"}."write", "Actions"=w1123) -> ("error out"=w1122:errorcluster)  [unwired: 3 in, 1 out]
          }
        }
        n531 = call <vilib>:"Add State(s) to Queue__JKI_lib_State_Machine.vi"("State(s) in (\"\")"=w1102) -> ("States Out"=w1103:string)  [unwired: 14 in]
      }
      frame "Mercury: Send To IPS" {
        w1149 = FALSE
        # "#implemented: Set IPS Targets"
        n532 = local read "Device Identifier"() -> (w1168:T24)
        n533 = Unbundle By Name(w1155) -> ("Mercury IPS Ref"=w1167:T35)
        n534 = call-poly <instrlib>:"Open.vi"("error in (no error)"=w1165, "Device Identifier"=w1168, "Mercury Reference In"=w1167) -> ("error out"=w1169:errorcluster, "Mercury Reference Out"=w1166:T35)  [unwired: 7 out]
        n535 = call-poly <instrlib>:"Signals (Set).vi"("error in"=w1169, "Target Field Rate"="Target Rate (T/min)", "Mercury Reference In"=w1166) -> ("error out"=w1163:errorcluster, "Response"=w1161:T34, "Mercury Reference Out"=w1154:T35)  [unwired: 2 in, 4 out]
        n536 = call "Set IPS PSU Targets.vi"("Target Field Rate (T/min)"="Target Rate (T/min)", "Target Field (T)"="Target Field (T)") -> ()  [unwired: 7 in, 3 out]
        n537 = call "MercuryStateHistory.vi"("initialize?"=FALSE, "Current State in"=w1161) -> ("delimited string"=w1157:string)  [unwired: 8 in, 1 out]
        n538 = call "IPSReplytoDSC.vi"("error in (no error)"=w1163, "Response"=w1161) -> ("error out"=w1162:errorcluster)  [unwired: 9 in]
        n539 = local write "Magnet Status 2"(w1157) -> ()
        n540 = call-poly <instrlib>:"Signals (Set).vi"("error in"=w1162, "Target Field"="Target Field (T)", "Mercury Reference In"=w1154) -> ("error out"=w1164:errorcluster, "Response"=w1156:T34)  [unwired: 2 in, 5 out]
        n541 = local write "Send to IPS"(w1149) -> ()
        n542 = call "IPSReplytoDSC.vi"("error in (no error)"=w1164, "Response"=w1156) -> ("error out"=w1150:errorcluster)  [unwired: 9 in]
        n543 = call "MercuryStateHistory.vi"("initialize?"=FALSE, "Current State in"=w1156) -> ("delimited string"=w1158:string)  [unwired: 8 in, 1 out]
        n544 = local write "Magnet Status 2"(w1158) -> ()
        n545 = Bundle By Name(cluster=T31 {"Hold"=FALSE, "Clamp"=FALSE, "To Set"=FALSE, "To Zero"=FALSE, "Send to IPS"=FALSE, "PS Heat"=FALSE, "Lambda"=FALSE} ("Actions"), "Send to IPS"=w1149) -> (w1152:T31)
        n546 = call "FGV_PSP - Mercury Actions.vi"("error in"=w1150, "Function"=enum16{"write", "read"}."write", "Actions"=w1152) -> ("error out"=w1148:errorcluster)  [unwired: 3 in, 1 out]
        n547 = call <vilib>:"Add State(s) to Queue__JKI_lib_State_Machine.vi"("State(s) in (\"\")"=w1170) -> ("States Out"=w1171:string)  [unwired: 14 in]
      }
      frame "Mercury: Lambda" {
        # "#implemented: Set ITC LPF State"
        # "Lambda device"
        # "AUX\nPRES\nHTR\nTEMP"
        n548 = Unbundle By Name(w1181) -> ("Mercury ITC Ref"=w1190:T35)
        n549 = local read "Lambda"() -> (w1176:bool)
        n550 = call-poly <instrlib>:"Open.vi"("error in (no error)"=w1182, "Device Identifier"="lambda:LPC", "Mercury Reference In"=w1190) -> ("error out"=w1189:errorcluster, "Mercury Reference Out"=w1188:T35)  [unwired: 7 out]
        n551 = Select(t="ON" ("Sweep Mode"), s=w1176, f="OFF" ("Sweep Mode")) -> (s? t:f=w1172:string)
        n552 = case shown="False" w1176 {
          frame False {
            n553 = disable-structure shown="Disabled" {
              frame Disabled {
                n554 = property on="Close Needle Valve" class="Bool (strict)"("Val(Sgnl)"=TRUE ("Value (Signaling)")) -> ()  [unwired: 2 in, 2 out]
              }
              frame Enabled {
              }
            }
          }
          frame True {
          }
        }
        n555 = case shown="False" w1176 {
          frame False {
            n556 = local write "LPF ON"(timestamp(0 s since 1904-01-01) ("LPF ON")) -> ()
          }
          frame True {
            n557 = Get Date/Time In Seconds() -> (seconds since 1Jan1904=w1195:timestamp)
            n558 = local write "LPF ON"(w1195) -> ()
          }
        }
        n559 = call-poly <instrlib>:"Configuration (Set).vi"("error in"=w1189, "Lambda Auto"=w1172, "Mercury Reference In"=w1188) -> ("error out"=w1186:errorcluster, "Response"=w1185:T34)  [unwired: 5 in, 2 out]
        n560 = call "Set ITC LPF State.vi"("LPF State"=w1172) -> ()  [unwired: 8 in, 3 out]
        n561 = call "ITCReplytoDSC.vi"("error in (no error)"=w1186, "Response"=w1185) -> ("error out"=w1177:errorcluster)  [unwired: 9 in]
        n562 = call "MercuryStateHistory.vi"("initialize?"=FALSE, "Current State in"=w1185) -> ("delimited string"=w1183:string)  [unwired: 8 in, 1 out]
        n563 = local write "Magnet Status 2"(w1183) -> ()
        n564 = Bundle By Name(cluster=T31 {"Hold"=FALSE, "Clamp"=FALSE, "To Set"=FALSE, "To Zero"=FALSE, "Send to IPS"=FALSE, "PS Heat"=FALSE, "Lambda"=FALSE} ("Actions"), "Lambda"=w1176) -> (w1179:T31)
        n565 = call "FGV_PSP - Mercury Actions.vi"("error in"=w1177, "Function"=enum16{"write", "read"}."write", "Actions"=w1179) -> ("error out"=w1175:errorcluster)  [unwired: 3 in, 1 out]
        n566 = call <vilib>:"Add State(s) to Queue__JKI_lib_State_Machine.vi"("State(s) in (\"\")"=w1191) -> ("States Out"=w1192:string)  [unwired: 14 in]
      }
      frame "Mercury: Fast/Slow Fill" {
        # "#implemented: Set IPS Fill Mode"
        # "He level sensor"
        n567 = local read "IPS Devices"() -> (w1209:string[])
        n568 = Unbundle By Name(w1197) -> ("Mercury IPS Ref"=w1211:T35)
        n569 = local read "Fast/Slow Fill"() -> (w1198:bool)
        n570 = Index Array(array=w1209, index=0) -> (element=w1206:string)
        n571 = call-poly <instrlib>:"Open.vi"("error in (no error)"=w1200, "Device Identifier"=w1206, "Mercury Reference In"=w1211) -> ("error out"=w1207:errorcluster, "Mercury Reference Out"=w1208:T35)  [unwired: 7 out]
        n572 = Select(t="OFF" ("Temperature setpoint"), s=w1198, f="ON" ("Temperature setpoint")) -> (s? t:f=w1196:string)
        n573 = call "Set IPS Fill Mode.vi"("Fill Mode"=w1196) -> ()  [unwired: 8 in, 3 out]
        n574 = call-poly <instrlib>:"Configuration (Set).vi"("error in"=w1207, "Delay"=w1196, "Mercury Reference In"=w1208) -> ("error out"=w1202:errorcluster, "Response"=w1201:T34)  [unwired: 5 in, 2 out]
        n575 = call "IPSReplytoDSC.vi"("error in (no error)"=w1202, "Response"=w1201) -> ("error out"=w1199:errorcluster)  [unwired: 9 in]
        n576 = call "MercuryStateHistory.vi"("Current State in"=w1201) -> ("delimited string"=w1203:string)  [unwired: 9 in, 1 out]
        n577 = local write "Magnet Status 2"(w1203) -> ()
        n578 = call <vilib>:"Add State(s) to Queue__JKI_lib_State_Machine.vi"("State(s) in (\"\")"=w1212) -> ("States Out"=w1213:string)  [unwired: 14 in]
      }
      frame "Mercury: Needle Valve" {
        # "#implemented: Set ITC LPF Needle Valve"
        n579 = Unbundle By Name(w1218) -> ("Mercury ITC Ref"=w1215:T35)
        n580 = Build Array("Close Needle Valve", "Open Needle Valve") -> (w1226:bool[])
        n581 = call-poly <instrlib>:"Open.vi"("error in (no error)"=w1216, "Device Identifier"="lambda:LPC", "Mercury Reference In"=w1215) -> ("error out"=w1225:errorcluster, "Mercury Reference Out"=w1224:T35)  [unwired: 7 out]
        n582 = Boolean Array To Number(Boolean array=w1226) -> (number=w1223:u32)
        n583 = call "Set ITC LPF Needle Valve.vi"("Percentage Open (%)"="Percentage Open") -> ()  [unwired: 8 in, 3 out]
        n584 = case shown="1" w1223 {
          tunnel: w1225 -> [w1234 w1239 w1246]
          tunnel: w1224 -> [_ w1240 w1245]
          tunnel: [w1234 w1238 w1244] -> w1220
          tunnel: [T34 "" ("Response") w1237 w1243] -> w1219
          tunnel: [FALSE ("Close Needle Valve") FALSE ("Close Needle Valve") FALSE ("Close Needle Valve")] -> w1222
          tunnel: "Percentage Open" -> [_ _ w1241]
          frame 0, Default {
          }
          frame 1 {
            n585 = call-poly <instrlib>:"Configuration (Set).vi"("error in"=w1239, "Percentage Open"=0.0, "Mercury Reference In"=w1240) -> ("error out"=w1238:errorcluster, "Response"=w1237:T34)  [unwired: 5 in, 2 out]
          }
          frame 2 {
            n586 = call-poly <instrlib>:"Configuration (Set).vi"("error in"=w1246, "Percentage Open"=w1241, "Mercury Reference In"=w1245) -> ("error out"=w1244:errorcluster, "Response"=w1243:T34)  [unwired: 5 in, 2 out]
          }
        }
        n587 = local write "Close Needle Valve"(w1222) -> ()
        n588 = local write "Open Needle Valve"(w1222) -> ()
        n589 = call "ITCReplytoDSC.vi"("error in (no error)"=w1220, "Response"=w1219) -> ("error out"=w1217:errorcluster)  [unwired: 9 in]
        n590 = call "MercuryStateHistory.vi"("Current State in"=w1219) -> ("delimited string"=w1221:string)  [unwired: 9 in, 1 out]
        n591 = local write "Magnet Status 2"(w1221) -> ()
        n592 = call <vilib>:"Add State(s) to Queue__JKI_lib_State_Machine.vi"("State(s) in (\"\")"=w1230) -> ("States Out"=w1231:string)  [unwired: 14 in]
      }
    }
  }
  n593 = disable-structure shown="Enabled" {
    frame Disabled {
      (unwired) FALSE
      n594 = call-poly <instrlib>:"Configuration (Read).vi"() -> ()  [unwired: 3 in, 9 out]
      n595 = disable-structure shown="Disabled" {
        frame Disabled {
          n596 = property on="Fast/Slow Fill" class="Bool (strict)" props=["Val(Sgnl)"]() -> ()  [unwired: 3 in, 2 out]
        }
        frame Enabled {
        }
      }
      n597 = local read "PS Heat"() -> ()  [unwired: 1 in]
      n598 = local read "Lambda"() -> ()  [unwired: 1 in]
      n599 = call-poly <instrlib>:"Signals (Read).vi"() -> ()  [unwired: 3 in, 9 out]
    }
    frame Enabled {
    }
  }
